vi "BIMS_Collector.vi"() -> ()   [LabVIEW 2015]
doc: "This program is currently beta software. It is designed to address the data requirements defined primarily by the DHB Ballistic Test Report.\n\nThe general operation of this program is based on the Ballistics Version 2005 application developed internally by DuPont as a research tool for the Spruance Plant Ballistics Lab in Richmond, VA.\n\nPlease note that the original trigger control logic was modified and no longer depends on a safety interlock system to enable operation of a ballistic test.\n\nDuPont makes no warranties and assumes no liabilities in connection with any use of this program."
uses:
  DataSource.ctl
  shotsArr.ctl
  Shot Record.ctl
  Collector State.ctl
  <vilib>/Utility/error.llb/DialogType.ctl
  <vilib>/registry/registry.llb/Registry RtKey.ctl
  <vilib>/DAQmx/read.llb/DAQmx Read (Counter DBL 1Chan 1Samp).vi
  BIMS_Collector Globals.vi
  <vilib>/Utility/config.llb/Write Key (String).vi
  <vilib>/addons/database/Connection.llb/DB Tools Open Connec (Path).vi
  <vilib>/addons/database/Connection.llb/Conn Execute.vi
  <vilib>/addons/database/Recordset.llb/Rec Destroy - Connection.vi
  <vilib>/DAQmx/miscellaneous.llb/DAQmx Fill In Error Info.vi
  <vilib>/addons/database/NI_Database_API.lvlib
  <vilib>/Utility/config.llb/NI_LVConfig.lvlib
  <vilib>/Utility/file.llb/Write To Spreadsheet File (string).vi
panel:
  in  "diagPageVisible":bool
  in  "runtimeMenusVisible":bool=TRUE
  out "loadStatus":string
  out "Loading":u16(ring)
  in  "RESET All":bool
  out "ConfigName":string
  out "TimeNow":string
  in  "EXIT":bool
  in  "mainTabCntrl":enum32{"Setup", "Measure", "History", "System"}(tab)=enum."System"
  in  "SampleEntryTabCntrl":enum32{"Environment", "Sample"}(tab)
  in  "ThreatDetails":u16(ring) caption="Detail"
  in  "ThreatGroups":u16(ring) caption="Group" items=["", "RCC", "FSP", "44 Magnum", "0.22 Caliber", "0.380 Caliber", "0.38 Caliber", "9mm Luger", "40 S&W", "0.357 MAG", "0.44 Expp Mag", ".44 SWC Gas Checked", ".44 SJHP", ".357 SIG", "7.62 AP", "7.62 Comum", "5.56 AP", "5.56 Comum", "0.44 Rem Mag"]
  in  "PowderTypes":u16(ring) caption="Type" items=["", "CBC 236", "CBC 210", "CBC 220", "CBC 216", "CBC 207", "CBC PCL 504", "CBC 102"]
  in  "Ballisticians":u16(ring) caption="Laboratorists" items=["", "Gustavo M Rubio", "Manoel Machado", "Outros (others)", "Renato Dantas"]
  in  "Recorders":u16(ring) caption="Recorder"
  in  "Shooters":u16(ring) caption="Shooter" items=["", "Manoel C. Machado                                 ", "Gustavo M Rubio                                   ", "Assef Maluf                                       "]
  in  "Methods":u16(ring) caption="Method" items=["", "V50", "NIJ 0101.04", "NIJ 0101.06", "NIJ 0108.01", "Helmets", "Others"]
  in  "RoomT":sgl caption="Temperature (° C)" format="%.1f"
  in  "RoomHum":sgl caption="Humidity (%)" min=0 max=100 format="%.1f"
  in  "SampleBackings":u16(ring)=3 caption="Type" items=["", "Clay", "Roma Clay", "Corfix Clay", "Dim Clay"]
  in  "clayCalArray":i16[](array[numeric])=[0, 0, 0, 0, 0] caption="Calibration (mm)" min=0 max=99 format="%02.0f"
  out "clayAverage":sgl caption="Clay Average (mm)" format="%#.1f"
  in  "clayTemp":sgl caption="Clay Temp (° F)" format="%.1f"
  out "threatDetails":T1 caption="Description"
  in  "SampleClamping":u16(ring) caption="Clamping" items=["", "elástic with Velcro", "screws", "rubber tube", "anti spall ", "box against fragments"]
  in  "Sample SubTabCntrl":T2(tab)
  in  "SampleID":string caption="Sample ID"
  in  "SampleDimensions":u16(ring) caption="Dimensions" items=["", "40 x 40", "50 x 50", "P", "M", "G", "GG", "Car Part", "Indefinite"]
  in  "ModelMfrs":u16(ring) caption="Manufacturer" items=["DuPont Experimental"]
  in  "SampleTypes":u16(ring) caption="Sample Type" items=["", "Aramid", "Glass", "Steel", "Ceramic", "Panel", "Body Armor", "Car Parts", "Quality Control", "Helmets", "Shield", "Other"]
  in  "Submitters":u16(ring) caption="Submitter" items=["", "Ana P Viegas", "Julio Tabegna", "Priscila Akiti", "Ariana Bottura", "Carlos Magno", "Rodrigo Gomez", "Angela C Vargas", "Manoel Machado", "Others", "Marcelo Fonseca", "Rosa Buono", "Mayara Guimarães", "Katia Hamada", "Lucas Loureiro"]
  in  "ProjectID":string caption="Project ID"
  in  "BackLayers":i32 caption="# of Layers" min=0 max=99 step=5
  in  "FrontLayers":i32 caption="# of Layers" min=0 max=99 step=5
  in  "BackLayer":u16(ring) caption="Back Layer" items=["", "PC", "Steel", "PE Foam", "Ghost", "ceramic plate", "Others"]
  in  "FrontLayer":u16(ring) caption="Front Layer" items=["", "PC", "Steel", "PE Foam", "Ghost", "ceramic plate", "Others"]
  out "totalNumLayers":i32 caption="Total # of Layers" min=0 max=100 step=5
  out "totalBAW":sgl caption="Total BAW (psf)" format="%.2f"
  in  "LayerTabControl":enum32{"1", "2", "3", "4", "5", "6"}(tab) caption="Inner Layers"
  out "fab1_totalWt":sgl caption="Fab1 Wt" min=0 max=99 step=5 format="%.2f"
  out "SampleAttribs_1":T3 caption="fabricAttribs_1"
  in  "Layer_1":T4 caption="Fabric #1" {"plyNum" min=0}
  in  "SampleStyle_1":u16(ring) items=["", "S 5200 GR", "S 623 GR", "S 758 Prepeg", "S363 GR", "S363 WR", "S436 GR", "S436 WR", "S704 GR", "S704 WR", "S706WRH", "S708 GR", "S708 WR", "S720", "S720 GR", "S720 WR", "S724 GR", "S729 GR", "S729 WR", "S731 GR", "S731 WR", "S745 BKT", "S745 BKT 20", "S745 GR", "S745 H", "S745 WR", "S745GR-1", "S754 GR", "S778 GR", "S778 WR", "S779GR", "S779WR", "XF", "XP1000"]
  in  "Mfr_1":u16(ring) caption="vendor" items=["", "AGP", "Assef Maluf", "DuPont", "DuPont Cooper River", "DuPont do Brasil", "TEADIT", "TestBob1"]
  in  "layerStitch_1":u16(ring) caption="Stitch" items=["", "1-inch quilt", "2-inch quilt", "Corners Bartack", "Corners", "Custom (Panel)", "Custom (Vest)", "Diamond", "Edge", "n/a", "Normal"]
  out "fab2_totalWt":sgl caption="Fab2 Wt" min=0 max=99 step=5 format="%.2f"
  out "SampleAttribs_2":T3 caption="fabricAttribs_2"
  in  "Layer_2":T4 caption="Fabric #2" {"plyNum" min=0}
  in  "SampleStyle_2":u16(ring)
  in  "Mfr_2":u16(ring) caption="vendor" items=["", "AGP", "Assef Maluf", "DuPont", "DuPont Cooper River", "DuPont do Brasil", "TEADIT", "TestBob1"]
  in  "layerStitch_2":u16(ring) caption="Stitch" items=["", "1-inch quilt", "2-inch quilt", "Corners Bartack", "Corners", "Custom (Panel)", "Custom (Vest)", "Diamond", "Edge", "n/a", "Normal"]
  out "fab3_totalWt":sgl caption="Fab3 Wt" min=0 max=99 step=5 format="%.2f"
  out "SampleAttribs_3":T3 caption="fabricAttribs_3"
  in  "Layer_3":T4 caption="Fabric #3" {"plyNum" min=0}
  in  "SampleStyle_3":u16(ring)
  in  "Mfr_3":u16(ring) caption="vendor" items=["", "AGP", "Assef Maluf", "DuPont", "DuPont Cooper River", "DuPont do Brasil", "TEADIT", "TestBob1"]
  in  "layerStitch_3":u16(ring) caption="Stitch" items=["", "1-inch quilt", "2-inch quilt", "Corners Bartack", "Corners", "Custom (Panel)", "Custom (Vest)", "Diamond", "Edge", "n/a", "Normal"]
  out "fab4_totalWt":sgl caption="Fab4 Wt" min=0 max=99 step=5 format="%.2f"
  out "SampleAttribs_4":T3 caption="fabricAttribs_4"
  in  "Layer_4":T4 caption="Fabric #4" {"plyNum" min=0}
  in  "SampleStyle_4":u16(ring)
  in  "Mfr_4":u16(ring) caption="vendor" items=["", "AGP", "Assef Maluf", "DuPont", "DuPont Cooper River", "DuPont do Brasil", "TEADIT", "TestBob1"]
  in  "layerStitch_4":u16(ring) caption="Stitch" items=["", "1-inch quilt", "2-inch quilt", "Corners Bartack", "Corners", "Custom (Panel)", "Custom (Vest)", "Diamond", "Edge", "n/a", "Normal"]
  out "fab5_totalWt":sgl caption="Fab5 Wt" min=0 max=99 step=5 format="%.2f"
  out "SampleAttribs_5":T3 caption="fabricAttribs_5"
  in  "Layer_5":T4 caption="Fabric #5" {"plyNum" min=0}
  in  "SampleStyle_5":u16(ring)
  in  "Mfr_5":u16(ring) caption="vendor" items=["", "AGP", "Assef Maluf", "DuPont", "DuPont Cooper River", "DuPont do Brasil", "TEADIT", "TestBob1"]
  in  "layerStitch_5":u16(ring) caption="Stitch" items=["", "1-inch quilt", "2-inch quilt", "Corners Bartack", "Corners", "Custom (Panel)", "Custom (Vest)", "Diamond", "Edge", "n/a", "Normal"]
  out "fab6_totalWt":sgl caption="Fab6 Wt" min=0 max=99 step=5 format="%.2f"
  out "SampleAttribs_6":T3 caption="fabricAttribs_6"
  in  "Layer_6":T4 caption="Fabric #6" {"plyNum" min=0}
  in  "SampleStyle_6":u16(ring)
  in  "Mfr_6":u16(ring) caption="vendor" items=["", "AGP", "Assef Maluf", "DuPont", "DuPont Cooper River", "DuPont do Brasil", "TEADIT", "TestBob1"]
  in  "layerStitch_6":u16(ring) caption="Stitch" items=["", "1-inch quilt", "2-inch quilt", "Corners Bartack", "Corners", "Custom (Panel)", "Custom (Vest)", "Diamond", "Edge", "n/a", "Normal"]
  in  "SampleCoverings":u16(ring) caption="Sample Covering" items=["None", "RipStop", "Plastic bag", "Other"]
  in  "Assemblers":u16(ring) caption="Technician" items=["", "Gustavo M Rubio", "Lucas Loureiro", "Manoel Machado", "Assef Maluf", "Client", "Tecidos Especiales", "Others"]
  in  "Thickness":dbl caption="Thickness (mm)" format="%.3f"
  in  "totalSampleWt":sgl caption="Total Weight (g)" format="%.3f"
  in  "Comments":string caption="Remarks (optional):"
  in  "TestConditions":u16(ring) caption="Sample Condition" items=["", "Dry", "Wet", "T & H Controlled", "After Tumbling", "Heated", "Cooled"]
  in  "shotsTabCntrl":T5(tab)
  in  "2ndScreen":bool=TRUE caption="Enabled"
  out "cntDn":i32
  in  "Frag Rod":sgl format="%.1f"
  in  "Drag Corrected":bool=TRUE
  out "Impact/speed":sgl caption="Chronograph 1" min=0 max=10000 step=0.1 format="%.1f"
  out "residual/speed":sgl caption="Residual" min=0 max=10000 step=0.1 format="%.1f"
  in  "MeasVelScrnSet1":sgl caption="Set #1" min=0 max=10000 step=0.1 format="%.1f"
  in  "Current/shotstatus":u16(ring) caption="Penetration" items=["Partial", "Complete"]
  in  "Current/residual/speed":sgl caption="Residual Set" min=0 max=10000 step=0.1 format="%.1f"
  in  "shotTimestamp":string caption="Date/Time"
  in  "MeasVelScrnSet2":sgl caption="Set #2" min=0 max=1000000 step=0.1 format="%.1f"
  out "%_Difference":sgl caption="% Vel Diff" format="%.3f"
  in  "backdepth":sgl caption="BF Depth"
  out "Redundant/speed":sgl caption="Chronograph 2" min=0 max=10000 step=0.1 format="%.1f"
  out "Current/avg/speed":sgl caption="Average" min=0 max=1000000 step=0.1 format="%.1f"
  out "Avg/speed":sgl caption="Average" min=0 max=10000 step=0.1 format="%.1f"
  out "DC_ factor":sgl=1.0 caption="DC Factor" format="%.4f"
  in  "Barrel Temp":sgl format="%.1f"
  in  "Shot Description":string caption="Description (optional)"
  in  "Powder Loading":sgl caption="Powder Load" min=0 max=100 step=0.1 format="%.3f"
  in  "Shot Angle":u16 max=90 step=1
  out "Projectile Mass":sgl caption="Projectile Mass (grains)" min=0 step=1
  in  "N.I.J":u16(ring) items=["n/a", "PASS", "FAIL"]
  in  "addShot":bool caption="RANGE SETUP must be selected before shots can be added."
  in  "loadingUnits":enum32{"grams", "grains"}(radio)
  out "instruct_addShot":string="RANGE SETUP and THREAT must be selected before shots can be added."
  out "Set#1 Separation":sgl=1.0 caption="Outer" format="%.2f"
  out "Set#2 Separation":sgl=1.0 caption="Inner" format="%.2f"
  out "ARMED":bool caption="Armed"
  in  "commercialReport":bool caption="Report"
  out "velSTDEV":sgl caption="Standard Deviation" min=0 max=10000 step=1 format="%.1f"
  out "saveReq":string="Number of layers in sample ply specification and number of shots in shots table must be greater than 0 to enable saving."
  out "Table of Shots":string[][](table) caption="Shot Table"
  in  "MC Listbox of Shots":i32(listbox)
  in  "saveShots":bool
  in  "clearShots":bool
  out "highPartial":i32 caption="High Partial" min=0 max=10000 step=1
  out "lowComplete":i32 caption="Low Complete" min=0 max=10000 step=1
  out "rangeOfResults":i32 caption="Range of Results" min=0 max=10000 step=1
  out "zmr 2":sgl caption="ZMR" format="%.1f"
  out "computed_V50":sgl caption="V50  (m/s)" format="%.1f"
  out "Pairs":i16 min=0 max=100 step=1
  in  "reportV50":bool caption="Report"
  in  "maxDev":sgl=10.0 caption="Max Deviation (m/s)" min=0 max=100 format="%.1f"
  in  "undoLastShot":bool
  in  "reportType":enum32{"V50", "NIJ"}(radio)
  in  "language":enum16{"Spanish", "Portuguese", "English"}(ring)
  in  "deleteShot":bool
  in  "nextShot":bool
  in  "shotsArr":T6 {"Frag Rod" format="%.1f"; "UncorrectedAvgVel_PB" format="%.1f"; "UncorrectedRed_PB" format="%.1f"; "strikeVel_PB" format="%.1f"; "velLoss_PB" format="%.1f"; "avgVel_PB" format="%.1f"; "Redundant_Velocity" format="%.1f"; "Energy Loss (J)" format="%.3e"; "Projectile Mass" min=0 step=1 format="%.4f"; "Corrected residual" format="%.2f"; "Uncorrected Residual" format="%.1f"; "Corrected Impact" format="%.2f"; "Uncorrected Impact" format="%.1f"; "Shot Angle" max=90 step=1; "SHOT STATUS" items=["Partial", "Complete"]; "IMPACT VELOCITY" min=0 max=10000 step=0.1 format="%.1f"; "Barrel Temperature" format="%.1f"; "Powder Loading" format="%.4f"; "RESIDUAL  VELOCITY" min=0 max=10000 step=0.1 format="%.1f"}
  out "velProfile":cluster{dbl, dbl}[](graph) caption="Shot Velocity Measurement Profile"
  out "velCompProf":cluster{"vStrike":dbl, "vA":dbl} caption="Velocity in fps\n(computed)"
  out "velMeasProf":T8 caption="Velocity in fps\n(measured)"
  out "relativeTime":cluster{"ts2":dbl, "ts3":dbl, "ts1":dbl} caption="Relative time\n(microsec)"
  out "displacement":T9={"ds_v2"=6.75, "ds2"=5.0833, "ds_vB"=4.9167, "ds3"=4.75, "ds_vAvg"=6.9167, "ds_v1"=7.0833, "ds1"=8.75, "ds_vA"=8.9167, "ds0"=9.0833} caption="Distance from\ntarget (ft)" {"ds0" format="%_4g"; "ds_vA" format="%_4g"; "ds1" format="%_4g"; "ds_v1" format="%_4g"; "ds_vAvg" format="%_4g"; "ds3" format="%_4g"; "ds_vB" format="%#_4g"; "ds2" format="%#_4g"; "ds_v2" format="%_4g"}
  out "arrIDC":dbl[](array[numeric]) caption="Instantaneous Drag Coefficient"
  in  "rangeSetup":u16(ring)=1 caption="Range Dimensions" items=["Short (small frag)", "Standard (handgun)", "Long (rifle)"]
  out "mid_to_targ_dist":sgl=5.0 caption="Mid To Target (ft)"
  in  "historyTabCntrl":enum32{"Powder Loading", "Panel Search"}(tab)=enum."Panel Search"
  in  "Threat.freeTxt":string caption="Threat"
  in  "Powder.freeTxt":string caption="Powder"
  in  "QueryLoad":bool
  in  "lkupEndDate":timestamp caption="End Date" format="%<%x>T"
  in  "lkupStartDate":timestamp caption="Begin Date" format="%<%x>T"
  out "Vel.vs.Loading":cluster{dbl[], dbl[]}(graph)
  out "v50_table":string[][](table)
  in  "maxRecs":u16=1001 caption="Max # of SHOT Records" min=1 max=10000 step=100
  out "ActualNumRecs":i32=1001 caption="Actual # Returned"
  in  "appendPrjs":bool caption="merge projects"
  in  "prjAll":bool
  in  "prjV50Rpt":bool
  in  "prjSelect":bool[](array[boolean])
  in  "ProjectID_0":u16(ring) caption="Project ID"
  in  "ThreatSize_0":u16(ring) caption="Threat Size" items=["", "2", "4", "16", "17", "33", "40", "44", "55", "61", "85", "95", "124", "125", "138", "147", "158", "180", "240"]
  in  "panelSearch":bool
  in  "Mfr_0":u16(ring) caption="Manufacturer" items=["", "AGP", "Assef Maluf", "DuPont", "DuPont Cooper River", "DuPont do Brasil", "TEADIT", "TestBob1"]
  in  "SampleStyle_0":u16(ring) caption="Sample Style"
  in  "srchParams":T10={"maxPanels"=1001, "lkupPanelStartDate"=timestamp(0 s since 1904-01-01), "lkupPanelEndDate"=timestamp(3552315047.0950403 s since 1904-01-01)} {"lkupPanelEndDate" format="%<%x>T"; "lkupPanelStartDate" format="%<%x>T"; "maxPanels" min=1 max=10000 step=100}
  out "actualNumPanels":i32 caption="Actual # Returned"
  out "pastPanels":string[][](table)
  in  "Record #":i32=1 min=0 max=3199
  in  "reportV50_History":bool
  out "SampleAttribs_0":T11 caption="fabricAttribs_1"
  in  "Requestors_0":u16(ring) caption="Submitter" items=["", "Ana P Viegas", "Angela C Vargas", "Ariana Bottura", "Carlos Magno", "Julio Tabegna", "Katia Hamada", "Lucas Loureiro", "Manoel Machado", "Marcelo Fonseca", "Mayara Guimarães", "Others", "Priscila Akiti", "Rodrigo Gomez", "Rosa Buono"]
  in  "aboutTabCntrl":T12(tab)
  in  "RefreshMetadata":bool
  out "lastShot":i32 caption="Shot"
  out "lastSamp":i32 caption="Sample"
  in  "PublishNewRecords":bool
  in  "btnScrnSets":bool caption="Update Screen Sets"
  in  "screenSet_1":sgl caption="Outer" format="%.2f"
  in  "screenSet_2":sgl caption="Inner" format="%.2f"
  in  "internal":enum32{"ctr", "deploy", "misc"}(tab)=enum."misc"
  out "taskCtr1":refnum<k21>
  in  "ctr1":tag="LightScreens/ctr1"
  in  "readyClock":bool caption="Clock"
  in  "ActiveDev":tag="LightScreens"
  in  "ctr0":tag="LightScreens/ctr0"
  in  "SampClk.Timebase.Src":tag="/LightScreens/80MHzTimebase"
  out "Device S/N":string
  in  "MeasSrc":T13=enum."Screens" caption="Source"
  in  "ARM":bool
  out "errCtr0":errorcluster
  out "errCtr1":errorcluster
  out "taskCtr0":refnum<k21>
  in  "Folder":string caption="Publish Folder"
  in  "useBMC":bool caption="Use Message Center?"
  in  "Server":string
  in  "Site":string
  in  "InterlockExists":bool=TRUE caption="Safety Interlock Hardware Exist?"
  in  "ScreenSetAvgg":bool=TRUE caption="Average Screen Sets?"
  in  "Sort by AVG":bool=TRUE caption="Sort shots by average velocity"
  in  "useBallisitican":bool=TRUE caption="Use Ballistician field in Setup?"
  in  "useRecorder":bool caption="Use Recorder field in Setup?"
  in  "useShooter":bool caption="Use Shooter field in Setup?"
  in  "close arming loop":bool
  out "progState":T14
  in  "clearErrors":bool
  in  "LayerStitchTypes":u16(ring) caption="Stitch" items=["", "1-inch quilt", "2-inch quilt", "Corners Bartack", "Corners", "Custom (Panel)", "Custom (Vest)", "Diamond", "Edge", "n/a", "Normal"]
  out "GrainSize":u16 caption="Grain"
  out "U/I EvErr":errorcluster
  out "SMErr":errorcluster
  in  "Models":u16(ring) caption="Model #" items=["n/a"]
  in  "serialNum":string caption="Serial #"
  in  "SampleDescrip":u16(ring) caption="Misc. Sample Description (legacy)"
  out "lengthUnits":string="FOOT" caption="Distance Units"
  out "massUnits":string="GRAMS" caption="Weight Units"
  in  "Threat":u16(ring) caption="Threat (long description)"
  in  "Type of work":string="QC"
  in  "minV50":i32=1500 caption="Minimum V50"
  out "configPath":path=path "P:/Private/My Projects/AFS/BIMS/2008/BIMS_Collector.ini" caption="Configuration Path (INI)"
  out "STOP (Shots MC LB)":bool=TRUE
  in  "lookupRec":bool caption="lookup"
  in  "clayCalib":string="##-##-##-##-##" caption="Calibration"
  in  "Fabric Description":string caption="Fabric Desc"
  in  "Areal density text":string
  in  "Areal Density":dbl format="%.2f"
  out "Residual factor":sgl=1.0 caption="Residual" min=0 max=1 format="%.5f"
  out "Impact factor":sgl=1.0 caption="Impact" min=0 max=1 format="%.5f"
  out "Partial":sgl[](array[numeric]) format="%.2f"
  out "factor array":sgl[](array[numeric]) format="%.4f"
  out "Complete":sgl[](array[numeric]) format="%.2f"
  in  "old threat":u16
  out "Z.M.R.":sgl min=0 step=0.1 format="%.1f"
  in  "Residual/Target Dist":sgl=7.083333 format="%.2f"
  out "Residual/Separation":sgl=4.0 format="%.2f"
  in  "Set#1_to_Target":sgl=7.083333 format="%.2f"
  out "Barrel to Screen":sgl=7.8333 format="%.2f"
  out "CorrectedVelScrnSet1":sgl=1503.981 format="%.2f"
  out "Corrected Residual":sgl=751.9905 format="%.2f"
  out "correction coefficient":sgl format="%.8f"
  in  "SoftwareVersion":dbl caption="Version" format="%.2f"
  in  "percent warning":sgl=1.0 format="%.2f"
  out "#_partials":i32
  out "#_completes":i32
  out "conversion factor":sgl=0.3048037 format="%.5f"
  out "CorrectedVelScrnSet2":sgl=1551.8816 caption="Corrected Redundant" format="%.2f"
  out "Corrected Average":sgl=1527.9313 format="%.2f"
  in  "processShots":bool caption="Proc Shots"
  in  "WeaponTypes":u16(ring) caption="Weapon" items=["", "Universal Receiver", "Other"]
  in  "TestStandards":u16(ring)=2 caption="Standard" items=["n/a", "NIJ 0101.04", "MIL-STD-662F"]
  out "SUBMIT DATE/TIME":string
  in  "VsVr Report":bool caption="Report"
  # "Effectively restarts the application from scratch, as if the user pressed the EXIT button and then restarted the application."
  # "Configured for"
  # "Threat"
  # "*"
  # "*"
  # "Test"
  # "Powder"
  # "*"
  # "Personnel"
  # "Room"
  # "*"
  # "Backing"
  # "*"
  # "*"
  # "*"
  # "Strike Face"
  # "Body Side"
  # "Layer"
  # "Mfr"
  # "Style"
  # "# of Plies"
  # "Lot"
  # "Roll"
  # "Stitch"
  # "Internal ID"
  # "Fiber"
  # "Denier"
  # "Construction"
  # "Weave"
  # "Finish"
  # "Basis weight (oz/yd²)"
  # "Yarn Merge"
  # "Total Weight"
  # "*"
  # "*"
  # "*"
  # "1"
  # "2"
  # "3"
  # "4"
  # "5"
  # "6"
  # "Required"
  # "*"
  # "Shot Parameters"
  # "cm"
  # "deg"
  # "° C"
  # "Screens\nSeparation"
  # "meters"
  # "Velocity Measurements"
  # "Observations"
  # "Table Functions"
  # "Summary"
  # "Reports"
  # "Test Record"
  # "Edit Shot Records"
  # "Corrected"
  # "Shot #"
  # "t0"
  # "0"
  # "S Strike"
  # "0"
  # "Internal ID#"
  # "Fiber"
  # "Denier"
  # "Pick"
  # "Weave"
  # "Finish"
  # "oz/yd²"
  # "Asset"
  # "DuPont Protection Technologies\nBallistics Information Management System\n\nBIMS\n\n\nSample Performance\nData Collector\n\nSeptember 17, 2016"
  # "DuET Dynamic Simulation, Control, and Optimization\n+1 (302) 992-2010 for technical support"
  # "Last Assigned\nRecord Numbers"
  # "Screens\nSeparation"
  # "meters"
  # "Deployment Configuration"
  # "NI LabVIEW 2015 Ver 15.0.1f1 (32-bit)\nLast build on 06/23/2016"
  # "Correction Factors"
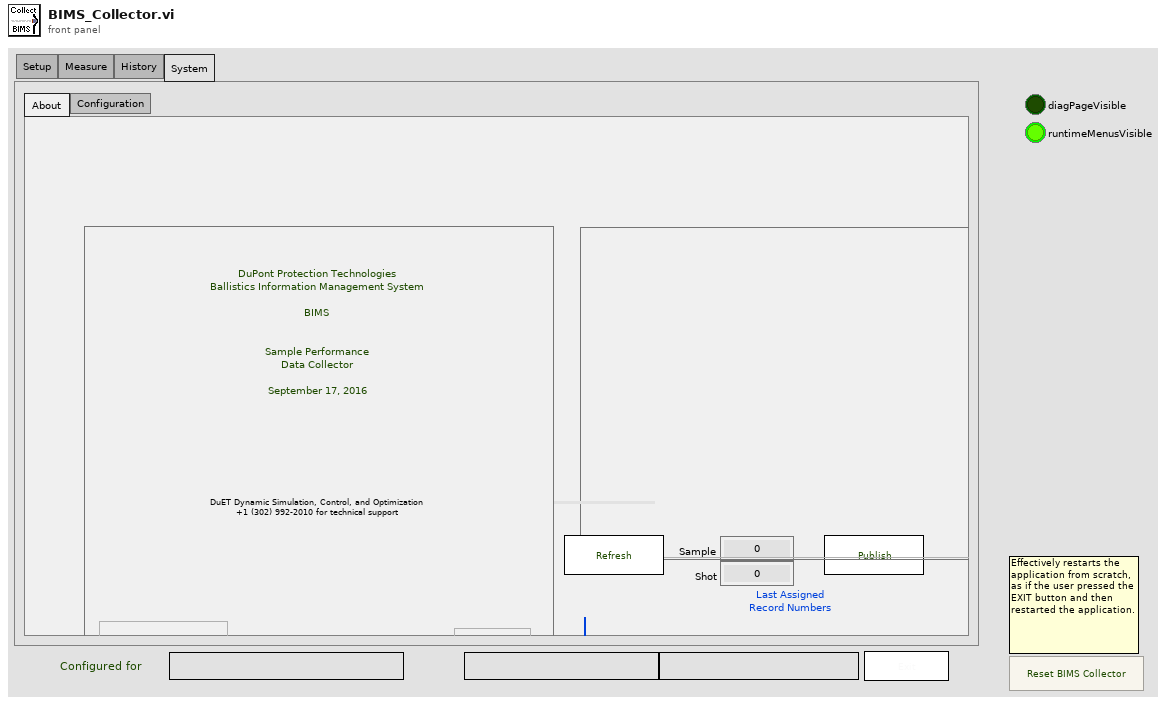
[diagram p1: front panel]
types:
  T1 = cluster{"barrelLength":string, "dragCorrection":string, "detailDescription":string, "barrelCaliber":string, "grainSize":string, "Make":string, "Model":string}
  T2 = enum32{"General Specification", "Ply Specification", "Preparation"}
  T3 = cluster{"Fabric.fiber":string, "Fabric.denier":string, "pick":string, "weave":string, "finish":string, "ozPerYd2":string, "fabricID_DHB":string, "yarnMerge":string}
  T4 = cluster{"plyNum":i32, "LotNum":string, "RollNum":string}
  T5 = enum32{"Ready-Aim-Fire", "Shots Table", "Edit", "Instantaneous DC"}
  T6 = typedef "shotsArr.ctl" = T7[]
  T7 = typedef "Shot Record.ctl" = cluster{"Uncorrected Impact":sgl, "Uncorrected Residual":sgl, "avgVel_PB":sgl, "IMPACT VELOCITY":sgl, "RESIDUAL  VELOCITY ":sgl, "Shot Description":string, "Powder Loading ":sgl, "Barrel Temperature":sgl, "TIME / DATE":string, "shot order":i32, "SHOT STATUS":u16, "Shot Angle":u16, "Corrected Impact":sgl, "Corrected residual":sgl, "Projectile Mass":sgl, "usedv50":bool, "Energy Loss (J)":sgl, "BackFace\nDepth":sgl, "BackFace\nDiameter":sgl, "Redundant_Velocity":sgl, "velLoss_PB":sgl, "strikeVel_PB":sgl, "UncorrectedRed_PB":sgl, "CorrectedRed_PB":sgl, "UncorrectedAvgVel_PB":sgl, "V50userExcl":bool, "Frag Rod":sgl, "fairHit":bool}
  T8 = cluster{"v2":dbl, "vB":dbl, "vOuter":dbl, "v1":dbl, "vA":dbl, "vInner":dbl}
  T9 = cluster{"ds_v2":dbl, "ds2":dbl, "ds_vB":dbl, "ds3":dbl, "ds_vAvg":dbl, "ds_v1":dbl, "ds1":dbl, "ds_vA":dbl, "ds0":dbl}
  T10 = cluster{"maxPanels":u16, "lkupPanelStartDate":timestamp, "lkupPanelEndDate":timestamp}
  T11 = cluster{"Fabric.fiber":string, "Fabric.denier":string, "pick":string, "weave":string, "finish":string, "ozPerYd2":string, "fabricID_DHB":string, "asset":string}
  T12 = enum32{"About ", "Configuration", "Internal Use"}
  T13 = typedef "DataSource.ctl" = enum16{"Simulated", "Radar", "Screens"}
  T14 = typedef "Collector State.ctl" = enum16{"POLL", "INITIALIZE", "V50 Report or GET Record", "VsVr Report", "SAVE SHOTS", "ADD SHOT", "CLEAR SHOTS", "NEXT SHOT", "DELETE SHOT", "READY CLOCK", "PROC SHOTS", "CHECK DAQ"}
  T15 = typedef "DialogType.ctl" = u16
  T16 = enum8{"Enabled", "Disabled", "Disabled and Grayed Out"}
  T17 = enum32{"Page Enabled", "Page Disabled", "Page Disabled & Grayed"}
  T18 = enum32{"invalid app kind", "Development System", "Run Time System", "Student Edition", "Embedded LabVIEW", "Evaluation", "Custom"}
  T19 = cluster{"Mfr_0":refnum<vi>, "SampleStyle_0":refnum<vi>, "pastPanels":refnum<vi>, "ProjectID_0":refnum<vi>}
  T20 = cluster{"clayAverage":string, "clayCalib":string, "maxBFD":string, "minBFD":string, "avgBFD":string, "bfdSTDEV":string}
  T21 = cluster{"V50":string, "highPartial":string, "lowComplete":string, "STDEV":string}
  T22 = cluster{"ProjectID":string, "Comments":string, "method":string, "Thickness":string, "SampleDimension":string, "numPlies":string, "PowderType":string, "SampleBacking":string, "totalSampleWt":string, "RoomHum":string, "RoomT":string, "grainSize":string, "threatGroup":string, "TestConditions":string, "Muzzel/Target":string, "Muzzel/Screen1":string, "Screen1/Screen2":string, "Screen2/Target":string, "Ballistician":string}
  T23 = cluster{"numOfPlies":i32, "LotNum":string, "RollNum":string}[]
  T24 = cluster{"numOfPlies":i32, "LotNum":string, "RollNum":string}
  T25 = typedef "LVRowAndColumnTypeDef.ctl" = cluster{"Row":i32, "Column":i32}
  T26 = typedef "LVRowAndColumnUnsignedTypeDef.ctl" = cluster{"Row":u32, "Column":u32}
  T27 = cluster{"barrelLength":string, "dragCoefficient":string, "detailDescription":string, "barrelCaliber":string, "grainSize":string, "Make":string, "Model":string}
  T28 = cluster{"fiber":string, "denier":string, "construction":string, "weave":string, "finish":string, "ozPerYd2":string, "fabricStyle_DHB":string, "yarnMerge":string}
  T29 = cluster{"fiber":string, "denier":string, "pick":string, "weave":string, "finish":string, "ozPerYd2":string, "internal_ID":string, "asset":string}[]
  T30 = cluster{"plyNum":i32, "LotNum":string, "RollNum":string}[]
  T31 = typedef "NI_LVConfig.lvlib/Config Data RefNum.ctl" = refnum<k1>
  T32 = typedef "Registry RtKey.ctl" = enum32{"HKEY_CLASSES_ROOT", "HKEY_CURRENT_USER", "HKEY_LOCAL_MACHINE", "HKEY_USERS", "HKEY_PERFORMANCE_DATA", "HKEY_CURRENT_CONFIG", "HKEY_DYN_DATA"}
  T33 = cluster{"[0]":string, "[1]":string, "[2]":string, "[3]":string, "[4]":string, "[5]":string, "[6]":string, "[7]":string, "[8]":string, "[9]":string}[]
  T34 = cluster{"[0]":string, "[1]":string, "[2]":string, "[3]":string, "[4]":string, "[5]":string, "[6]":string, "[7]":string, "[8]":string}[]
  T35 = cluster{"Fabric.fiber":string, "Fabric.denier":string, "pick":string, "weave":string, "finish":string, "ozPerYd2":string, "fabricID_DHB":string, "yarnMerge":string}[]
  T36 = cluster{"Uncorrected Impact":bool, "Uncorrected Residual":bool, "avgVel_PB":bool, "IMPACT VELOCITY":bool, "RESIDUAL  VELOCITY ":bool, "Shot Description":bool, "Powder Loading ":bool, "Barrel Temperature":bool, "TIME / DATE":bool, "shot order":bool, "SHOT STATUS":bool, "Shot Angle":bool, "Corrected Impact":bool, "Corrected residual":bool, "Projectile Mass":bool, "usedv50":bool, "Energy Loss (J)":bool, "BackFace\nDepth":bool, "BackFace\nDiameter":bool, "Redundant_Velocity":bool, "velLoss_PB":bool, "strikeVel_PB":bool, "UncorrectedRed_PB":bool, "CorrectedRed_PB":bool, "UncorrectedAvgVel_PB":bool, "V50userExcl":bool, "Frag Rod":bool, "fairHit":bool}
  T37 = cluster{"SampleTypes":refnum<vi>, "SampleDescrip":refnum<vi>}
  T38 = cluster{"max dev":sgl, "residual separation":sgl, "Set#1 Separation":sgl, "Set#2 Separation ":sgl, "impact target dist":sgl, "resid target dist":sgl, "barrel screen dist":sgl, "midpt_to_target_dist":sgl}
  T39 = cluster{"muzzle / target":string, "muzzle / scr#1":string, "Set#1 Separation":string, "scr#2 / target":string, "mid_to_targ_dist":string, string, string, string, "clayCalib":string, string}
  T40 = cluster{string, string, string, string, string, string, string}
  T41 = cluster{"SampleID":string, "element":string, "Type of work":string, "serialNum":string, "element":string, string, string, string, "element":string, string}
  T42 = cluster{"SampleID":string, "element":string, string, string, string, "element":string}
  T43 = cluster{"[0]":string, "[1]":string, "[2]":string, "[3]":string, "[4]":string, "[5]":string, "[6]":string, "[7]":string, "[8]":string, "[9]":string}
  T44 = cluster{"[0]":string, "[1]":string, "[2]":string, "[3]":string, "[4]":string, "[5]":string, "[6]":string, "[7]":string, "[8]":string}
  T45 = cluster{"element":string, "element":string, "grainSize":string, "element":string, "barrelLength":string, string, "element":string, "element":string, "element":string}
  T46 = cluster{"element":string, "grainSize":string, "element":string, "barrelLength":string, string, "element":string}
  T47 = cluster{string, string, string, string, string, string, string, string, "clayCalib":string, string}
  T48 = typedef "NI_Database_API.lvlib/Conn ObjectReference.ctl" = refnum<k1>
  T49 = typedef "NI_Database_API.lvlib/Rec ObjectReference.ctl" = refnum<k1>
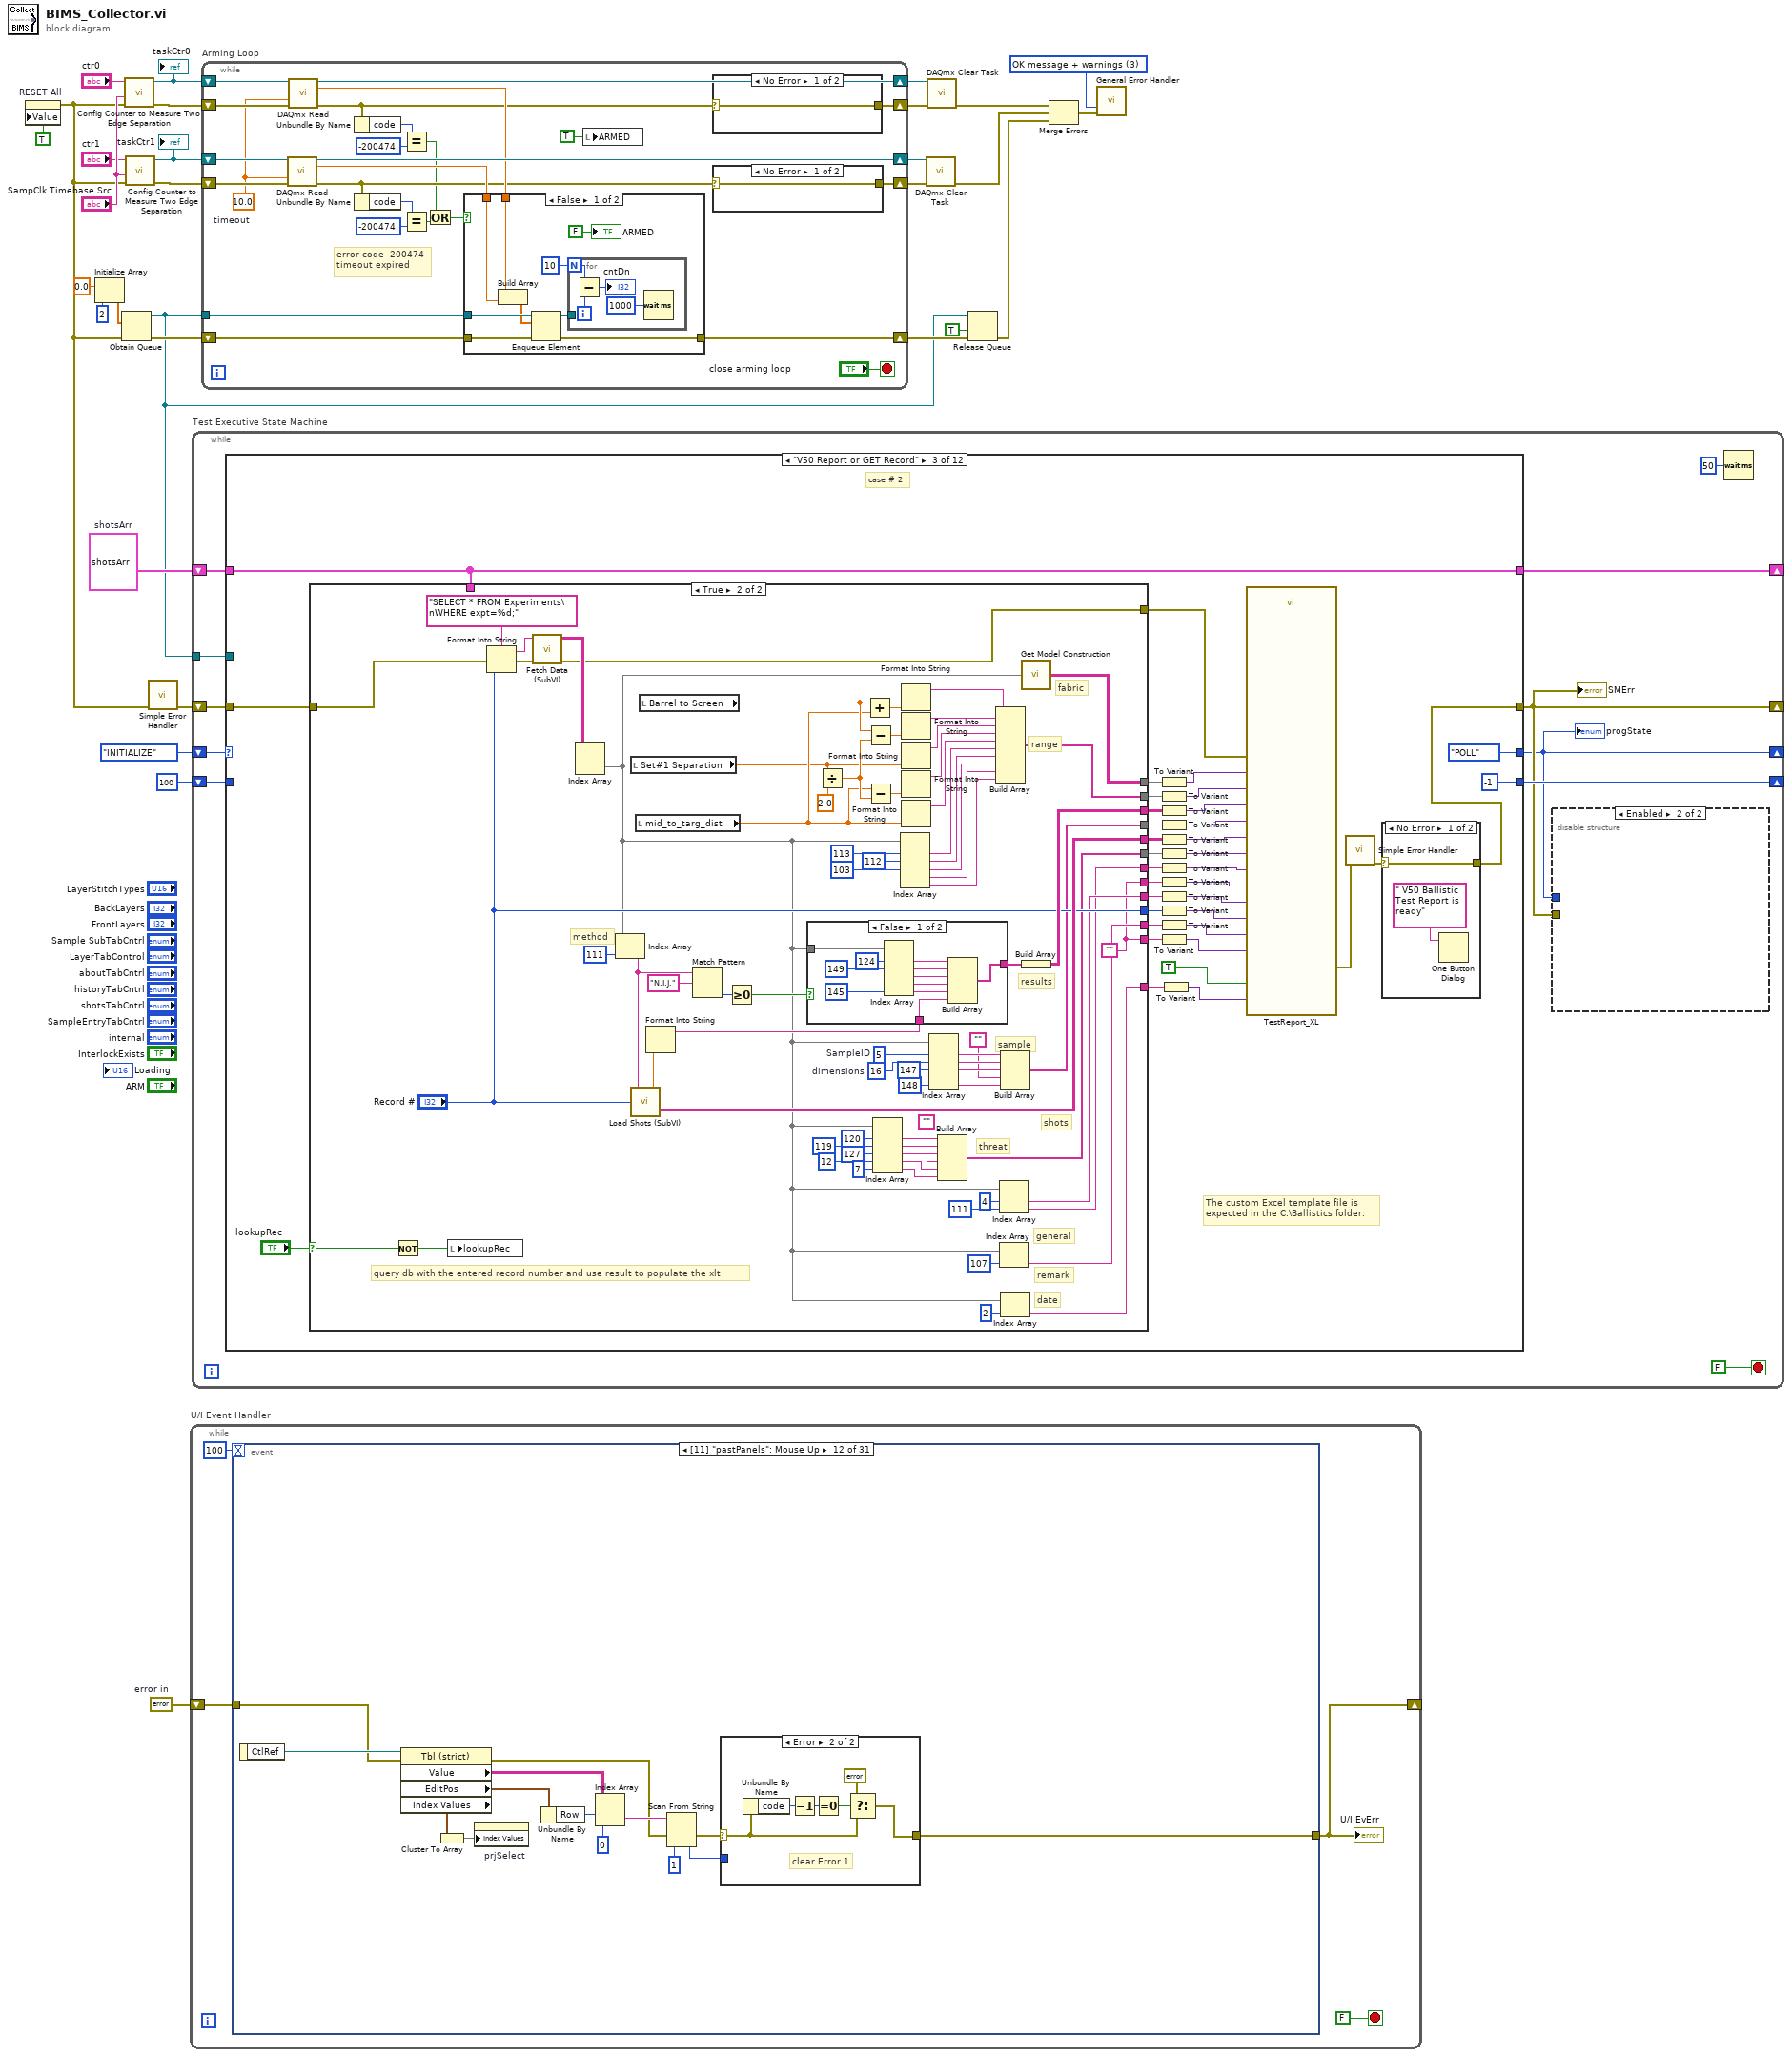
[diagram p0: block diagram]
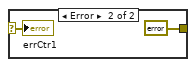
[diagram p3: hidden frame]
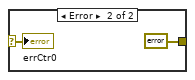
[diagram p4: hidden frame]
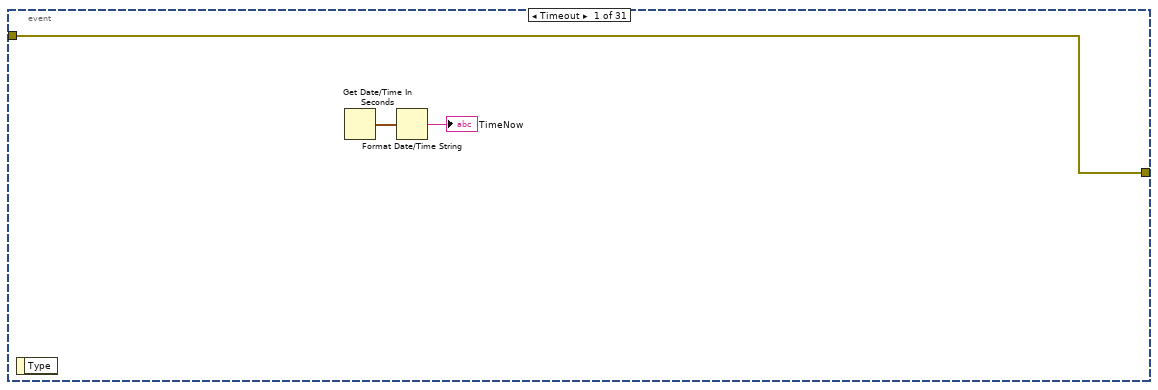
[diagram p5: hidden frame]
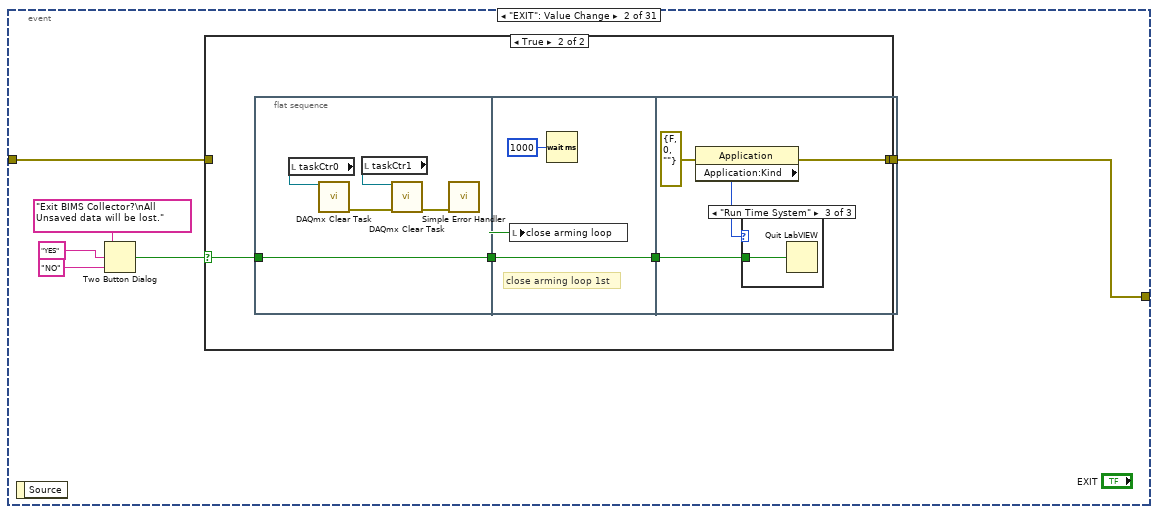
[diagram p6: hidden frame]
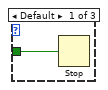
[diagram p8: hidden frame]
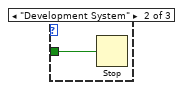
[diagram p9: hidden frame]
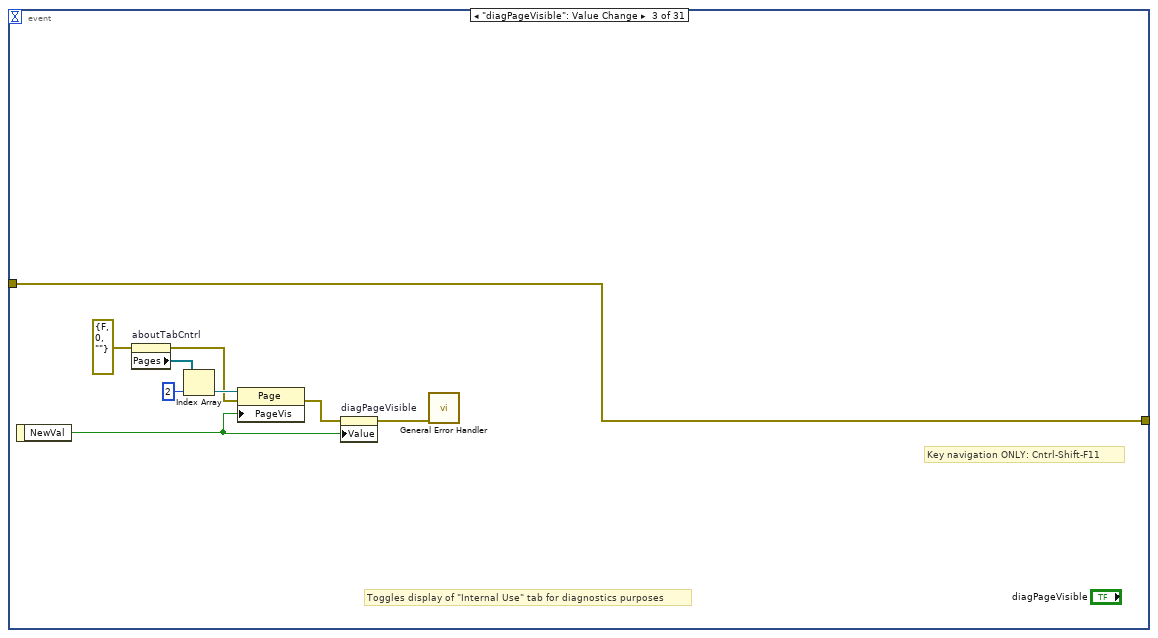
[diagram p10: hidden frame]
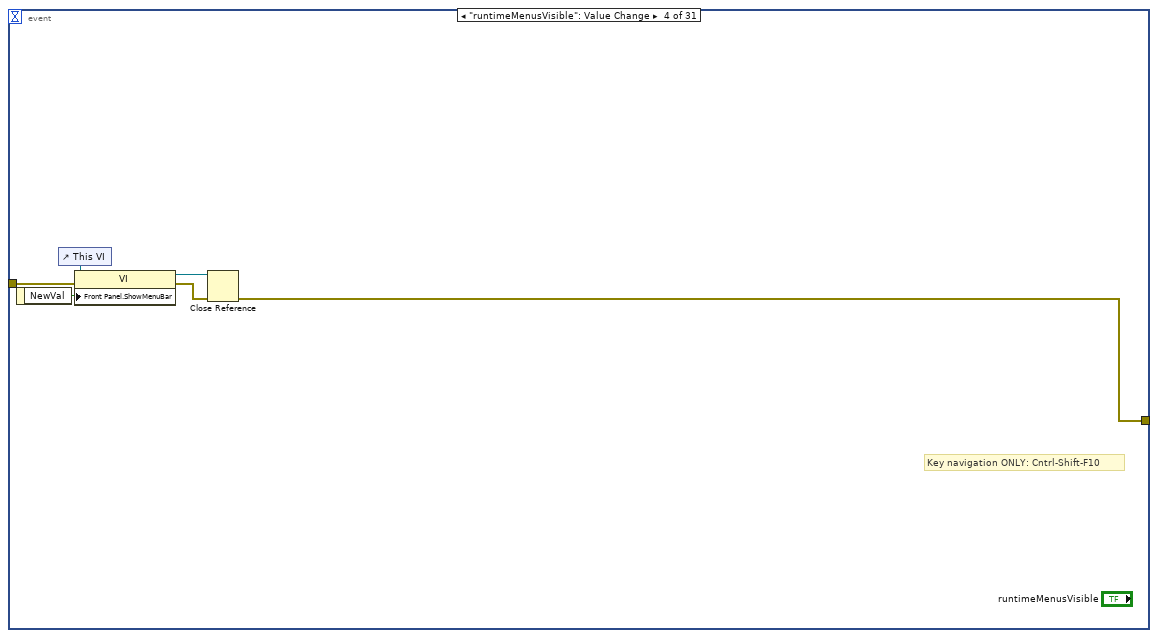
[diagram p11: hidden frame]
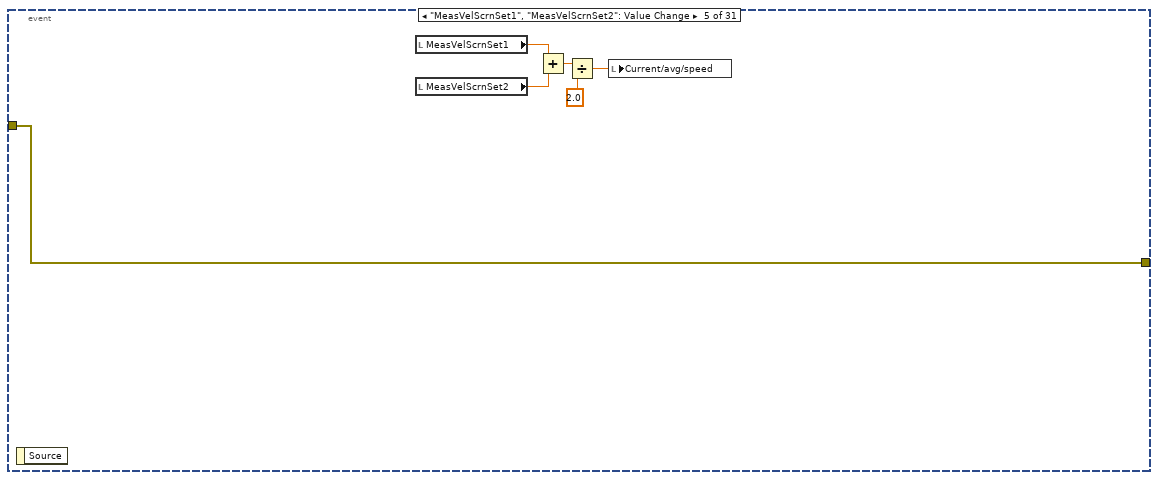
[diagram p12: hidden frame]
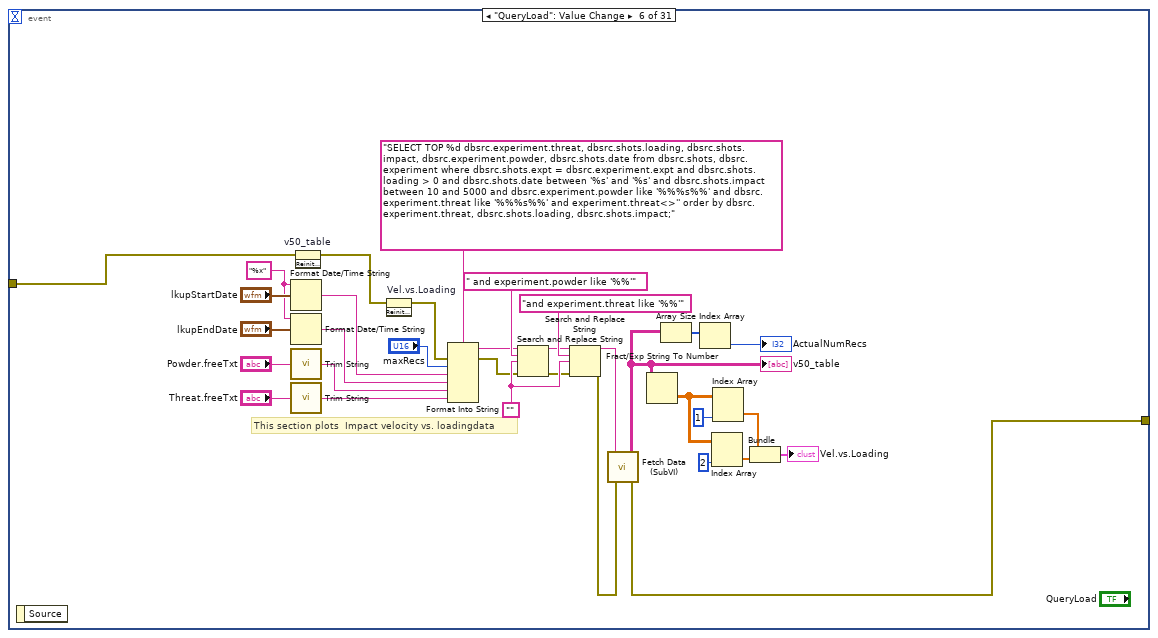
[diagram p13: hidden frame]
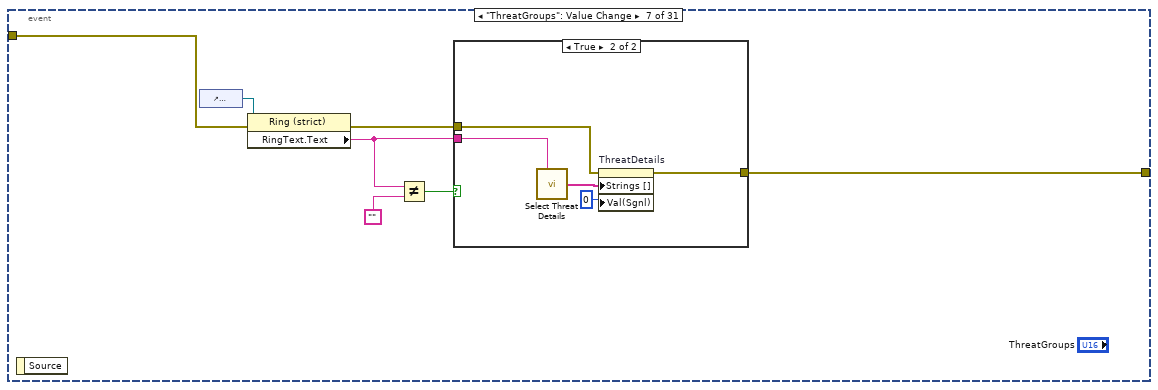
[diagram p14: hidden frame]
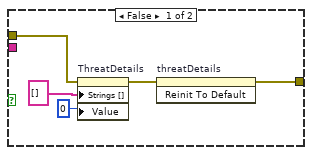
[diagram p15: hidden frame]
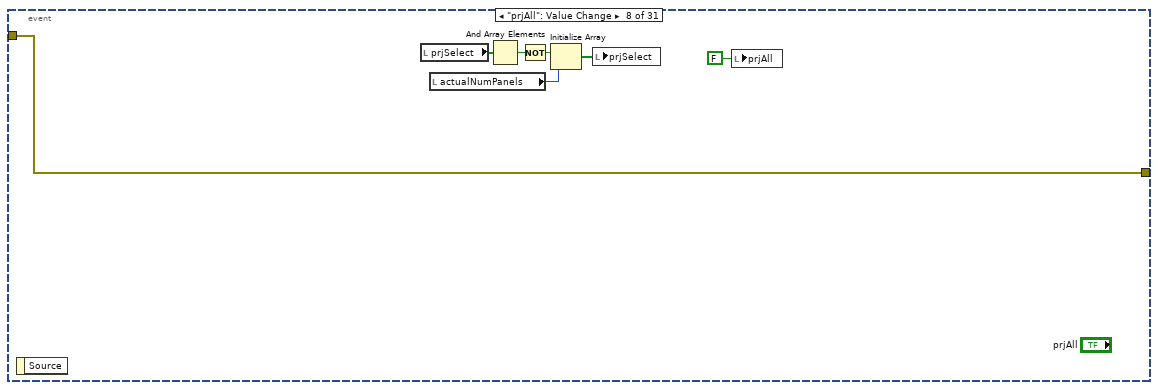
[diagram p16: hidden frame]
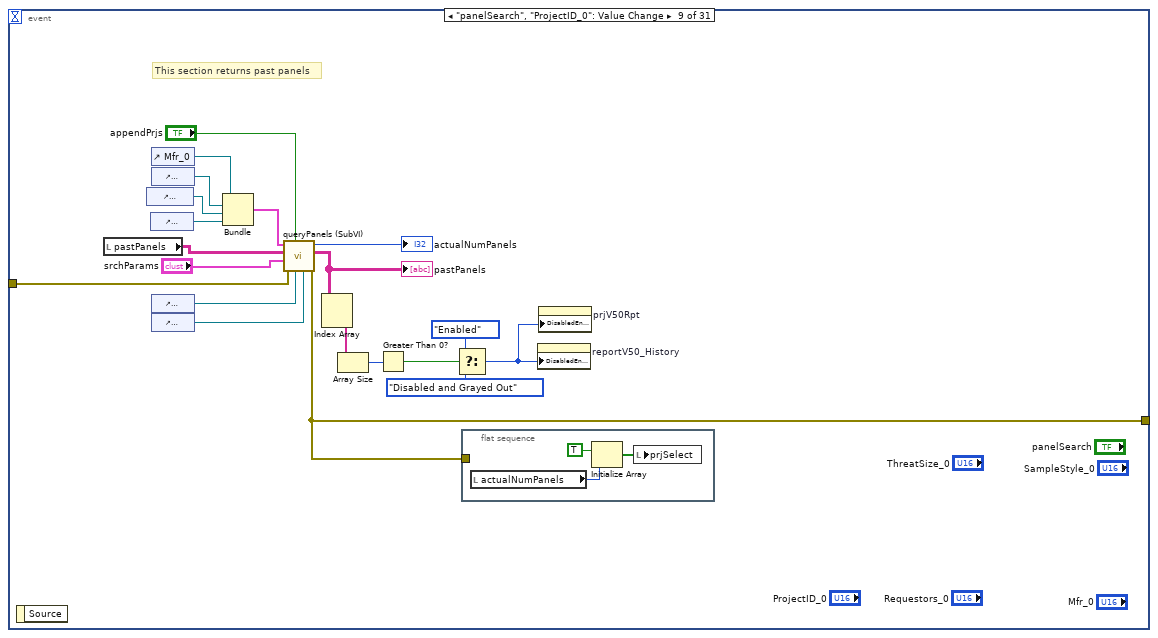
[diagram p17: hidden frame]
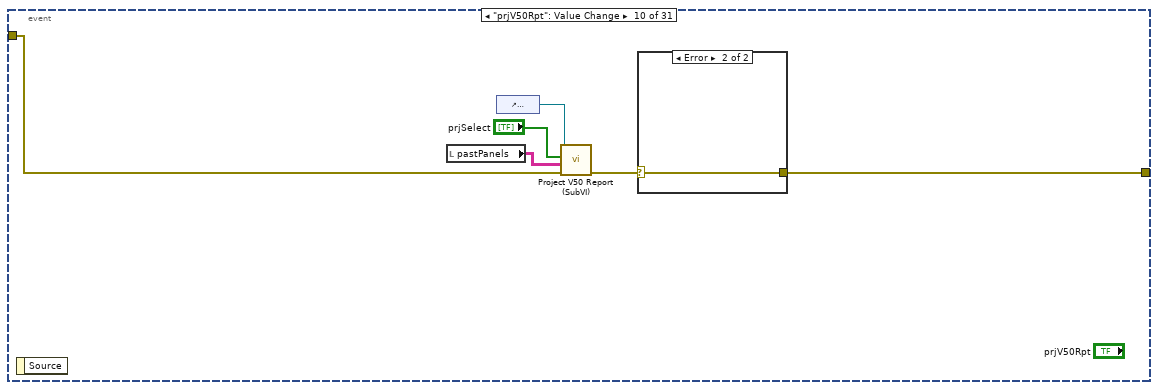
[diagram p18: hidden frame]
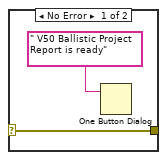
[diagram p19: hidden frame]
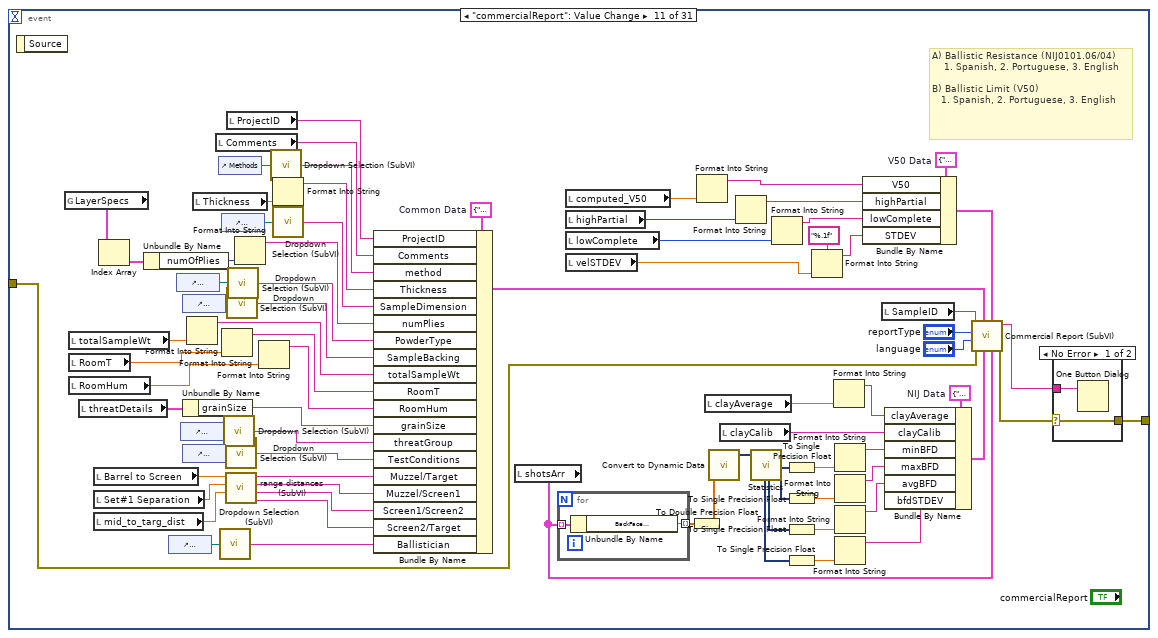
[diagram p20: hidden frame]
diagram:
  w16 = T15 3 items=["no dialog", "OK message", "continue or stop message", "OK message + warnings", "continue/stop + warnings"] ("type of dialog (OK msg:1)")
  w26 = T6 [{"Uncorrected Impact"=0.0, "Uncorrected Residual"=0.0, "avgVel_PB"=0.0, "IMPACT VELOCITY"=0.0, "RESIDUAL  VELOCITY "=0.0, "Shot Description"="", "Powder Loading "=0.0, "Barrel Temperature"=0.0, "TIME / DATE"="", "shot order"=1, "SHOT STATUS"=1, "Shot Angle"=0, "Corrected Impact"=0.0, "Corrected residual"=0.0, "Projectile Mass"=0.0, "usedv50"=FALSE, "Energy Loss (J)"=0.0, "BackFace\nDepth"=0.0, "BackFace\nDiameter"=0.0, "Redundant_Velocity"=0.0, "velLoss_PB"=0.0, "strikeVel_PB"=0.0, "UncorrectedRed_PB"=0.0, "CorrectedRed_PB"=0.0, "UncorrectedAvgVel_PB"=0.0, "V50userExcl"=FALSE, "Frag Rod"=0.0, "fairHit"=FALSE}]  # shotsArr
  w27 = errorcluster {"status"=FALSE, "code"=0, "source"=""}  # error in
  n1 = property on="RESET All" class="Bool (strict)"("Value"=TRUE ("RESET")) -> (error out=w5:errorcluster)  [unwired: 2 in, 1 out]
  n2 = Initialize Array(0.0, 2 ("dimension size")) -> (w6:dbl[])
  n3 = Obtain Queue(element data type=w6, error in (no error)=w5) -> (queue out=w3:refnum<queue>, error out=w21:errorcluster)  [unwired: 3 in, 1 out]
  n4 = call "Config Counter to Measure Two Edge Separation.vi"("errIN"=w5, "SampClk.Timebase.Src"="SampClk.Timebase.Src", "Counter"="ctr0") -> ("errOUT"=w10:errorcluster, "task out"=w2:refnum<k21>)  [unwired: 7 in]
  "taskCtr0" <- w2
  n5 = call "Config Counter to Measure Two Edge Separation.vi"("errIN"=w5, "SampClk.Timebase.Src"="SampClk.Timebase.Src", "Counter"="ctr1") -> ("errOUT"=w9:errorcluster, "task out"=w1:refnum<k21>)  [unwired: 7 in]
  "taskCtr1" <- w1
  n6 = call <vilib>:"Simple Error Handler.vi"("error in (no error)"=w5) -> ("error out"=w22:errorcluster)  [unwired: 4 in, 4 out]
  n7 = while "U/I Event Handler" {
    shift-right: [w31] -> _
    shift-left: w27 -> [w32]
    stop <- FALSE stop-if-true
    n8 = event shown="[11] \"pastPanels\": Mouse Up" {
      selector: _ -> [_ _ _ _ _ _ _ _ _ _ _ _ _ _ _ _ _ _ _ _ _ _ _ _ _ _ _ _ _ _ _]
      dyn-events: _ -> [_ _ _ _ _ _ _ _ _ _ _ _ _ _ _ _ _ _ _ _ _ _ _ _ _ _ _ _ _ _ _]
      timeout: 100 -> [_ _ _ _ _ _ _ _ _ _ _ _ _ _ _ _ _ _ _ _ _ _ _ _ _ _ _ _ _ _ _]
      tunnel: w32 -> [w35 w38 w65 w75 w83 w85 w122 w140 w159 w166 w195 w261 w295 w332 w374 w412 w414 w450 w486 w493 w501 w528 w530 w539 w565 w582 w584 w594 w637 w668 _]
      tunnel: [w35 w40 w65 w72 w83 w84 w121 w140 w149 w164 w250 w258 w303 w331 w371 w412 w414 w450 w486 w492 w497 w528 w530 w536 w562 w582 w584 w593 w639 w668 w675] -> w31
      event Timeout {
        n9 = event-data() -> ()  [unwired: 2 out]
        n10 = Get Date/Time In Seconds() -> (seconds since 1Jan1904=w37:timestamp)
        n11 = Format Date/Time String(seconds (now)=w37) -> (date/time string=→"TimeNow":string)  [unwired: 2 out]
      }
      event "EXIT": Value Change {
        n12 = event-data() -> ()  [unwired: 2 out]
        n13 = Two Button Dialog(message="Exit BIMS Collector?\nAll Unsaved data will be lost.", 1:"NO" ("F button name (\"Cancel\")"), 2:"YES" ("T button name (\"OK\")")) -> (T button?=w39:bool)
        n14 = case shown="True" w39 {
          selector: w39 -> [_ w47]
          tunnel: [w44 w48] -> w40
          tunnel: w38 -> [w44 _]
          frame False {
          }
          frame True {
            n15 = flat-sequence {
              tunnel: w47 -> [w53]
              tunnel: [w53] -> w45
              tunnel: [w55] -> w46
              tunnel: w45 -> [w55]
              tunnel: [w57] -> w48
              tunnel: w46 -> [w56]
              frame #0 {
                n16 = local read "taskCtr0"() -> (w51:refnum<k21>)
                n17 = call <vilib>:"DAQmx Clear Task.vi"("task in"=w51) -> ("error out"=w50:errorcluster)  [unwired: 14 in]
                n18 = local read "taskCtr1"() -> (w52:refnum<k21>)
                n19 = call <vilib>:"DAQmx Clear Task.vi"("task in"=w52, "error in"=w50) -> ("error out"=w49:errorcluster)  [unwired: 13 in]
                n20 = call <vilib>:"Simple Error Handler.vi"("error in (no error)"=w49) -> ()  [unwired: 4 in, 5 out]
              }
              frame #1 {
                # "close arming loop 1st"
                n21 = local write "close arming loop"(w55) -> ()
                n22 = Wait (ms)(milliseconds to wait=u32 1000) -> ()  [unwired: 1 out]
              }
              frame #2 {
                n23 = property on="Property Node" class="Application"(error in=errorcluster {"status"=FALSE, "code"=0, "source"=""} ("error in (no error)")) -> (error out=w57:errorcluster, "Application:Kind"=w59:T18)  [unwired: 1 in, 1 out]
                n24 = case shown="\"Run Time System\"" w59 {
                  tunnel: w56 -> [w60 w61 w62]
                  frame Default {
                    n25 = Stop(stop? (T)=w60) -> ()
                  }
                  frame "Development System" {
                    n26 = Stop(stop? (T)=w61) -> ()
                  }
                  frame "Run Time System" {
                    n27 = Quit LabVIEW(quit? (T)=w62) -> ()
                  }
                }
              }
            }
          }
        }
      }
      event "diagPageVisible": Value Change {
        # "Toggles display of \"Internal Use\" tab for diagnostics purposes"
        # "Key navigation ONLY: Cntrl-Shift-F11"
        n28 = event-data() -> ("NewVal"=w68:bool)  [unwired: 1 out]
        n29 = property on="aboutTabCntrl" class="TabCtl (strict)"(error in=errorcluster {"status"=FALSE, "code"=0, "source"=""} ("error in (no error)")) -> (error out=w67:errorcluster, "Pages"=w71:refnum<vi>[])  [unwired: 1 in, 1 out]
        n30 = Index Array(array=w71, index=2) -> (element=w69:refnum<vi>)
        n31 = property on="Property Node" class="Page"(reference=w69, error in=w67, "PageVis"=w68) -> (error out=w66:errorcluster)  [unwired: 1 out]
        n32 = property on="diagPageVisible" class="Bool (strict)"(error in=w66, "Value"=w68) -> (error out=w63:errorcluster)  [unwired: 1 in, 1 out]
        n33 = call <vilib>:"General Error Handler.vi"("error in (no error)"=w63) -> ()  [unwired: 2 in, 13 out]
      }
      event "runtimeMenusVisible": Value Change {
        # "Key navigation ONLY: Cntrl-Shift-F10"
        n34 = event-data() -> ("NewVal"=w77:bool)  [unwired: 1 out]
        n35 = control-ref of="This VI"() -> (w76:refnum<vi>)
        n36 = property class="VI"(reference=w76, error in=w75, "Front Panel.ShowMenuBar"=w77) -> (reference out=w74:refnum<vi>, error out=w73:errorcluster)
        n37 = Close Reference(reference=w74, error in (no error)=w73) -> (error out=w72:errorcluster)
      }
      event "MeasVelScrnSet1", "MeasVelScrnSet2": Value Change {
        n38 = event-data() -> ()  [unwired: 2 out]
        n39 = local read "MeasVelScrnSet1"() -> (w82:sgl)
        n40 = local read "MeasVelScrnSet2"() -> (w81:sgl)
        n41 = Add(x=w82, y=w81) -> (x+y=w80:sgl)
        n42 = Divide(x=w80, y=sgl 2.0) -> (x/y=w78:sgl)
        n43 = local write "Current/avg/speed"(w78) -> ()
      }
      event "QueryLoad": Value Change {
        w90 = "%x" ("time format string (%c)")
        w106 = "" ("replace string (\"\")")
        # "This section plots  Impact velocity vs. loadingdata"
        n44 = event-data() -> ()  [unwired: 2 out]
        n45 = Format Date/Time String(time format string (%c)=w90, seconds (now)="lkupStartDate") -> (date/time string=w89:string)  [unwired: 1 out]
        n46 = Format Date/Time String(time format string (%c)=w90, seconds (now)="lkupEndDate") -> (date/time string=w88:string)  [unwired: 1 out]
        n47 = call "Trim String.vi"("inStr"="Powder.freeTxt") -> ("outStr"=w104:string)
        n48 = call "Trim String.vi"("inStr"="Threat.freeTxt") -> ("outStr"=w105:string)
        n49 = invoke on="v50_table" class="Tbl" method="Reinit To Default"(error in=w85) -> (error out=w97:errorcluster)  [unwired: 2 in, 2 out]
        n50 = invoke on="Vel.vs.Loading" class="WFGraph (strict)" method="Reinit To Default"(error in=w97) -> (error out=w92:errorcluster)  [unwired: 2 in, 2 out]
        n51 = Format Into String(format string="SELECT TOP %d dbsrc.experiment.threat, dbsrc.shots.loading, dbsrc.shots.impact, dbsrc.experiment.powder, dbsrc.shots.date from dbsrc.shots, dbsrc.experiment where dbsrc.shots.expt = dbsrc.experiment.expt and dbsrc.shots.loading > 0 and dbsrc.shots.date between '%s' and '%s' and dbsrc.shots.impact between 10 and 5000 and dbsrc.experiment.powder like '%%%s%%' and dbsrc.experiment.threat like '%%%s%%' and experiment.threat<>'' order by dbsrc.experiment.threat, dbsrc.shots.loading, dbsrc.shots.impact;" ("Format String"), error in=w92, "maxRecs", w89, w88, w104, w105) -> (resulting string=w110:string, error out=w95:errorcluster)  [unwired: 1 in]
        n52 = Search and Replace String(input string=w110, search string=" and experiment.powder like '%%'", replace string=w106, error in=w95) -> (result string=w108:string, error out=w96:errorcluster)  [unwired: 6 out]
        n53 = Search and Replace String(input string=w108, search string="and experiment.threat like '%%'", replace string=w106, error in=w96) -> (result string=w99:string, error out=w94:errorcluster)  [unwired: 6 out]
        n54 = call "Fetch Data (SubVI).vi"("error IN"=w94, "query string"=w99) -> ("error OUT"=w84:errorcluster, "recordset data"=w100:string[][])  [unwired: 4 out]
        "v50_table" <- w100
        n55 = Fract/Exp String To Number(string=w100) -> (number=w114:dbl[][])  [unwired: 4 out]
        n56 = Array Size(array=w100) -> (size(s)=w102:i32[])
        n57 = Index Array(array=w102) -> (element=→"ActualNumRecs":i32)  [unwired: 1 in]
        n58 = Index Array(array=w114, index (col)=2 ("Disabled Index (col)")) -> (element=w113:dbl[])  [unwired: 1 in]
        n59 = Index Array(array=w114, index (col)=1 ("Disabled Index (col)")) -> (element=w112:dbl[])  [unwired: 1 in]
        n60 = Bundle(w112, w113) -> (→"Vel.vs.Loading":cluster{dbl[], dbl[]})  [unwired: 1 out]
      }
      event "ThreatGroups": Value Change {
        n61 = event-data() -> ()  [unwired: 2 out]
        n62 = control-ref of="ThreatGroups"() -> (w123:refnum<vi>)
        n63 = property on="Property Node" class="Ring (strict)"(reference=w123, error in=w122) -> (error out=w120:errorcluster, "RingText.Text"=w118:string)  [unwired: 1 out]
        n64 = Not Equal?(x=w118, y="") -> (x != y?=w117:bool)
        n65 = case shown="True" w117 {
          tunnel: w118 -> [_ w132]
          tunnel: [w124 w130] -> w121
          tunnel: w120 -> [w127 w129]
          frame False {
            n66 = property on="ThreatDetails" class="Ring (strict)"(error in=w127, "Strings []"=string[] [], "Value"=u16 0 ("Value (Signaling)")) -> (error out=w125:errorcluster)  [unwired: 1 in, 1 out]
            n67 = invoke on="threatDetails" class="Clust (strict)" method="Reinit To Default"(error in=w125) -> (error out=w124:errorcluster)  [unwired: 2 in, 2 out]
          }
          frame True {
            n68 = call "Select Threat Details.vi"("threatGroup"=w132) -> ("threatDetails"=w131:string[])  [unwired: 1 out]
            n69 = property on="ThreatDetails" class="Ring (strict)"(error in=w129, "Strings []"=w131, "Val(Sgnl)"=u16 0 ("Value (Signaling)")) -> (error out=w130:errorcluster)  [unwired: 1 in, 1 out]
          }
        }
      }
      event "prjAll": Value Change {
        n70 = event-data() -> ()  [unwired: 2 out]
        n71 = local read "prjSelect"() -> (w136:bool[])
        n72 = local read "actualNumPanels"() -> (w139:i32)
        n73 = And Array Elements(Boolean array=w136) -> (logical AND=w134:bool)
        n74 = Not(x=w134) -> (.not. x?=w135:bool)
        n75 = Initialize Array(w135, w139) -> (w138:bool[])
        n76 = local write "prjSelect"(w138) -> ()
        n77 = local write "prjAll"(FALSE ("prjAll")) -> ()
      }
      event "panelSearch", "ProjectID_0": Value Change {
        # "This section returns past panels"
        n78 = event-data() -> ()  [unwired: 2 out]
        n79 = local read "pastPanels"() -> (w142:string[][])
        n80 = control-ref of="pastPanels"() -> (w145:refnum<vi>)
        n81 = control-ref of="ProjectID_0"() -> (w144:refnum<vi>)
        n82 = control-ref of="Mfr_0"() -> (w147:refnum<vi>)
        n83 = control-ref of="SampleStyle_0"() -> (w146:refnum<vi>)
        n84 = control-ref of="Requestors_0"() -> (w158:refnum<vi>)
        n85 = control-ref of="ThreatSize_0"() -> (w157:refnum<vi>)
        n86 = Bundle("Mfr_0"=w147, "SampleStyle_0"=w146, "pastPanels"=w145, "ProjectID_0"=w144) -> (w143:T19)  [unwired: 1 in]
        n87 = call "queryPanels (SubVI).vi"("ThreatSize_0"=w157, "Requestors_0"=w158, "append"="appendPrjs", "error in"=w159, "srchParams"="srchParams", "recoSet_IN"=w142, "criteria"=w143) -> ("error out"=w149:errorcluster, "recoSet_OUT"=w156:string[][], "actualNumPanels"=→"actualNumPanels":i32)  [unwired: 2 in]
        "pastPanels" <- w156
        n88 = Index Array(array=w156) -> (element=w151:string[])  [unwired: 2 in]
        n89 = Array Size(array=w151) -> (size(s)=w155:i32)
        n90 = Greater Than 0?(x=w155) -> (x > 0?=w154:bool)
        n91 = Select(t=T16."Enabled" ("Disabled"), s=w154, f=T16."Disabled and Grayed Out" ("Disabled")) -> (s? t:f=w148:T16)
        n92 = flat-sequence {
          tunnel: w149 -> [_]
          frame #0 {
            n93 = local read "actualNumPanels"() -> (w163:i32)
            n94 = Initialize Array(TRUE ("element"), w163) -> (w162:bool[])
            n95 = local write "prjSelect"(w162) -> ()
          }
        }
        n96 = property on="reportV50_History" class="Bool"("DisabledEnum"=w148) -> ()  [unwired: 2 in, 2 out]
        n97 = property on="prjV50Rpt" class="Bool"("DisabledEnum"=w148) -> ()  [unwired: 2 in, 2 out]
      }
      event "prjV50Rpt": Value Change {
        n98 = event-data() -> ()  [unwired: 2 out]
        n99 = local read "pastPanels"() -> (w168:string[][])
        n100 = control-ref of="ProjectID_0"() -> (w167:refnum<vi>)
        n101 = call "Project V50 Report (SubVI).vi"("errIN"=w166, "pastPanels"=w168, "prjSelect"="prjSelect", "Project ID"=w167) -> ("errOUT"=w165:errorcluster)  [unwired: 7 in]
        n102 = case shown="Error" w165 {
          selector: w165 -> [w170 w172]
          tunnel: [w170 w172] -> w164
          frame No Error {
            n103 = One Button Dialog(message=" V50 Ballistic Project Report is ready") -> ()  [unwired: 2 out]
          }
          frame Error {
          }
        }
      }
      event "commercialReport": Value Change {
        w194 = T20 {"clayAverage"="", "clayCalib"="", "maxBFD"="", "minBFD"="", "avgBFD"="", "bfdSTDEV"=""}  # NIJ Data
        w202 = T21 {"V50"="", "highPartial"="", "lowComplete"="", "STDEV"=""}  # V50 Data
        w244 = T22 {"ProjectID"="", "Comments"="", "method"="", "Thickness"="", "SampleDimension"="", "numPlies"="", "PowderType"="", "SampleBacking"="", "totalSampleWt"="", "RoomHum"="", "RoomT"="", "grainSize"="", "threatGroup"="", "TestConditions"="", "Muzzel/Target"="", "Muzzel/Screen1"="", "Screen1/Screen2"="", "Screen2/Target"="", "Ballistician"=""}  # Common Data
        # "A)\tBallistic Resistance (NIJ0101.06/04)\n    1.\tSpanish, 2.\tPortuguese, 3.\tEnglish\n\nB)\tBallistic Limit (V50)\n   1.\tSpanish, 2.\tPortuguese, 3.\tEnglish"
        n104 = event-data() -> ()  [unwired: 2 out]
        n105 = global read "BIMS_Collector Globals.vi" "LayerSpecs"() -> (w234:T23)
        n106 = local read "totalSampleWt"() -> (w226:sgl)
        n107 = local read "RoomT"() -> (w224:sgl)
        n108 = local read "RoomHum"() -> (w223:sgl)
        n109 = local read "threatDetails"() -> (w236:T1)
        n110 = local read "Barrel to Screen"() -> (w216:sgl)
        n111 = local read "Set#1 Separation"() -> (w214:sgl)
        n112 = local read "mid_to_targ_dist"() -> (w215:sgl)
        n113 = Index Array(array=w234) -> (element=w233:T24)  [unwired: 1 in]
        n114 = Unbundle By Name(w233) -> ("numOfPlies"=w232:i32)
        n115 = control-ref of="Ballisticians"() -> (w209:refnum<vi>)
        n116 = control-ref of="PowderTypes"() -> (w230:refnum<vi>)
        n117 = control-ref of="ThreatGroups"() -> (w220:refnum<vi>)
        n118 = control-ref of="SampleBackings"() -> (w228:refnum<vi>)
        n119 = Unbundle By Name(w236) -> ("grainSize"=w235:string)
        n120 = control-ref of="TestConditions"() -> (w218:refnum<vi>)
        n121 = Format Into String(w226) -> (resulting string=w225:string)  [unwired: 3 in, 1 out]
        n122 = local read "Thickness"() -> (w240:dbl)
        n123 = local read "Comments"() -> (w242:string)
        n124 = control-ref of="Methods"() -> (w245:refnum<vi>)
        n125 = call "Dropdown Selection (SubVI).vi"("reference"=w209) -> ("element"=w208:string)
        n126 = control-ref of="SampleDimensions"() -> (w238:refnum<vi>)
        n127 = Format Into String(w224) -> (resulting string=w222:string)  [unwired: 3 in, 1 out]
        n128 = call "Dropdown Selection (SubVI).vi"("reference"=w220) -> ("element"=w219:string)
        n129 = call "Dropdown Selection (SubVI).vi"("reference"=w218) -> ("element"=w217:string)
        n130 = call "range distances (SubVI).vi"("mid_to_targ_dist"=w215, "Set#1 Separation"=w214, "Barrel to Screen"=w216) -> ("scr#2 / target"=w211:string, "Set#1 Separation"=w210:string, "muzzle / scr#1"=w212:string, "muzzle / target"=w213:string)  [unwired: 3 in, 1 out]
        n131 = local read "ProjectID"() -> (w243:string)
        n132 = call "Dropdown Selection (SubVI).vi"("reference"=w228) -> ("element"=w227:string)
        n133 = call "Dropdown Selection (SubVI).vi"("reference"=w230) -> ("element"=w229:string)
        n134 = Format Into String(w232) -> (resulting string=w231:string)  [unwired: 3 in, 1 out]
        n135 = Format Into String(w223) -> (resulting string=w221:string)  [unwired: 3 in, 1 out]
        n136 = call "Dropdown Selection (SubVI).vi"("reference"=w245) -> ("element"=w241:string)
        n137 = Format Into String(w240) -> (resulting string=w239:string)  [unwired: 3 in, 1 out]
        n138 = call "Dropdown Selection (SubVI).vi"("reference"=w238) -> ("element"=w237:string)
        n139 = Bundle By Name(cluster=w244, "ProjectID"=w243, "Comments"=w242, "method"=w241, "Thickness"=w239, "SampleDimension"=w237, "numPlies"=w231, "PowderType"=w229, "SampleBacking"=w227, "totalSampleWt"=w225, "RoomT"=w222, "RoomHum"=w221, "grainSize"=w235, "threatGroup"=w219, "TestConditions"=w217, "Muzzel/Target"=w213, "Muzzel/Screen1"=w212, "Screen1/Screen2"=w210, "Screen2/Target"=w211, "Ballistician"=w208) -> (w197:T22)
        n140 = local read "shotsArr"() -> (w173:T6)
        n141 = for {
          tunnel: w173 -> [w252] mode=indexing
          tunnel: [w251] -> w189 mode=indexing
          n142 = Unbundle By Name(w252) -> ("BackFace\nDepth"=w251:sgl)
        }
        n143 = local read "computed_V50"() -> (w204:sgl)
        n144 = local read "highPartial"() -> (w205:i32)
        n145 = local read "lowComplete"() -> (w206:i32)
        n146 = local read "velSTDEV"() -> (w207:sgl)
        n147 = To Double Precision Float(number=w189) -> (double precision float=w187:dbl[])
        n148 = Format Into String(w204) -> (resulting string=w201:string)  [unwired: 3 in, 1 out]
        n149 = local read "clayAverage"() -> (w192:sgl)
        n150 = call "Convert to Dynamic Data"("Array"=w187) -> ("Dynamic Data Type"=w188:dynamicdata)  [unwired: 3 in]
        n151 = local read "clayCalib"() -> (w193:string)
        n152 = Format Into String(w205) -> (resulting string=w200:string)  [unwired: 3 in, 1 out]
        n153 = call "Statistics"("Signals"=w188) -> ("Standard Dev"=w176:dynamicdata, "Arithmetic Mean"=w179:dynamicdata, "Minimum"=w186:dynamicdata, "Maximum"=w182:dynamicdata)  [unwired: 22 in, 1 out]
        n154 = Format Into String(w206) -> (resulting string=w199:string)  [unwired: 3 in, 1 out]
        n155 = To Single Precision Float(number=w186) -> (single precision float=w185:sgl)
        n156 = To Single Precision Float(number=w182) -> (single precision float=w184:sgl)
        n157 = To Single Precision Float(number=w179) -> (single precision float=w183:sgl)
        n158 = To Single Precision Float(number=w176) -> (single precision float=w177:sgl)
        n159 = Format Into String(format string="%.1f", w207) -> (resulting string=w198:string)  [unwired: 2 in, 1 out]
        n160 = Format Into String(w192) -> (resulting string=w191:string)  [unwired: 3 in, 1 out]
        n161 = Format Into String(w185) -> (resulting string=w181:string)  [unwired: 3 in, 1 out]
        n162 = Format Into String(w184) -> (resulting string=w180:string)  [unwired: 3 in, 1 out]
        n163 = Format Into String(w183) -> (resulting string=w178:string)  [unwired: 3 in, 1 out]
        n164 = Format Into String(w177) -> (resulting string=w175:string)  [unwired: 3 in, 1 out]
        n165 = Bundle By Name(cluster=w202, "V50"=w201, "highPartial"=w200, "lowComplete"=w199, "STDEV"=w198) -> (w196:T21)
        n166 = local read "SampleID"() -> (w247:string)
        n167 = Bundle By Name(cluster=w194, "clayAverage"=w191, "clayCalib"=w193, "minBFD"=w181, "maxBFD"=w180, "avgBFD"=w178, "bfdSTDEV"=w175) -> (w190:T20)
        n168 = call "Commercial Report (SubVI).vi"("shotsArr"=w173, "V50 Data"=w196, "NIJ Data"=w190, "Common Data"=w197, "errIN"=w195, "language"="language", "reportType"="reportType", "SampleID"=w247) -> ("errOUT"=w249:errorcluster, "rptStat"=w174:string)  [unwired: 2 in]
        n169 = case shown="No Error" w249 {
          selector: w249 -> [w254 w255]
          tunnel: [w254 w255] -> w250
          tunnel: w174 -> [w253 _]
          frame No Error {
            n170 = One Button Dialog(message=w253) -> ()  [unwired: 2 out]
          }
          frame Error {
          }
        }
      }
      event "pastPanels": Mouse Up {
        n171 = event-data() -> ("CtlRef"=w269:refnum<vi>)  [unwired: 1 out]
        n172 = property on="Property Node" class="Tbl (strict)"(reference=w269, error in=w261) -> (error out=w260:errorcluster, "Value"=w268:string[][], "EditPos"=w267:T25, "Index Values"=w257:T26)  [unwired: 1 out]
        n173 = Cluster To Array(cluster=w257) -> (array=w256:u32[])
        n174 = property on="prjSelect" class="Arr (strict)"("Index Values"=w256) -> ()  [unwired: 2 in, 2 out]
        n175 = Unbundle By Name(w267) -> ("Row"=w266:i32)
        n176 = Index Array(array=w268, index (row)=w266, index (col)=0 ("disabled index (col)")) -> (element=w265:string)
        n177 = Scan From String(input string=w265, error in=w260, default 1=1 ("Record #")) -> (error out=w259:errorcluster, output 1=w263:i32)  [unwired: 2 in, 2 out]
        n178 = case shown="Error" w259 {
          selector: w259 -> [w270 w273]
          tunnel: w263 -> [w271 _]
          tunnel: [w270 w274] -> w258
          frame No Error {
            n179 = local write "Record #"(w271) -> ()
          }
          frame Error {
            # "clear Error 1"
            n180 = Unbundle By Name(w273) -> ("code"=w277:i32)
            n181 = Decrement(x=w277) -> (x-1=w276:i32)
            n182 = Equal To 0?(x=w276) -> (x = 0?=w275:bool)
            n183 = Select(t=errorcluster {"status"=FALSE, "code"=0, "source"=""} ("error IO"), s=w275, f=w273) -> (s? t:f=w274:errorcluster)
          }
        }
      }
      event "ThreatDetails", "SampleID": Value Change {
        # "A Sample ID is entered"
        # "A range is selected"
        # "A measurement requires the selection of a threat,\nso delay enabling the \"Measure\" tab until a grain wt\nis chosen."
        n184 = event-data() -> ()  [unwired: 2 out]
        n185 = control-ref of="ThreatGroups"() -> (w296:refnum<vi>)
        n186 = control-ref of="ThreatDetails"() -> (w293:refnum<vi>)
        n187 = call "Get Projectile Atributes from ThreatGroupDetail.vi"("error IN"=w295, "ThreatDetail"=w293, "ThreatGroup"=w296) -> ("error out"=w294:errorcluster, "projectileAttribs"=w292:T27)  [unwired: 1 out]
        "threatDetails" <- w292
        n188 = Unbundle By Name(w292) -> ("grainSize"=w285:string)
        n189 = Equal?(x=w285, y="") -> (x = y?=w286:bool)
        n190 = case shown="False" w286 {
          tunnel: w285 -> [w313 _]
          tunnel: [w312 u16 0 ("GrainSize")] -> w291
          frame False {
            # "A grain size is selected"
            n191 = Scan From String(input string=w313) -> (output 1=w312:u16)  [unwired: 3 in, 4 out]
            "GrainSize" <- w312
          }
          frame True {
            # "A grain size not selected"
          }
        }
        n192 = Equal?(x=w285, y="") -> (x = y?=w310:bool)
        n193 = local read "rangeSetup"() -> (w307:u16)
        n194 = case shown="False" w310 {
          tunnel: [w317 sgl 0.0] -> w306
          tunnel: w285 -> [w315 _]
          frame False {
            w319 = sgl 0.0  # sgl
            n195 = Scan From String(format string="%f " ("Format String"), input string=w315, default 1=w319) -> (output 1=w318:sgl)  [unwired: 2 in, 3 out]
            n196 = disable-structure shown="Enabled" {
              disable-tunnel: w318 -> [w322 w323]
              disable-tunnel: [w321 w323] -> w317
              frame Disabled {
                n197 = Multiply(x=sgl 0.06479891, y=w322) -> (x*y=w321:sgl)
              }
              frame Enabled {
              }
            }
          }
          frame True {
          }
        }
        "Projectile Mass" <- w306
        n198 = local read "SampleID"() -> (w290:string)
        n199 = Greater Than 0?(x=w307) -> (x > 0?=w308:bool)
        n200 = Greater Than 0?(x=w291) -> (x > 0?=w309:bool)
        n201 = Not Equal?(x=w290, y="") -> (x != y?=w288:bool)
        n202 = Compound Arithmetic op=AND(w309, w308, w288) -> (w283:bool)
        n203 = property on="mainTabCntrl" class="TabCtl (strict)"(error in=w294) -> (error out=w299:errorcluster, "Pages"=w302:refnum<vi>[])  [unwired: 1 in, 1 out]
        n204 = Not(x=w283) -> (.not. x?=w298:bool)
        n205 = Index Array(array=w302, index=1) -> (element=w300:refnum<vi>)
        n206 = Select(t=T17."Page Enabled" ("Page Enabled State"), s=w283, f=T17."Page Disabled & Grayed" ("Page Enabled State")) -> (s? t:f=w282:T17)
        n207 = property on="Property Node" class="Page"(reference=w300, error in=w299, "PageEnb"=w282) -> (error out=w297:errorcluster)  [unwired: 1 out]
        n208 = Select(t=T16."Enabled" ("Disabled"), s=w283, f=T16."Disabled and Grayed Out" ("Disabled")) -> (s? t:f=w280:T16)
        n209 = property on="ARM" class="Bool"(error in=w297, "Disabled"=w280) -> (error out=w305:errorcluster)  [unwired: 1 in, 1 out]
        n210 = property on="addShot" class="Bool"(error in=w305, "Disabled"=w280) -> (error out=w304:errorcluster)  [unwired: 1 in, 1 out]
        n211 = property on="instruct_addShot" class="Str"(error in=w304, "Visible"=w298) -> (error out=w303:errorcluster)  [unwired: 1 in, 1 out]
      }
      event "Mfr_1", "Mfr_2", "Mfr_3", "Mfr_4", "Mfr_5", "Mfr_6", "Mfr_0": Value Change {
        n212 = event-data() -> ("CtlRef"=w340:refnum<vi>)  [unwired: 1 out]
        n213 = property on="Property Node" class="Ring (strict)"(reference=w340, error in=w332) -> (error out=w330:errorcluster, "Label.Text"=w336:string, "RingText.Text"=w337:string)  [unwired: 1 out]
        n214 = flat-sequence {
          tunnel: ["Mfr_1"] -> _
          tunnel: ["Mfr_2"] -> _
          tunnel: ["Mfr_3"] -> _
          tunnel: ["Mfr_4"] -> _
          tunnel: ["Mfr_5"] -> _
          tunnel: ["Mfr_6"] -> _
          frame #0 {
          }
        }
        n215 = call "Select Sample Style.vi"("error IN"=w330, "Mfr"=w337) -> ("error Out"=w329:errorcluster, "SampleStyles"=w326:string[])  [unwired: 4 out]
        n216 = Scan From String(format string="Mfr_%d", input string=w336, error in=w329, default 1=0 ("Mfr#")) -> (error out=w327:errorcluster, output 1=w335:i32)  [unwired: 1 in, 2 out]
        n217 = case shown="1" w335 {
          tunnel: [w352 w355 w358 w361 w364 w367 w370] -> w334
          tunnel: [w351 w354 w357 w360 w363 w366 w369] -> w328
          tunnel: w327 -> [w351 w354 w357 w360 w363 w366 w369]
          tunnel: w326 -> [w350 w353 w356 w359 w362 w365 w368]
          tunnel: [w349 w353 w356 w359 w362 w365 w368] -> w325
          frame 0, Default {
            n218 = Delete From Array(array=w350, length=1, index=0) -> (array with subset deleted=w349:string[])  [unwired: 1 out]
            n219 = control-ref of="SampleStyle_0"() -> (w352:refnum<vi>)
          }
          frame 1 {
            n220 = control-ref of="SampleStyle_1"() -> (w355:refnum<vi>)
          }
          frame 2 {
            n221 = control-ref of="SampleStyle_2"() -> (w358:refnum<vi>)
          }
          frame 3 {
            n222 = control-ref of="SampleStyle_3"() -> (w361:refnum<vi>)
          }
          frame 4 {
            n223 = control-ref of="SampleStyle_4"() -> (w364:refnum<vi>)
          }
          frame 5 {
            n224 = control-ref of="SampleStyle_5"() -> (w367:refnum<vi>)
          }
          frame 6 {
            n225 = control-ref of="SampleStyle_6"() -> (w370:refnum<vi>)
          }
        }
        n226 = property on="Property Node" class="Ring (strict)"(reference=w334, error in=w328, "Strings []"=w325, "Val(Sgnl)"=u16 0 ("Value (Signaling)")) -> (error out=w331:errorcluster)  [unwired: 1 out]
      }
      event "SampleStyle_1", "SampleStyle_2", "SampleStyle_3", "SampleStyle_4", "SampleStyle_5", "SampleStyle_6", "SampleStyle_0": Value Change {
        n227 = event-data() -> ("CtlRef"=w380:refnum<vi>)  [unwired: 1 out]
        n228 = call "Get Sample Style Atributes.vi"("StyleNumRef"=w380) -> ("SampleSpecs"=w375:T28)  [unwired: 1 in]
        n229 = flat-sequence {
          tunnel: ["SampleStyle_1"] -> _
          tunnel: ["SampleStyle_2"] -> _
          tunnel: ["SampleStyle_3"] -> _
          tunnel: ["SampleStyle_4"] -> _
          tunnel: ["SampleStyle_5"] -> _
          tunnel: ["SampleStyle_6"] -> _
          frame #0 {
          }
        }
        n230 = property on="Property Node" class="Ring (strict)"(reference=w380, error in=w374) -> (error out=w373:errorcluster, "Label.Text"=w379:string)  [unwired: 1 out]
        n231 = Scan From String(format string="SampleStyle_%d", input string=w379, error in=w373, default 1=0 ("default value 1")) -> (error out=w372:errorcluster, output 1=w377:i32)  [unwired: 1 in, 2 out]
        n232 = case shown="1" w377 {
          tunnel: w375 -> [w389 w392 w395 w398 w401 w404 w407]
          tunnel: w372 -> [w388 w391 w394 w397 w400 w403 w406]
          tunnel: [w387 w390 w393 w396 w399 w402 w405] -> w371
          frame 0, Default {
            n233 = property on="SampleAttribs_0" class="Clust (strict)"(error in=w388, "Val(Sgnl)"=w389) -> (error out=w387:errorcluster)  [unwired: 1 in, 1 out]
            "SampleAttribs_0" <- w389
          }
          frame 1 {
            n234 = property on="SampleAttribs_1" class="Clust (strict)"(error in=w391, "Val(Sgnl)"=w392) -> (error out=w390:errorcluster)  [unwired: 1 in, 1 out]
            "SampleAttribs_1" <- w392
          }
          frame 2 {
            n235 = property on="SampleAttribs_2" class="Clust (strict)"(error in=w394, "Val(Sgnl)"=w395) -> (error out=w393:errorcluster)  [unwired: 1 in, 1 out]
            "SampleAttribs_2" <- w395
          }
          frame 3 {
            n236 = property on="SampleAttribs_3" class="Clust (strict)"(error in=w397, "Val(Sgnl)"=w398) -> (error out=w396:errorcluster)  [unwired: 1 in, 1 out]
            "SampleAttribs_3" <- w398
          }
          frame 4 {
            n237 = property on="SampleAttribs_4" class="Clust (strict)"(error in=w400, "Val(Sgnl)"=w401) -> (error out=w399:errorcluster)  [unwired: 1 in, 1 out]
            "SampleAttribs_4" <- w401
          }
          frame 5 {
            n238 = property on="SampleAttribs_5" class="Clust (strict)"(error in=w403, "Val(Sgnl)"=w404) -> (error out=w402:errorcluster)  [unwired: 1 in, 1 out]
            "SampleAttribs_5" <- w404
          }
          frame 6 {
            n239 = property on="SampleAttribs_6" class="Clust (strict)"(error in=w406, "Val(Sgnl)"=w407) -> (error out=w405:errorcluster)  [unwired: 1 in, 1 out]
            "SampleAttribs_6" <- w407
          }
        }
      }
      event "Sort by AVG": Value Change {
        n240 = event-data() -> ()  [unwired: 2 out]
        n241 = local read "shotsArr"() -> (w410:T6)
        n242 = local read "Site"() -> (w408:string)
        n243 = call "Update Shot Table.vi"("Sort by AVG"="Sort by AVG", "Site"=w408, "shotsArr"=w410) -> ("shotTable OUT"=→"Table of Shots":string[][])
      }
      event "Layer_1", "Layer_2", "Layer_3", "Layer_4", "Layer_5", "Layer_6", "SampleAttribs_1.ozPerYd2", "SampleAttribs_2.ozPerYd2", "SampleAttribs_3.ozPerYd2", "SampleAttribs_4.ozPerYd2", "SampleAttribs_5.ozPerYd2", "SampleAttribs_6.ozPerYd2": Value Change {
        n244 = event-data() -> ()  [unwired: 2 out]
        n245 = global read "BIMS_Collector Globals.vi" "SampleAttribs"() -> (w413:T29)
        n246 = Build Array("Layer_1", "Layer_2", "Layer_3", "Layer_4", "Layer_5", "Layer_6") -> (w415:T30)
        n247 = global write "BIMS_Collector Globals.vi" "LayerSpecs"(w415) -> ()
        n248 = for {
          tunnel: w415 -> [w442] mode=indexing
          shift-right: [w444] -> w423
          shift-left: 0 -> [w443]
          tunnel: [w441] -> w433 mode=indexing
          tunnel: w413 -> [w439] mode=indexing
          n249 = Unbundle By Name(w439) -> ("ozPerYd2"=w435:string)
          n250 = Equal?(x=w435, y="" ("Empty String Constant")) -> (x = y?=w434:bool)
          n251 = case shown="False" w434 {
            tunnel: [w448 sgl 0.0 ("default value 1")] -> w438
            tunnel: w435 -> [w445 _]
            frame False {
              n252 = Scan From String(format string="%f", input string=w445, default 1=sgl 0.0 ("default value 1")) -> (output 1=w448:sgl)  [unwired: 2 in, 3 out]
            }
            frame True {
            }
          }
          n253 = Unbundle By Name(w442) -> ("plyNum"=w440:i32)
          n254 = Add(x=w443, y=w440) -> (x+y=w444:i32)
          n255 = To Single Precision Float(number=w440) -> (single precision float=w437:sgl)
          n256 = Multiply(x=w437, y=w438) -> (x*y=w441:sgl)
        }
        "totalNumLayers" <- w423
        n257 = Divide(x=w433, y=sgl 144.0) -> (x/y=w431:sgl[])
        n258 = Index Array(array=w431) -> (element #1=→"fab1_totalWt":sgl, element #2=→"fab2_totalWt":sgl, element #3=→"fab3_totalWt":sgl, element #4=→"fab4_totalWt":sgl, element #5=→"fab5_totalWt":sgl, element #6=→"fab6_totalWt":sgl)  [unwired: 6 in]
        n259 = Add Array Elements(numeric array=w431) -> (sum=→"totalBAW":sgl)
      }
      event "clayCalArray": Value Change {
        n260 = event-data() -> ()  [unwired: 2 out]
        n261 = for {
          tunnel: "clayCalArray" -> [w476] mode=indexing
          shift-right: [w475] -> w458
          shift-left: "" ("Empty String Constant") -> [w473]
          shift-right: [w470] -> w454
          shift-left: i16[] [] -> [w469]
          n262 = Greater Than 0?(x=w476) -> (x > 0?=w477:bool)
          n263 = case shown="False" w477 {
            tunnel: w476 -> [_ w483]
            tunnel: ["##" ("clayCalib") w485] -> w474
            tunnel: w473 -> [w480 w484]
            tunnel: [w480 w484] -> w472
            tunnel: [w478 w482] -> w470
            tunnel: w469 -> [w478 w481]
            frame False {
            }
            frame True {
              n264 = Format Into String(w483) -> (resulting string=w485:string)  [unwired: 3 in, 1 out]
              n265 = Build Array (concatenate)(w481, w483) -> (w482:i16[])
            }
          }
          n266 = Concatenate Strings(w472, w474, "-" ("string")) -> (w475:string)
        }
        n267 = String Length(string=w458) -> (length=w459:i32)
        n268 = Add Array Elements(numeric array=w454) -> (sum=w463:i16)
        n269 = Array Size(array=w454) -> (size(s)=w464:i32)
        n270 = Decrement(x=w459) -> (x-1=w456:i32)
        n271 = To Single Precision Float(number=w463) -> (single precision float=w462:sgl)
        n272 = To Single Precision Float(number=w464) -> (single precision float=w452:sgl)
        n273 = String Subset(string=w458, length (rest)=w456) -> (substring=w457:string)  [unwired: 1 out]
        n274 = Equal To 0?(x=w452) -> (x = 0?=w451:bool)
        n275 = local write "clayCalib"(w457) -> ()
        n276 = case shown="True" w451 {
          tunnel: w462 -> [w467 w468]
          tunnel: w452 -> [w466 _]
          tunnel: [w465 w468] -> w461
          frame False {
            n277 = Divide(x=w467, y=w466) -> (x/y=w465:sgl)
          }
          frame True {
          }
        }
        "clayAverage" <- w461
      }
      event "reportV50_History": Value Change {
        n278 = event-data() -> ()  [unwired: 2 out]
        n279 = local write "lookupRec"(TRUE ("lookupRec")) -> ()
      }
      event "Methods": Value Change {
        n280 = event-data() -> ("CtlRef"=w496:refnum<vi>)  [unwired: 1 out]
        n281 = call "Dropdown Selection (SubVI).vi"("reference"=w496) -> ("element"=w495:string)
        n282 = Equal?(x=w495, y="V50") -> (x = y?=w489:bool)
        n283 = property on="minV50" class="DigNum (strict)"(error in=w493, "Visible"=w489) -> (error out=w492:errorcluster)  [unwired: 1 in, 1 out]
        n284 = Select(t=enum32{"V50", "NIJ"}."V50" ("reportType"), s=w489, f=enum32{"V50", "NIJ"}."NIJ") -> (s? t:f=w490:enum32{"V50", "NIJ"})
        n285 = local write "reportType"(w490) -> ()
      }
      event "rangeSetup": Value Change {
        n286 = event-data() -> ("NewVal"=w505:u16)  [unwired: 1 out]
        n287 = case shown="2" w505 {
          tunnel: ["0" ("section") "5.0" ("section") "7.5" ("section") "45.0" ("section")] -> w511
          frame 0, Default {
          }
          frame 1 {
          }
          frame 2 {
          }
          frame 3 {
          }
        }
        n288 = local read "configPath"() -> (w513:path)
        n289 = local read "GrainSize"() -> (w504:u16)
        n290 = Greater Than 0?(x=w505) -> (x > 0?=w508:bool)
        n291 = Greater Than 0?(x=w504) -> (x > 0?=w506:bool)
        n292 = call <vilib>:"Open Config Data (compatibility).vi"("error in (no error)"=w501, "configuration file path"=w513) -> ("error out"=w521:errorcluster, "refnum"=w523:T31)  [unwired: 7 in, 1 out]
        n293 = And(x=w508, y=w506) -> (x .and. y?=w507:bool)
        n294 = call-poly <vilib>:"Write Key.vi"("write raw string? (F)"=TRUE, "section"="Ballistic Parameters", "error in (no error)"=w521, "value"=w511, "key"="MidPoint To Target Distance", "refnum"=w523) -> ("error out"=w520:errorcluster, "refnum out"=w519:T31)  [unwired: 4 out]
        n295 = call <vilib>:"Close Config Data.vi"("error in (no error)"=w520, "refnum"=w519) -> ("error out"=w512:errorcluster)  [unwired: 1 in, 8 out]
        n296 = Not(x=w507) -> (.not. x?=w517:bool)
        n297 = Select(t=u8 0 ("y"), s=w507, f=u8 2 ("y")) -> (s? t:f=w503:u8)
        n298 = Scan From String(input string=w511, error in=w512, default 1=sgl 0.0 ("default value 1")) -> (error out=w500:errorcluster, output 1=w510:sgl)  [unwired: 2 in, 2 out]
        n299 = local write "mid_to_targ_dist"(w510) -> ()
        n300 = property on="ARM" class="Bool"(error in=w500, "Disabled"=w503) -> (error out=w499:errorcluster)  [unwired: 1 in, 1 out]
        n301 = property on="addShot" class="Bool"(error in=w499, "Disabled"=w503) -> (error out=w498:errorcluster)  [unwired: 1 in, 1 out]
        n302 = property on="instruct_addShot" class="Str"(error in=w498, "Visible"=w517) -> (error out=w497:errorcluster)  [unwired: 1 in, 1 out]
        "instruct_addShot" <- "RANGE SETUP and THREAT must be selected before shots can be added." ("instruct_addShot")
      }
      event "Drag Corrected", "maxDev": Value Change {
        n303 = event-data() -> ()  [unwired: 2 out]
        n304 = local write "processShots"(TRUE ("ProcessShots")) -> ()
      }
      event "2ndScreen": Value Change {
        n305 = event-data() -> ()  [unwired: 7 out]
        n306 = Select(t=T16."Enabled" ("Disabled"), s="2ndScreen", f=T16."Disabled and Grayed Out" ("Disabled")) -> (s? t:f=w531:T16)
        n307 = property on="Redundant/speed" class="DigNum (strict)"("DisabledEnum"=w531) -> ()  [unwired: 2 in, 2 out]
        n308 = property on="MeasVelScrnSet2" class="DigNum (strict)"("DisabledEnum"=w531) -> ()  [unwired: 2 in, 2 out]
      }
      event "MC Listbox of Shots": Mouse Up {
        n309 = event-data() -> ()  [unwired: 2 out]
        n310 = flat-sequence {
          tunnel: w539 -> [w543]
          tunnel: [w541] -> w538
          tunnel: ["MC Listbox of Shots"] -> w535
          tunnel: w538 -> [w547]
          tunnel: [w546] -> w537
          tunnel: w535 -> [_]
          tunnel: w537 -> [w552]
          tunnel: [w550] -> w536
          frame #0 {
            n311 = property on="Table of Shots" class="Tbl (strict)"(error in=w543) -> (error out=w542:errorcluster, "Value"=w544:string[][])  [unwired: 1 in, 1 out]
            n312 = local write "STOP (Shots MC LB)"(FALSE ("STOP (Shots MC LB)")) -> ()
            n313 = property on="MC Listbox of Shots" class="MCListbox (strict)"(error in=w542, "ItemNames"=w544) -> (error out=w541:errorcluster)  [unwired: 1 in, 1 out]
          }
          frame #1 {
            n314 = control-ref of="MC Listbox of Shots"() -> (w549:refnum<vi>)
            n315 = control-ref of="STOP (Shots MC LB)"() -> (w548:refnum<vi>)
            n316 = call "multicolumn listbox sort.vi"("error IN"=w547, "Bool Refnum"=w548, "MCListbox Refnum"=w549) -> ("error out"=w546:errorcluster)  [unwired: 4 in]
          }
          frame #2 {
            n317 = property on="MC Listbox of Shots" class="MCListbox (strict)"(error in=w552) -> (error out=w551:errorcluster, "ItemNames"=w553:string[][])  [unwired: 1 in, 1 out]
            n318 = property on="Table of Shots" class="Tbl (strict)"(error in=w551, "Val(Sgnl)"=w553) -> (error out=w550:errorcluster)  [unwired: 1 in, 1 out]
          }
        }
      }
      event "PublishNewRecords": Value Change {
        w559 = "\\" ("string")
        w569 = TRUE  # overwrite (F)
        # "2. INSERT new records to Experiments and  \n      Shots tables in local Export.mdb file."
        # "1. SELECT new records from local MDB \n     by comparing against last record numbers \n     found in IMPORT table on BIMS server."
        # "Pushes latest ballistics performance data up to BIMS Server\n\n - Attempts connection with server (reports connection success in msgbox)\n - If successful:\n   - Exports all experiment/shot records since last table marker to [site].mdb file\n   - Sends export.mdb file to drop location on BIMS File Server\n   - Executes SSIS package to import records from export.mdb file\n - Otherwise provides option to try again or cancel"
        # "3. Copy Export.mdb file to [sitename].mdb in [sitename] \n      FileDrop folder on BIMS server."
        n319 = event-data() -> ()  [unwired: 2 out]
        n320 = property on="Loading" class="Ring (strict)"(error in=w565, "Visible"=TRUE) -> (error out=w564:errorcluster)  [unwired: 1 in, 1 out]
        n321 = local read "Site"() -> (w554:string)
        n322 = call "Export New Records.vi"("error IN"=w564, "Site"=w554) -> ("error out"=w571:errorcluster)  [unwired: 3 in, 6 out]
        n323 = Concatenate Strings("\\\\" ("string"), "Server", w559, "Folder", w559, w554, ".mdb" ("string")) -> (w555:string)
        n324 = String To Path(string=w555) -> (path=w567:path)
        n325 = Copy(8:w571, 9:w569, 10:w567, 11:path "C:/Ballistics/Export.mdb" ("source path")) -> (0:w568:errorcluster)  [unwired: 3 out]
        n326 = case shown="No Error" w568 {
          selector: w568 -> [w573 w575]
          tunnel: [w573 w574] -> w563
          frame No Error {
            n327 = One Button Dialog(message="New sample performance records submitted \nto BIMS Warehouse successfully.\n\nPublishing will occur in under five minutes.") -> ()  [unwired: 2 out]
          }
          frame Error {
            n328 = call <vilib>:"General Error Handler.vi"("error in (no error)"=w575) -> ("error out"=w574:errorcluster)  [unwired: 2 in, 12 out]
          }
        }
        n329 = property on="Loading" class="Ring (strict)"(error in=w563, "Visible"=FALSE) -> (error out=w562:errorcluster)  [unwired: 1 in, 1 out]
      }
      event "arrIDC": Mouse Up {
        n330 = event-data() -> ()  [unwired: 2 out]
        "velProfile" <- cluster{dbl, dbl}[] [] ("velProfile")
        "arrIDC" <- dbl[] [] ("arrIDC")
        "relativeTime" <- cluster{"ts2":dbl, "ts3":dbl, "ts1":dbl} {"ts2"=0.0, "ts3"=0.0, "ts1"=0.0} ("relativeTime")
        "velMeasProf" <- T8 {"v2"=0.0, "vB"=0.0, "vOuter"=0.0, "v1"=0.0, "vA"=0.0, "vInner"=0.0} ("velMeasProf")
        "velCompProf" <- cluster{"vStrike":dbl, "vA":dbl} {"vStrike"=0.0, "vA"=0.0} ("velCompProf")
        "displacement" <- T9 {"ds_v2"=6.75, "ds2"=5.0833, "ds_vB"=4.9167, "ds3"=4.75, "ds_vAvg"=6.9167, "ds_v1"=7.0833, "ds1"=8.75, "ds_vA"=8.9167, "ds0"=9.0833} ("displacement")
      }
      event "SampleBackings": Value Change {
        # "Clay is the default sample backing material.\n\n  If another selection is made, then grey out and disable all controls relating to clay."
        n331 = event-data() -> ()  [unwired: 2 out]
        n332 = case shown="2.." "SampleBackings" {
          tunnel: [T16."Disabled and Grayed Out" ("Disabled") T16."Enabled" ("Disabled") T16."Disabled and Grayed Out" ("Disabled")] -> w583
          frame 0, Default {
          }
          frame 1 {
          }
          frame 2.. {
          }
        }
        n333 = property on="clayCalArray" class="Arr (strict)"("DisabledEnum"=w583) -> ()  [unwired: 2 in, 2 out]
        n334 = property on="clayAverage" class="DigNum (strict)"("DisabledEnum"=w583) -> ()  [unwired: 2 in, 2 out]
        n335 = property on="clayTemp" class="DigNum (strict)"("DisabledEnum"=w583) -> ()  [unwired: 2 in, 2 out]
      }
      event "btnScrnSets": Value Change {
        n336 = event-data() -> ()  [unwired: 2 out]
        n337 = Bundle("screenSet_1"="screenSet_1", "screenSet_2"="screenSet_2") -> (w590:cluster{"screenSet_1":sgl, "screenSet_2":sgl})  [unwired: 1 in]
        n338 = local read "configPath"() -> (w589:path)
        n339 = call "Write Parameters.vi"("error in (no error)"=w594, "rangeParams"=w590, "appended path"=w589) -> ("error out"=w593:errorcluster)  [unwired: 4 in]
        n340 = case shown="No Error" w593 {
          tunnel: "screenSet_1" -> [w598 _]
          tunnel: "screenSet_2" -> [w597 _]
          frame No Error {
            n341 = Format Into String(format string="Updated Screen Separations\n                (meters)\n\n       Set #1: %.3f\n       Set #2: %.3f", w598, w597) -> (resulting string=w596:string)  [unwired: 2 in, 1 out]
            n342 = One Button Dialog(message=w596) -> ()  [unwired: 1 in, 1 out]
          }
          frame Error {
          }
        }
      }
      event "RefreshMetadata": Value Change {
        # "Pulls latest metadata down from BIMS Database Server\n - Attempts connection with server \n        (reports failure if connection is unsuccessful)\n - If successful:\n   - Updates local database records from server\n   - Updates dropdown listboxes from local database"
        n343 = event-data() -> ()  [unwired: 2 out]
        n344 = Initialize Array(T4 {"plyNum"=0, "LotNum"="-", "RollNum"="-"} ("Layer_1"), 6 ("dimension size")) -> (w609:T30)
        n345 = property on="Loading" class="Ring (strict)"(error in=w637, "Visible"=TRUE) -> (error out=w636:errorcluster)  [unwired: 1 in, 1 out]
        n346 = control-ref of="LayerStitchTypes"() -> (w622:refnum<vi>)
        n347 = control-ref of="BackLayer"() -> (w632:refnum<vi>)
        n348 = control-ref of="FrontLayer"() -> (w633:refnum<vi>)
        n349 = control-ref of="ThreatGroups"() -> (w634:refnum<vi>)
        n350 = control-ref of="SampleClamping"() -> (w641:refnum<vi>)
        n351 = control-ref of="SampleTypes"() -> (w658:refnum<vi>)
        n352 = control-ref of="SampleDimensions"() -> (w657:refnum<vi>)
        n353 = control-ref of="ModelMfrs"() -> (w656:refnum<vi>)
        n354 = control-ref of="Assemblers"() -> (w655:refnum<vi>)
        n355 = control-ref of="Submitters"() -> (w654:refnum<vi>)
        n356 = control-ref of="PowderTypes"() -> (w653:refnum<vi>)
        n357 = control-ref of="Methods"() -> (w650:refnum<vi>)
        n358 = control-ref of="TestConditions"() -> (w649:refnum<vi>)
        n359 = control-ref of="SampleBackings"() -> (w648:refnum<vi>)
        n360 = control-ref of="Ballisticians"() -> (w647:refnum<vi>)
        n361 = control-ref of="Shooters"() -> (w646:refnum<vi>)
        n362 = control-ref of="Recorders"() -> (w645:refnum<vi>)
        n363 = global write "BIMS_Collector Globals.vi" "LayerSpecs"(w609) -> ()
        n364 = control-ref of="SampleCoverings"() -> ()  [unwired: 1 out]
        n365 = Build Array(w622, w632, w633, w634, w641, w658, w657, w656, w655, w654, w653, w650, w649, w648, w647, w646, w645) -> (w652:refnum<vi>[])
        n366 = Index Array(array=w609) -> (element #1=w610:T4, element #2=w608:T4, element #3=w607:T4, element #4=w606:T4, element #5=w605:T4, element #6=w604:T4)  [unwired: 8 in, 2 out]
        n367 = control-ref of="loadStatus"() -> (w616:refnum<vi>)
        n368 = local write "Layer_1"(w610) -> ()
        n369 = local write "Layer_2"(w608) -> ()
        n370 = local write "Layer_3"(w607) -> ()
        n371 = local write "Layer_4"(w606) -> ()
        n372 = local write "Layer_5"(w605) -> ()
        n373 = local write "Layer_6"(w604) -> ()
        n374 = call "Update Metadata using listbox names.vi"("loadStatus Refnum"=w616, "error in"=w636, "Site"="Site", "RefNumArrIn"=w652) -> ("error out"=w614:errorcluster, "RefNumArrOut"=w651:refnum<vi>[])  [unwired: 6 out]
        n375 = control-ref of="ProjectID_0"() -> (w599:refnum<vi>)
        n376 = control-ref of="ThreatSize_0"() -> (w618:refnum<vi>)
        n377 = control-ref of="Requestors_0"() -> (w621:refnum<vi>)
        n378 = call "Fill Lists from DB (1st Pass).vi"("error in"=w614, "RefNumArray"=w651) -> ("error out"=w603:errorcluster)  [unwired: 1 in, 4 out]
        n379 = flat-sequence {
          frame #0 {
            n380 = local write "RefreshMetadata"(FALSE ("UpdateMetadata")) -> ()
            n381 = local write "TimeNow"("Loading from BIMS Server . . ." ("TimeNow")) -> ()
          }
        }
        n382 = call "Fill Stitch Lists.vi"("error IN"=w603) -> ("error OUT"=w602:errorcluster)  [unwired: 6 in]
        n383 = Build Array(w599, w618, w621) -> (w620:refnum<vi>[])
        n384 = call "Fill Lists from DB (2nd Pass).vi"("errorIN"=w602, "colNames"=string[] ["ProjectID", "GrainSize", "requestor"] ("lkupTableNames"), "lkupTableNames"=string[] ["Experiments", "ThreatDetails", "Submitters"], "RefNumArray"=w620) -> ("error OUT"=w600:errorcluster)  [unwired: 3 in]
        n385 = property class="Str"(reference=w616, error in=w614, "Value"="filling dropdown lists") -> (reference out=w615:refnum<vi>)  [unwired: 1 out]
        n386 = property on="LayerStitchTypes" class="Ring (strict)"(error in=w600) -> ("Strings []"=w601:string[])  [unwired: 1 in, 2 out]
        n387 = call "Create local tables from Server DB.vi"("loadStatus Refnum"=w615, "error in"=w600, "Site"="Site", "tableNames"=string[] ["Threats", "ThreatDetails", "ThreatCalibers", "Mfrs", "SampleStyles", "SampleSpecs", "FiberTypes"]) -> ("error out"=w643:errorcluster)  [unwired: 7 out]
        n388 = call "Fill Lists From DB (3rd Pass).vi"("error IN"=w643) -> ("error OUT"=w624:errorcluster)  [unwired: 3 in, 3 out]
        n389 = property on="layerStitch_1" class="Ring (strict)"("Strings []"=w601) -> ()  [unwired: 2 in, 2 out]
        n390 = property on="layerStitch_2" class="Ring (strict)"("Strings []"=w601) -> ()  [unwired: 2 in, 2 out]
        n391 = property on="layerStitch_3" class="Ring (strict)"("Strings []"=w601) -> ()  [unwired: 2 in, 2 out]
        n392 = property on="layerStitch_4" class="Ring (strict)"("Strings []"=w601) -> ()  [unwired: 2 in, 2 out]
        n393 = property on="layerStitch_5" class="Ring (strict)"("Strings []"=w601) -> ()  [unwired: 2 in, 2 out]
        n394 = property on="layerStitch_6" class="Ring (strict)"("Strings []"=w601) -> ()  [unwired: 2 in, 2 out]
        n395 = control-ref of="ModelMfrs"() -> (w631:refnum<vi>)
        n396 = property class="Ring (strict)"(reference=w631, error in=w624) -> (reference out=w630:refnum<vi>, error out=w629:errorcluster, "Strings []"=w628:string[])
        n397 = Delete From Array(array=w628, length=1, index=0) -> (array with subset deleted=w627:string[])  [unwired: 1 out]
        n398 = property class="Ring (strict)"(reference=w630, error in=w629, "Strings []"=w627) -> (error out=w623:errorcluster)  [unwired: 1 out]
        n399 = case shown="No Error" w623 {
          selector: w623 -> [w660 w663]
          tunnel: [w660 w663] -> w640
          frame No Error {
            n400 = local write "TimeNow"("Collector Metadata is READY!" ("TimeNow")) -> ()
            n401 = Wait (ms)(milliseconds to wait=u32 2000) -> ()  [unwired: 1 out]
            "loadStatus" <- ""
          }
          frame Error {
            n402 = call <vilib>:"General Error Handler.vi"("error in (no error)"=w663) -> ()  [unwired: 2 in, 13 out]
          }
        }
        n403 = property on="Loading" class="Ring (strict)"(error in=w640, "Visible"=FALSE) -> (error out=w639:errorcluster)  [unwired: 1 in, 1 out]
      }
      event "loadingUnits": Value Change {
        n404 = local read "Powder Loading"() -> (w667:sgl)
        n405 = event-data() -> ("NewVal"=w666:enum32{"grams", "grains"})  [unwired: 6 out]
        n406 = case shown="\"grams\", Default" w666 {
          tunnel: w667 -> [w671 w672]
          frame "grams", Default {
            n407 = Multiply(x=w671, y=sgl 0.06479891) -> (x*y=w669:sgl)
            n408 = local write "Powder Loading"(w669) -> ()
          }
          frame "grains" {
            n409 = Multiply(x=w672, y=sgl 15.432359) -> (x*y=w673:sgl)
            n410 = local write "Powder Loading"(w673) -> ()
          }
        }
      }
      event "clearErrors": Value Change {
        w675 = errorcluster {"status"=FALSE, "code"=0, "source"=""} ("error in")
        n411 = event-data() -> ()  [unwired: 7 out]
        n412 = local write "SMErr"(w675) -> ()
      }
    }
    "U/I EvErr" <- w31
  }
  n413 = while "Test Executive State Machine" {
    shift-left: 100 -> [w684]
    shift-right: [w685] -> _
    shift-left: Collector_State."INITIALIZE" ("progState") -> [w681]
    shift-right: [w678] -> _
    shift-right: [w682] -> _
    shift-left: w26 -> [w683]
    shift-right: [w679] -> _
    shift-left: w22 -> [w680]
    tunnel: w3 -> [w676]
    stop <- FALSE stop-if-true
    n414 = case shown="\"V50 Report or GET Record\"" w681 {
      tunnel: [w705 w817 Collector_State."POLL" ("progState") Collector_State."POLL" ("progState") w1852 Collector_State."PROC SHOTS" ("progState") Collector_State."POLL" ("progState") Collector_State."PROC SHOTS" ("progState") Collector_State."PROC SHOTS" ("progState") Collector_State."POLL" ("progState") Collector_State."POLL" ("progState") w2457] -> w678
      tunnel: [-1 -1 ("index of element") -1 ("index of element") -1 ("index of element") w1851 -1 ("index of element") -1 -1 ("index of element") -1 ("index of element") -1 -1 ("index of element") w2456] -> w685
      tunnel: w684 -> [_ w818 _ _ _ _ _ _ _ _ _ _]
      tunnel: w683 -> [w708 w816 w972 w1600 w1846 w2085 w2127 w2137 w2155 w2206 w2220 w2458]
      tunnel: [w700 w815 w972 w1600 w1845 w2071 w2131 w2137 w2152 w2206 w2224 w2458] -> w682
      tunnel: w680 -> [_ w811 w969 w1598 w1848 w2081 w2123 w2140 w2151 w2203 w2219 w2450]
      tunnel: [w711 w812 w968 w1597 w1847 w2079 w2123 w2138 w2150 w2202 w2218 w2455] -> w679
      tunnel: w676 -> [_ _ _ _ _ _ _ _ _ _ _ w2449]
      frame "POLL", Default {
        w709 = Collector_State."POLL"  # progStateType
        w721 = TRUE  # element
        w724 = 4  # SAVE
        # "case # 0"
        # "This section checks for any buttons, maintains routine check of the parameters"
        n415 = case shown="\"Measure\"" "mainTabCntrl" {
          frame "Setup", Default {
            n416 = control-ref of="layerStitch_1"() -> (w741:refnum<vi>)
            n417 = control-ref of="layerStitch_2"() -> (w740:refnum<vi>)
            n418 = control-ref of="layerStitch_3"() -> (w739:refnum<vi>)
            n419 = control-ref of="layerStitch_4"() -> (w738:refnum<vi>)
            n420 = control-ref of="layerStitch_5"() -> (w737:refnum<vi>)
            n421 = control-ref of="layerStitch_6"() -> (w736:refnum<vi>)
            n422 = control-ref of="SampleStyle_0"() -> (w734:refnum<vi>)
            n423 = control-ref of="SampleStyle_1"() -> (w755:refnum<vi>)
            n424 = control-ref of="SampleStyle_2"() -> (w756:refnum<vi>)
            n425 = control-ref of="SampleStyle_3"() -> (w757:refnum<vi>)
            n426 = control-ref of="SampleStyle_4"() -> (w758:refnum<vi>)
            n427 = control-ref of="SampleStyle_5"() -> (w759:refnum<vi>)
            n428 = control-ref of="SampleStyle_6"() -> (w760:refnum<vi>)
            n429 = Build Array(w741, w740, w739, w738, w737, w736) -> (w742:refnum<vi>[])
            n430 = global write "BIMS_Collector Globals.vi" "LayerStitchTypeRefs"(w742) -> ()
            n431 = Build Array(w734, w755, w756, w757, w758, w759, w760) -> (w753:refnum<vi>[])
            n432 = global write "BIMS_Collector Globals.vi" "SampleStyles"(w753) -> ()
            n433 = local read "Fabric Description"() -> (w745:string)
            n434 = control-ref of="Mfr_0"() -> (w735:refnum<vi>)
            n435 = control-ref of="Mfr_1"() -> (w766:refnum<vi>)
            n436 = control-ref of="Mfr_2"() -> (w765:refnum<vi>)
            n437 = control-ref of="Mfr_3"() -> (w764:refnum<vi>)
            n438 = control-ref of="Mfr_4"() -> (w763:refnum<vi>)
            n439 = control-ref of="Mfr_5"() -> (w762:refnum<vi>)
            n440 = control-ref of="Mfr_6"() -> (w761:refnum<vi>)
            n441 = String Subset(string=w745, length (rest)=75 ("length (rest)")) -> (substring=w744:string)  [unwired: 1 out]
            n442 = Build Array(w735, w766, w765, w764, w763, w762, w761) -> (w754:refnum<vi>[])
            n443 = local write "Fabric Description"(w744) -> ()
            n444 = global write "BIMS_Collector Globals.vi" "Mfrs"(w754) -> ()
            n445 = local read "SampleAttribs_1"() -> (w747:T3)
            n446 = local read "SampleAttribs_2"() -> (w749:T3)
            n447 = local read "SampleAttribs_3"() -> (w750:T3)
            n448 = local read "SampleAttribs_4"() -> (w751:T3)
            n449 = local read "SampleAttribs_5"() -> (w752:T3)
            n450 = local read "SampleAttribs_6"() -> (w748:T3)
            n451 = Build Array(w747, w749, w750, w751, w752, w748) -> (w746:T35)
            n452 = global write "BIMS_Collector Globals.vi" "SampleAttribs"(w746) -> ()
          }
          frame "Measure" {
            # "Disable and gray out the \"Save\" button\nIF the shot table has no shots, \nOR if there are no plies; otherwise, enable it."
            # "Disable and gray out the \"Clear Shots\" button\nIF the shot table has no shots; otherwise, enable it."
            n453 = local read "shotsArr"() -> (w771:T6)
            n454 = local read "totalNumLayers"() -> (w769:i32)
            n455 = Equal To 0?(x=w769) -> (x = 0?=w770:bool)
            n456 = Array Size(array=w771) -> (size(s)=w781:i32)
            n457 = Equal To 0?(x=w781) -> (x = 0?=w768:bool)
            n458 = Or(x=w768, y=w770) -> (x .or. y?=w767:bool)
            n459 = property on="saveReq" class="Str"("Visible"=w767) -> ()  [unwired: 2 in, 2 out]
            n460 = Select(t=T16."Disabled and Grayed Out" ("Disabled"), s=w767, f=T16."Enabled" ("Disabled")) -> (s? t:f=w772:T16)
            n461 = Select(t=T16."Disabled and Grayed Out" ("Disabled"), s=w768, f=T16."Enabled" ("Disabled")) -> (s? t:f=w780:T16)
            n462 = property on="reportV50" class="Bool"("Disabled"=w772) -> ()  [unwired: 2 in, 2 out]
            n463 = property on="saveShots" class="Bool"("Disabled"=w772) -> ()  [unwired: 2 in, 2 out]
            n464 = property on="clearShots" class="Bool"("Disabled"=w780) -> ()  [unwired: 2 in, 2 out]
            n465 = local read "Shot Description"() -> (w779:string)
            n466 = String Subset(string=w779, length (rest)=30 ("length (rest)")) -> (substring=w777:string)  [unwired: 1 out]
            n467 = local write "Shot Description"(w777) -> ()
          }
          frame "History" {
          }
          frame "System" {
          }
        }
        n468 = Format Date/Time String(time format string (%c)="%x   %H:%M:%S") -> (date/time string=w697:string)  [unwired: 2 out]
        n469 = local write "shotTimestamp"(w697) -> ()
        n470 = Or(x="undoLastShot", y="deleteShot") -> (x .or. y?=w719:bool)
        n471 = Or(x="reportV50", y="reportV50_History") -> (x .or. y?=w727:bool)
        n472 = flat-sequence {
          tunnel: [w788] -> w710
          frame #0 {
            n473 = Wait (ms)(milliseconds to wait=u32 10 ("millisecond timer value")) -> ()  [unwired: 1 out]
          }
          frame #1 {
            n474 = local read "SMErr"() -> (w788:errorcluster)
          }
        }
        n475 = Build Array("RESET All", w727, "VsVr Report", "saveShots", "addShot", "clearShots", "nextShot", w719, "readyClock", "processShots") -> (w722:bool[])
        n476 = Search 1D Array(1D array=w722, element=w721) -> (index of element=w732:i32)  [unwired: 1 out]
        n477 = Increment(x=w732) -> (x+1=w733:i32)
        n478 = Equal?(x=w733, y=w724) -> (x = y?=w725:bool)
        n479 = case shown="False" w725 {
          tunnel: w733 -> [w790 w802]
          tunnel: [w791 w807] -> w731
          tunnel: w710 -> [w789 w798]
          tunnel: [w789 w796] -> w711
          frame False {
            w793 = 0  # Not Found
            n480 = Equal?(x=w790, y=w793) -> (x = y?=w792:bool)
            n481 = case shown="False" w792 {
              tunnel: w790 -> [w794 _]
              tunnel: [w794 w795] -> w791
              frame False {
              }
              frame True {
                w795 = 11  # CheckDAQ
                # "USUAL SCENARIO"
              }
            }
          }
          frame True {
            # "Before allowing data record to be saved,\nprompt user to validate."
            n482 = call "Get Last Record (SubVI).vi"("error in"=w798) -> ("error out"=w797:errorcluster, "experiment record"=w799:i32, "shot record"=w800:i32)  [unwired: 2 out]
            n483 = local write "lastSamp"(w799) -> ()
            n484 = local write "lastShot"(w800) -> ()
            n485 = To Double Precision Float(number=w799) -> (double precision float=w801:dbl)
            n486 = Two Button Dialog(message="Are ALL Data Valid?", 1:"NO" ("F button name (\"Cancel\")"), 2:"YES" ("T button name (\"OK\")")) -> (T button?=w806:bool)
            n487 = property on="Record #" class="DigNum (strict)"(error in=w797, "Maximum"=w801) -> (error out=w796:errorcluster)  [unwired: 1 in, 1 out]
            n488 = case shown="False" w806 {
              tunnel: [0 ("index of element") w809] -> w807
              tunnel: w802 -> [_ w809]
              frame False {
                # "POLL"
              }
              frame True {
              }
            }
          }
        }
        n489 = local read "shotsArr"() -> (w700:T6)
        n490 = for {
          tunnel: w708 -> [w785] mode=indexing
          tunnel: w700 -> [w786] mode=indexing
          tunnel: [w782] -> w707 mode=indexing
          n491 = Not Equal?(x=w786, y=w785) -> (x != y?=w784:T36)
          n492 = Cluster To Array(cluster=w784) -> (array=w783:bool[])
          n493 = Or Array Elements(Boolean array=w783) -> (logical OR=w782:bool)
        }
        n494 = Or Array Elements(Boolean array=w707) -> (logical OR=w703:bool)
        n495 = To Variant(anything=w731) -> (Variant=w730:variant)
        n496 = Variant To Data(type=w709, Variant=w730) -> (data=w706:T14)  [unwired: 1 in, 1 out]
        n497 = Select(t=Collector_State."PROC SHOTS" ("progStateType"), s=w703, f=w706) -> (s? t:f=w705:T14)
        "STOP (Shots MC LB)" <- TRUE ("STOP (Shots MC LB)")
      }
      frame "INITIALIZE" {
        # "case # 1"
        # "This section reads the ini file"
        n498 = case shown="100" w818 {
          tunnel: [w824 w843] -> w819
          tunnel: [w822 w843] -> w814
          tunnel: w811 -> [w821 w835]
          tunnel: [w820 w835] -> w810
          frame 0, Default {
            n499 = local read "RESET All"() -> (w823:bool)
            n500 = case shown="False" w823 {
              tunnel: [TRUE w831] -> w824
              tunnel: [FALSE w831] -> w822
              tunnel: w821 -> [w825 w828]
              tunnel: [w825 w828] -> w820
              frame False {
                # "Refresh"
              }
              frame True {
                n501 = Two Button Dialog(message="Resetting will remove all unsaved data.\n\nDo you really  want to reset? ", 1:"NO" ("F button name (\"Cancel\")"), 2:"YES" ("T button name (\"OK\")")) -> (T button?=w831:bool)
              }
            }
          }
          frame 100 {
            w843 = TRUE  # Reset ALL
            n502 = control-ref of="Mfr_0"() -> (w833:refnum<vi>)
            n503 = control-ref of="Mfr_1"() -> (w842:refnum<vi>)
            n504 = control-ref of="Mfr_2"() -> (w841:refnum<vi>)
            n505 = control-ref of="Mfr_3"() -> (w840:refnum<vi>)
            n506 = control-ref of="Mfr_4"() -> (w839:refnum<vi>)
            n507 = control-ref of="Mfr_5"() -> (w838:refnum<vi>)
            n508 = control-ref of="Mfr_6"() -> (w837:refnum<vi>)
            n509 = property on="Loading" class="Ring (strict)"("Visible"=FALSE) -> ()  [unwired: 2 in, 2 out]
            n510 = Build Array(w833, w842, w841, w840, w839, w838, w837) -> (w836:refnum<vi>[])
            n511 = global write "BIMS_Collector Globals.vi" "Mfrs"(w836) -> ()
          }
        }
        n512 = case shown="True" w819 {
          tunnel: [Collector_State."POLL" ("progState") w885] -> w817
          tunnel: w816 -> [w846 _]
          tunnel: [w846 "shotsArr"] -> w815
          tunnel: w814 -> [_ w886]
          tunnel: [w844 w855] -> w812
          tunnel: w810 -> [w844 w884]
          frame False {
            n513 = local write "RESET All"(FALSE ("RESET")) -> ()
          }
          frame True {
            n514 = case shown="True" w886 {
              selector: w886 -> [_ w912]
              tunnel: [w895 w912] -> w867
              tunnel: [w894 w927] -> w851
              tunnel: w884 -> [w894 w914]
              tunnel: [w893 w911] -> w857
              frame False {
                w895 = FALSE  # Reset All
                # "Refresh"
                n515 = local read "configPath"() -> (w893:path)
              }
              frame True {
                # "This section resets\nentire program"
                # "Reset ALL"
                n516 = control-ref of="This VI"() -> (w904:refnum<vi>)
                n517 = invoke on="Invoke Node" class="VI" method="Default Vals.Reinit All"(reference=w904, error in=w914) -> (reference out=w903:refnum<vi>, error out=w902:errorcluster)  [unwired: 1 in, 1 out]
                n518 = property class="VI"(reference=w903, error in=w902, "Front Panel.ShowMenuBar"=FALSE ("Front Panel Window:Show Menu Bar")) -> (reference out=w900:refnum<vi>, error out=w898:errorcluster)
                n519 = control-ref of="ScreenSetAvgg"() -> (w922:refnum<vi>)
                n520 = control-ref of="InterlockExists"() -> (w923:refnum<vi>)
                n521 = control-ref of="useBallisitican"() -> (w924:refnum<vi>)
                n522 = control-ref of="useRecorder"() -> (w925:refnum<vi>)
                n523 = control-ref of="useShooter"() -> (w926:refnum<vi>)
                n524 = control-ref of="useBMC"() -> (w897:refnum<vi>)
                n525 = property on="mainTabCntrl" class="TabCtl (strict)"() -> (error out=w906:errorcluster, "Pages"=w908:refnum<vi>[])  [unwired: 2 in, 1 out]
                n526 = Close Reference(reference=w900, error in (no error)=w898) -> (error out=w899:errorcluster)
                n527 = call "RegReadParams.vi"("ScreenSetAveraging_Ref"=w922, "useBMC_Ref"=w897, "InterlockExist_Ref"=w923, "errorIN"=w899, "useShooter_Ref"=w926, "useRecorder_Ref"=w925, "useBallistician_Ref"=w924) -> ("error out"=w921:errorcluster)  [unwired: 4 out]
                n528 = Index Array(array=w908, index=1) -> (element=w910:refnum<vi>)
                n529 = control-ref of="Server"() -> (w913:refnum<vi>)
                n530 = control-ref of="ConfigName"() -> (w917:refnum<vi>)
                n531 = control-ref of="Site"() -> (w915:refnum<vi>)
                n532 = control-ref of="Folder"() -> (w896:refnum<vi>)
                n533 = property on="Property Node" class="Page"(reference=w910, error in=w906, "PageEnb"=T17."Page Disabled & Grayed" ("Page Enabled State")) -> (error out=w905:errorcluster)  [unwired: 1 out]
                n534 = Build Array(w917, w915, w913, w896) -> (w918:refnum<vi>[])
                n535 = property on="minV50" class="DigNum (strict)"(error in=w905, "Visible"=w912) -> ()  [unwired: 1 in, 2 out]
                n536 = call "InitStringValuesFromRegistry(SubVI).vi"("error in"=w921, "String References"=w918, "subkey"="SOFTWARE\\DuPont\\BIMS-15\\Collector", "root key (HKEY_LOCAL_MACHINE)"=Registry_RtKey."HKEY_LOCAL_MACHINE") -> ("error out"=w920:errorcluster)  [unwired: 3 out]
                n537 = Current VI's Path() -> (path=w930:path)
                n538 = call "Initialize (SubVI).vi"("path"=w930, "error IN"=w920) -> ("pathConfigOUT"=w911:path, "lengthUnits"=→"lengthUnits":string, "massUnits"=→"massUnits":string, "error out"=w927:errorcluster)  [unwired: 1 out]
                "configPath" <- w911
              }
            }
            n539 = control-ref of="MeasSrc"() -> (w853:refnum<vi>)
            n540 = call "check timing board (SubVI).vi"("errIN"=w851, "ActiveDev"="ActiveDev", "measSrc_ref"=w853) -> ("error out"=w850:errorcluster, "deviceID"=→"Device S/N":string)  [unwired: 7 in]
            n541 = property on="Ballisticians" class="Ring (strict)"("Visible"="useBallisitican") -> ()  [unwired: 2 in, 2 out]
            n542 = property on="Shooters" class="Ring (strict)"("Visible"="useShooter") -> ()  [unwired: 2 in, 2 out]
            n543 = property on="Recorders" class="Ring (strict)"("Visible"="useRecorder") -> ()  [unwired: 2 in, 2 out]
            n544 = control-ref of="Threat"() -> (w870:refnum<vi>)
            n545 = control-ref of="SampleTypes"() -> (w872:refnum<vi>)
            n546 = control-ref of="SampleDescrip"() -> (w879:refnum<vi>)
            n547 = call "Get Threats (SubVI).vi"("pathConfigIN"=w857, "refThreat"=w870, "error in"=w850) -> ("pathConfigOUT"=w874:path, "factorOut"=→"factor array":sgl[], "error out"=w877:errorcluster)  [unwired: 4 out]
            n548 = Bundle("SampleTypes"=w872, "SampleDescrip"=w879) -> (w878:T37)  [unwired: 1 out]
            n549 = call "Fill Lists from INI (SubVI).vi"("clusterListboxes"=w878, "error in"=w877, "pathConfigIN"=w874) -> ("error out"=w876:errorcluster, "pathConfigOUT"=w875:path)  [unwired: 4 out]
            n550 = call "Read Parameters.vi"("error in (no error)"=w876, "appended path"=w875) -> ("error out"=w869:errorcluster, "rangeParams"=w871:T38)  [unwired: 4 out]
            n551 = Unbundle(w871) -> ("max dev"=w858:sgl, "residual separation"=→"Residual/Separation":sgl, "Set#1 Separation"=w849:sgl, "Set#2 Separation"=w848:sgl, "impact target dist"=w860:sgl, "resid target dist"=w861:sgl, "barrel screen dist"=→"Barrel to Screen":sgl, "midpt_to_target_dist"=→"mid_to_targ_dist":sgl)
            "Set#1 Separation" <- w849
            "Set#2 Separation" <- w848
            n552 = local write "maxDev"(w858) -> ()
            n553 = local write "screenSet_1"(w849) -> ()
            n554 = local write "screenSet_2"(w848) -> ()
            n555 = local write "Set#1_to_Target"(w860) -> ()
            n556 = local write "Residual/Target Dist"(w861) -> ()
            n557 = property on="RefreshMetadata" class="Bool (strict)"(error in=w869, "Val(Sgnl)"=TRUE) -> (error out=w864:errorcluster)  [unwired: 1 in, 1 out]
            n558 = case shown="True" w867 {
              tunnel: [Collector_State."POLL" ("progState") w956] -> w885
              tunnel: [w931 w937] -> w883
              tunnel: w864 -> [w931 w953]
              tunnel: w857 -> [_ w944]
              tunnel: "useBMC" -> [_ w943]
              frame False {
                # "Refresh"
              }
              frame True {
                w933 = T16."Disabled and Grayed Out" ("Disabled")
                # "Reset ALL"
                n559 = Get Date/Time In Seconds() -> (seconds since 1Jan1904=w935:timestamp)
                n560 = global read "BIMS_Collector Globals.vi" "SampleStyles"() -> (w946:refnum<vi>[])
                n561 = local read "InterlockExists"() -> (w955:bool)
                n562 = case shown="True" w943 {
                  tunnel: w944 -> [_ w958]
                  frame False {
                  }
                  frame True {
                    n563 = Path To String(path=w958) -> (string=w959:string)
                    n564 = call "Ballistics Message Center.vi"("INI File Name"=w959) -> ()
                  }
                }
                n565 = local read "MeasSrc"() -> (w957:T13)
                n566 = call "Get Last Record (SubVI).vi"("error in"=w953) -> ("error out"=w945:errorcluster, "experiment record"=w951:i32, "shot record"=→"lastShot":i32)  [unwired: 2 out]
                "lastSamp" <- w951
                n567 = control-ref of="ThreatDetails"() -> (w942:refnum<vi>)
                n568 = control-ref of="SampleStyle_0"() -> (w948:refnum<vi>)
                n569 = control-ref of="ThreatGroups"() -> (w947:refnum<vi>)
                n570 = To Double Precision Float(number=w951) -> (double precision float=w950:dbl)
                n571 = case shown="\"Screens\"" w957 {
                  tunnel: [Collector_State."POLL" ("progState") Collector_State."POLL" ("progState") Collector_State."READY CLOCK" ("progState")] -> w956
                  frame "Simulated", Default {
                  }
                  frame "Radar" {
                  }
                  frame "Screens" {
                    # "check for PCI 6602"
                  }
                }
                n572 = Build Array (concatenate)(w942, w948, w947, w946) -> (w949:refnum<vi>[])
                n573 = property on="Record #" class="DigNum (strict)"(error in=w945, "Maximum"=w950) -> (error out=w937:errorcluster)  [unwired: 1 in, 1 out]
                n574 = local read "srchParams"() -> (w936:T10)
                n575 = Bundle By Name(cluster=w936, "lkupPanelEndDate"=w935) -> (w934:T10)
                n576 = Select(t=T16."Enabled" ("Disabled"), s=w955, f=T16."Disabled and Grayed Out" ("Disabled")) -> (s? t:f=w954:T16)
                n577 = for {
                  tunnel: w949 -> [w960] mode=indexing
                  n578 = property on="Property Node" class="Ring (strict)"(reference=w960, "Strings []"=string[] []) -> ()  [unwired: 1 in, 2 out]
                }
                n579 = property on="addShot" class="Bool"("Disabled"=T16."Enabled") -> ()  [unwired: 2 in, 2 out]
                n580 = property on="undoLastShot" class="Bool"("Disabled"=w933) -> ()  [unwired: 2 in, 2 out]
                n581 = property on="saveShots" class="Bool"("Disabled"=w933) -> ()  [unwired: 2 in, 2 out]
                n582 = property on="clearShots" class="Bool"("Disabled"=w933) -> ()  [unwired: 2 in, 2 out]
                n583 = property on="prjV50Rpt" class="Bool"("DisabledEnum"=w933) -> ()  [unwired: 2 in, 2 out]
                n584 = local write "srchParams"(w934) -> ()
                n585 = property on="ARM" class="Bool"("Disabled"=w954) -> ()  [unwired: 2 in, 2 out]
                n586 = property on="saveReq" class="Str"("Visible"=TRUE) -> ()  [unwired: 2 in, 2 out]
              }
            }
            n587 = call <vilib>:"General Error Handler.vi"("error in (no error)"=w883) -> ("error out"=w855:errorcluster)  [unwired: 2 in, 12 out]
            n588 = flat-sequence {
              tunnel: w855 -> [w887]
              frame #0 {
                n589 = local read "ConfigName"() -> (w888:string)
                n590 = case shown="No Error" w887 {
                  tunnel: [w891 "NOT READY!" ("ConfigName")] -> w889
                  tunnel: w888 -> [w891 _]
                  frame No Error {
                    n591 = Wait (ms)(milliseconds to wait=u32 1000) -> ()  [unwired: 1 out]
                  }
                  frame Error {
                  }
                }
                "ConfigName" <- w889
              }
            }
            "saveReq" <- "Number of layers in sample ply specification and number of shots in shots table must be greater than 0 to enable saving." ("saveReq")
          }
        }
      }
      frame "V50 Report or GET Record" {
        # "case # 2"
        # "The custom Excel template file is \nexpected in the C:\\Ballistics folder."
        n592 = case shown="True" "lookupRec" {
          selector: "lookupRec" -> [_ w1579]
          tunnel: [w1016 w1569] -> w996
          tunnel: [w1015 w1555] -> w995
          tunnel: [w1014 w1572] -> w994
          tunnel: [w1013 w1512] -> w993
          tunnel: [w1012 w1570] -> w992
          tunnel: [w1011 w1532] -> w991
          tunnel: [w1010 w1519] -> w978
          tunnel: [w1009 w1521] -> w977
          tunnel: [w1008 w1522] -> w976
          tunnel: [w1007 "Record #"] -> w975
          tunnel: [w1006 w1571] -> w974
          tunnel: [w1005 w1521] -> w967
          tunnel: w972 -> [w1004 _]
          tunnel: [w1003 w1544] -> w970
          tunnel: w969 -> [w1003 w1545]
          tunnel: [w1002 w1517] -> w965
          frame False {
            n593 = local read "Site"() -> (w1001:string)
            n594 = stacked-sequence {
              tunnel: [_ _ _ _ _ w1412] -> w1011
              tunnel: [_ w1080 _ _ _ _] -> w1015
              tunnel: [_ _ _ _ w1204 _] -> w1012
              tunnel: [_ _ _ w1137 _ _] -> w1013
              tunnel: [_ _ w1103 _ _ _] -> w1014
              tunnel: [w1028 _ _ _ _ _] -> w1016
              tunnel: [_ _ _ _ _ w1418] -> w1010
              tunnel: [_ _ _ _ _ w1414] -> w1009
              tunnel: [_ _ _ _ _ w1413] -> w1008
              tunnel: [_ _ _ _ _ w1417] -> w1007
              tunnel: [_ _ _ _ _ w1416] -> w1006
              tunnel: [_ _ _ _ _ w1415] -> w1005
              tunnel: w1004 -> [_ _ w1102 _ w1203 _]
              tunnel: w1001 -> [_ _ w1091 w1136 w1202 w1411]
              frame #0 {
                # "Need to remove first element\nsince it's associated with the \nhistory page."
                # "FABRIC"
                n595 = global read "BIMS_Collector Globals.vi" "SampleStyles"() -> (w1019:refnum<vi>[])
                n596 = global read "BIMS_Collector Globals.vi" "Mfrs"() -> (w1024:refnum<vi>[])
                n597 = global read "BIMS_Collector Globals.vi" "LayerStitchTypeRefs"() -> (w1026:refnum<vi>[])
                n598 = local read "fab1_totalWt"() -> (w1031:sgl)
                n599 = local read "fab2_totalWt"() -> (w1032:sgl)
                n600 = local read "fab3_totalWt"() -> (w1033:sgl)
                n601 = local read "fab4_totalWt"() -> (w1034:sgl)
                n602 = local read "fab5_totalWt"() -> (w1035:sgl)
                n603 = local read "fab6_totalWt"() -> (w1036:sgl)
                n604 = global read "BIMS_Collector Globals.vi" "SampleAttribs"() -> (w1017:T29)
                n605 = global read "BIMS_Collector Globals.vi" "LayerSpecs"() -> (w1027:T23)
                n606 = Delete From Array(array=w1019, length=1, index=0) -> (array with subset deleted=w1018:refnum<vi>[])  [unwired: 1 out]
                n607 = Delete From Array "Delete From Array"(array=w1024, length=1, index=0) -> (array with subset deleted=w1025:refnum<vi>[])  [unwired: 1 out]
                n608 = Build Array(w1031, w1032, w1033, w1034, w1035, w1036) -> (w1030:sgl[])
                n609 = for {
                  tunnel: w1030 -> [w1040] mode=indexing
                  tunnel: [w1048] -> w1029 mode=indexing
                  tunnel: w1017 -> [w1047] mode=indexing
                  tunnel: w1027 -> [w1046] mode=indexing
                  tunnel: w1025 -> [w1045] mode=indexing
                  tunnel: w1018 -> [w1044] mode=indexing
                  tunnel: w1026 -> [w1043] mode=indexing
                  n610 = call "Dropdown Selection (SubVI).vi"("reference"=w1045) -> ("element"=w1038:string)
                  n611 = call "Dropdown Selection (SubVI).vi"("reference"=w1044) -> ("element"=w1042:string)
                  n612 = Equal?(x="", y=w1038) -> (x = y?=w1037:bool)
                  n613 = call "Dropdown Selection (SubVI).vi"("reference"=w1043) -> ("element"=w1041:string)
                  n614 = case shown="False" w1037 {
                    tunnel: [w1067 w1069] -> w1048
                    tunnel: w1047 -> [w1066 _]
                    tunnel: w1046 -> [w1065 _]
                    tunnel: w1042 -> [w1059 _]
                    tunnel: w1041 -> [w1054 _]
                    tunnel: w1040 -> [w1052 _]
                    tunnel: w1038 -> [w1051 _]
                    frame False {
                      n615 = Unbundle By Name(w1065) -> ("numOfPlies"=w1053:i32, "LotNum"=w1062:string, "RollNum"=w1063:string)
                      n616 = Unbundle By Name(w1066) -> ("internal_ID"=w1057:string, "fiber"=w1058:string, "denier"=w1061:string, "pick"=w1060:string, "weave"=w1055:string, "finish"=w1056:string, "ozPerYd2"=w1064:string)
                      n617 = Format Into String(w1053) -> (resulting string=w1050:string)  [unwired: 3 in, 1 out]
                      n618 = Format Into String(w1052) -> (resulting string=w1049:string)  [unwired: 3 in, 1 out]
                      n619 = Build Array(w1050, w1051, w1059, w1057, w1058, w1061, w1060, w1055, w1056, w1062, w1063, w1064, w1049, w1054) -> (w1067:string[])
                    }
                    frame True {
                      n620 = Initialize Array("", 14 ("dimension size")) -> (w1069:string[])
                    }
                  }
                }
                n621 = Transpose 2D Array(2D array=w1029) -> (transposed array=w1028:string[][])
              }
              frame #1 {
                w1072 = "%.1f" ("format string")
                # "RANGE"
                n622 = local read "Barrel to Screen"() -> (w1073:sgl)
                n623 = local read "Set#1 Separation"() -> (w1075:sgl)
                n624 = local read "mid_to_targ_dist"() -> (w1074:sgl)
                n625 = local read "clayAverage"() -> (w1088:sgl)
                n626 = local read "RoomHum"() -> (w1083:sgl)
                n627 = local read "clayTemp"() -> (w1086:sgl)
                n628 = local read "clayCalib"() -> (w1089:string)
                n629 = local read "RoomT"() -> (w1084:sgl)
                n630 = call "range distances (SubVI).vi"("mid_to_targ_dist"=w1074, "Set#1 Separation"=w1075, "Barrel to Screen"=w1073) -> ("scr#2 / target"=w1071:string, "Set#1 Separation"=w1078:string, "muzzle / scr#1"=w1077:string, "muzzle / target"=w1076:string, "mid_to_targ_dist"=w1079:string)  [unwired: 3 in]
                n631 = Format Into String(w1083) -> (resulting string=w1081:string)  [unwired: 3 in, 1 out]
                n632 = Format Into String(format string=w1072, w1084) -> (resulting string=w1082:string)  [unwired: 2 in, 1 out]
                n633 = Format Into String(format string=w1072, w1086) -> (resulting string=w1085:string)  [unwired: 2 in, 1 out]
                n634 = Format Into String(format string=w1072, w1088) -> (resulting string=w1087:string)  [unwired: 2 in, 1 out]
                n635 = Bundle("muzzle / target"=w1076, "muzzle / scr#1"=w1077, "Set#1 Separation"=w1078, "scr#2 / target"=w1071, "mid_to_targ_dist"=w1079, w1081, w1082, w1085, "clayCalib"=w1089, w1087) -> (w1090:T39)  [unwired: 1 out]
                n636 = Cluster To Array(cluster=w1090) -> (array=w1080:string[])
              }
              frame #2 {
                # "RESULTS"
                n637 = for {
                  tunnel: w1102 -> [w1135] mode=indexing
                  tunnel: [w1134] -> w1101 mode=indexing
                  tunnel: [w1133] -> w1100
                  i -> [w1133]
                  n638 = Unbundle By Name(w1135) -> ("BackFace\nDepth"=w1134:sgl)
                }
                n639 = Increment(x=w1100) -> (x+1=w1098:i32)
                n640 = Add Array Elements(numeric array=w1101) -> (sum=w1099:sgl)
                n641 = To Single Precision Float(number=w1098) -> (single precision float=w1097:sgl)
                n642 = control-ref of="Methods"() -> (w1092:refnum<vi>)
                n643 = Divide(x=w1099, y=w1097) -> (x/y=w1096:sgl)
                n644 = call "Dropdown Selection (SubVI).vi"("reference"=w1092) -> ("element"=w1093:string)
                n645 = Format Into String(format string="%1.1f", w1096) -> (resulting string=w1095:string)  [unwired: 2 in, 1 out]
                n646 = case shown="\"V50\"" w1093 {
                  tunnel: [w1121 w1132] -> w1105
                  tunnel: w1095 -> [w1111 w1131]
                  tunnel: w1091 -> [w1110 _]
                  frame "V50" {
                    w1115 = "%1d" ("format string")
                    n647 = local read "Z.M.R."() -> (w1107:sgl)
                    n648 = local read "rangeOfResults"() -> (w1117:i32)
                    n649 = local read "computed_V50"() -> (w1120:sgl)
                    n650 = local read "lowComplete"() -> (w1118:i32)
                    n651 = local read "highPartial"() -> (w1119:i32)
                    n652 = Less Than 0?(x=w1107) -> (x < 0?=w1108:bool)
                    n653 = Select(t=sgl 0.0 ("Z.M.R."), s=w1108, f=w1107) -> (s? t:f=w1106:sgl)
                    n654 = case shown="\"BRZ\"" w1110 {
                      tunnel: [w1126 w1128] -> w1112
                      tunnel: w1111 -> [w1126 _]
                      frame Default {
                      }
                      frame "BRZ" {
                        n655 = local read "velSTDEV"() -> (w1129:sgl)
                        n656 = Format Into String(format string="%1.1f", w1129) -> (resulting string=w1128:string)  [unwired: 2 in, 1 out]
                      }
                    }
                    n657 = Format Into String(format string="%1.1f", w1120) -> (resulting string=w1124:string)  [unwired: 2 in, 1 out]
                    n658 = Format Into String(format string=w1115, w1119) -> (resulting string=w1123:string)  [unwired: 2 in, 1 out]
                    n659 = Format Into String(format string=w1115, w1118) -> (resulting string=w1122:string)  [unwired: 2 in, 1 out]
                    n660 = Format Into String(format string=w1115, w1117) -> (resulting string=w1125:string)  [unwired: 2 in, 1 out]
                    n661 = Format Into String(format string="%1.1f", w1106) -> (resulting string=w1114:string)  [unwired: 2 in, 1 out]
                    n662 = Bundle(w1124, w1123, w1122, w1125, w1114, w1112, w1111) -> (w1121:T40)  [unwired: 1 out]
                  }
                  frame Default {
                    w1130 = "" ("Empty String Constant")
                    n663 = Bundle(w1130, w1130, w1130, w1130, w1130, w1131, w1131) -> (w1132:T40)  [unwired: 1 out]
                  }
                }
                n664 = Cluster To Array(cluster=w1105) -> (array=w1104:string[])
                n665 = Build Array(w1104) -> (w1103:string[][])
              }
              frame #3 {
                # "SAMPLE"
                n666 = case shown="\"ICE1\", Default" w1136 {
                  tunnel: [w1139 w1163 w1176 w1189] -> w1137
                  frame "ICE1", Default {
                    # "PB Req"
                    n667 = control-ref of="Methods"() -> (w1140:refnum<vi>)
                    n668 = call "Dropdown Selection (SubVI).vi"("reference"=w1140) -> ("element"=w1142:string)
                    n669 = Equal?(x=w1142, y="V50") -> (x = y?=w1141:bool)
                    n670 = local read "totalSampleWt"() -> (w1152:sgl)
                    n671 = case shown="True" w1141 {
                      tunnel: ["n/a" w1162] -> w1146
                      frame False {
                      }
                      frame True {
                        n672 = local read "minV50"() -> (w1161:i32)
                        n673 = Format Into String(w1161) -> (resulting string=w1162:string)  [unwired: 3 in, 1 out]
                      }
                    }
                    n674 = control-ref of="SampleDimensions"() -> (w1158:refnum<vi>)
                    n675 = control-ref of="SampleCoverings"() -> (w1159:refnum<vi>)
                    n676 = control-ref of="Models"() -> (w1145:refnum<vi>)
                    n677 = local read "serialNum"() -> (w1154:string)
                    n678 = local read "SampleID"() -> (w1156:string)
                    n679 = local read "Thickness"() -> (w1149:dbl)
                    n680 = local read "totalBAW"() -> (w1148:sgl)
                    n681 = call "Dropdown Selection (SubVI).vi"("reference"=w1158) -> ("element"=w1155:string)
                    n682 = call "Dropdown Selection (SubVI).vi"("reference"=w1145) -> ("element"=w1144:string)
                    n683 = call "Dropdown Selection (SubVI).vi"("reference"=w1159) -> ("element"=w1153:string)
                    n684 = Format Into String(w1152) -> (resulting string=w1151:string)  [unwired: 3 in, 1 out]
                    n685 = Format Into String(w1149) -> (resulting string=w1150:string)  [unwired: 3 in, 1 out]
                    n686 = Format Into String(w1148) -> (resulting string=w1147:string)  [unwired: 3 in, 1 out]
                    n687 = Bundle("SampleID"=w1156, "element"=w1155, "Type of work"="Type of work", "serialNum"=w1154, "element"=w1144, w1151, w1150, w1147, "element"=w1153, w1146) -> (w1157:T41)  [unwired: 1 out]
                    n688 = Cluster To Array(cluster=w1157) -> (array=w1139:string[])
                  }
                  frame "SPR0" {
                    n689 = local read "totalSampleWt"() -> (w1169:sgl)
                    n690 = control-ref of="SampleDimensions"() -> (w1174:refnum<vi>)
                    n691 = control-ref of="SampleCoverings"() -> (w1175:refnum<vi>)
                    n692 = local read "SampleID"() -> (w1172:string)
                    n693 = local read "Thickness"() -> (w1166:dbl)
                    n694 = local read "totalBAW"() -> (w1165:sgl)
                    n695 = call "Dropdown Selection (SubVI).vi"("reference"=w1174) -> ("element"=w1171:string)
                    n696 = call "Dropdown Selection (SubVI).vi"("reference"=w1175) -> ("element"=w1170:string)
                    n697 = Format Into String(w1169) -> (resulting string=w1168:string)  [unwired: 3 in, 1 out]
                    n698 = Format Into String(w1166) -> (resulting string=w1167:string)  [unwired: 3 in, 1 out]
                    n699 = Format Into String(w1165) -> (resulting string=w1164:string)  [unwired: 3 in, 1 out]
                    n700 = Bundle("SampleID"=w1172, "element"=w1171, w1168, w1167, w1164, "element"=w1170) -> (w1173:T42)  [unwired: 1 out]
                    n701 = Cluster To Array(cluster=w1173) -> (array=w1163:string[])
                  }
                  frame "SPR1" {
                    n702 = local read "totalSampleWt"() -> (w1182:sgl)
                    n703 = control-ref of="SampleDimensions"() -> (w1187:refnum<vi>)
                    n704 = control-ref of="SampleCoverings"() -> (w1188:refnum<vi>)
                    n705 = local read "Thickness"() -> (w1179:dbl)
                    n706 = local read "totalBAW"() -> (w1178:sgl)
                    n707 = local read "SampleID"() -> (w1185:string)
                    n708 = call "Dropdown Selection (SubVI).vi"("reference"=w1187) -> ("element"=w1184:string)
                    n709 = call "Dropdown Selection (SubVI).vi"("reference"=w1188) -> ("element"=w1183:string)
                    n710 = Format Into String(w1182) -> (resulting string=w1181:string)  [unwired: 3 in, 1 out]
                    n711 = Format Into String(w1179) -> (resulting string=w1180:string)  [unwired: 3 in, 1 out]
                    n712 = Format Into String(w1178) -> (resulting string=w1177:string)  [unwired: 3 in, 1 out]
                    n713 = Bundle("SampleID"=w1185, "element"=w1184, w1181, w1180, w1177, "element"=w1183) -> (w1186:T42)  [unwired: 1 out]
                    n714 = Cluster To Array(cluster=w1186) -> (array=w1176:string[])
                  }
                  frame "BRZ" {
                    n715 = local read "totalSampleWt"() -> (w1195:sgl)
                    n716 = control-ref of="SampleDimensions"() -> (w1200:refnum<vi>)
                    n717 = control-ref of="SampleCoverings"() -> (w1201:refnum<vi>)
                    n718 = local read "SampleID"() -> (w1198:string)
                    n719 = local read "Thickness"() -> (w1192:dbl)
                    n720 = local read "totalBAW"() -> (w1191:sgl)
                    n721 = call "Dropdown Selection (SubVI).vi"("reference"=w1200) -> ("element"=w1197:string)
                    n722 = call "Dropdown Selection (SubVI).vi"("reference"=w1201) -> ("element"=w1196:string)
                    n723 = Format Into String(w1195) -> (resulting string=w1194:string)  [unwired: 3 in, 1 out]
                    n724 = Format Into String(w1192) -> (resulting string=w1193:string)  [unwired: 3 in, 1 out]
                    n725 = Format Into String(w1191) -> (resulting string=w1190:string)  [unwired: 3 in, 1 out]
                    n726 = Bundle("SampleID"=w1198, "element"=w1197, w1194, w1193, w1190, "element"=w1196) -> (w1199:T42)  [unwired: 1 out]
                    n727 = Cluster To Array(cluster=w1199) -> (array=w1189:string[])
                  }
                }
              }
              frame #4 {
                n728 = case shown="\"BRZ\"" w1202 {
                  tunnel: [w1214 w1264 w1316 w1368] -> w1204
                  tunnel: w1203 -> [w1207 w1257 w1309 w1361]
                  frame "ICE1", Default {
                    # "SHOT TABLE"
                    n729 = control-ref of="Methods"() -> (w1206:refnum<vi>)
                    n730 = call "Dropdown Selection (SubVI).vi"("reference"=w1206) -> ("element"=w1205:string)
                    n731 = for {
                      tunnel: w1207 -> [w1246] mode=indexing
                      shift-right: [w1223] -> _
                      shift-left: T33 [] -> [w1225]
                      tunnel: [w1223] -> w1210
                      tunnel: w1205 -> [w1219]
                      n732 = Unbundle By Name(w1246) -> ("shot order"=w1245:i32, "Powder Loading"=w1244:sgl, "Uncorrected Impact"=w1243:sgl, "UncorrectedRed_PB"=w1242:sgl, "UncorrectedAvgVel_PB"=w1241:sgl, "velLoss_PB"=w1240:sgl, "strikeVel_PB"=w1239:sgl, "SHOT STATUS"=w1228:u16, "usedv50"=w1238:bool, "Shot Angle"=w1220:u16, "BackFace\nDepth"=w1221:sgl)
                      n733 = case shown="\"V50\"" w1219 {
                        tunnel: w1238 -> [w1248 _]
                        tunnel: [w1247 w1252] -> w1237
                        tunnel: w1220 -> [_ w1251]
                        frame "V50" {
                          n734 = case shown="True" w1248 {
                            tunnel: ["" ("Empty String Constant") "*"] -> w1247
                            frame False {
                            }
                            frame True {
                            }
                          }
                        }
                        frame Default {
                          n735 = Format Into String(w1251) -> (resulting string=w1252:string)  [unwired: 3 in, 1 out]
                        }
                      }
                      n736 = case shown="1" w1228 {
                        tunnel: ["P" "C"] -> w1227
                        frame 0, Default {
                        }
                        frame 1 {
                        }
                      }
                      n737 = Format Into String(format string="%2d", w1245) -> (resulting string=w1230:string)  [unwired: 2 in, 1 out]
                      n738 = Format Into String(w1244) -> (resulting string=w1231:string)  [unwired: 3 in, 1 out]
                      n739 = Format Into String(w1243) -> (resulting string=w1232:string)  [unwired: 3 in, 1 out]
                      n740 = Format Into String(w1242) -> (resulting string=w1233:string)  [unwired: 3 in, 1 out]
                      n741 = Format Into String(w1241) -> (resulting string=w1234:string)  [unwired: 3 in, 1 out]
                      n742 = Format Into String(w1240) -> (resulting string=w1235:string)  [unwired: 3 in, 1 out]
                      n743 = Format Into String(w1239) -> (resulting string=w1236:string)  [unwired: 3 in, 1 out]
                      n744 = Format Into String(w1221) -> (resulting string=w1229:string)  [unwired: 3 in, 1 out]
                      n745 = Build Array(w1230, w1231, w1232, w1233, w1234, w1235, w1236, w1227, w1237, w1229) -> (w1224:string[])
                      n746 = Array To Cluster(array=w1224) -> (cluster=w1226:T43)
                      n747 = Build Array (concatenate)(w1225, w1226) -> (w1223:T33)
                    }
                    n748 = Array Size(array=w1210) -> (size(s)=w1212:i32)
                    n749 = Equal To 0?(x=w1212) -> (x = 0?=w1208:bool)
                    n750 = case shown="True" w1208 {
                      tunnel: [w1215 T33 [{"[0]"="", "[1]"="", "[2]"="", "[3]"="", "[4]"="", "[5]"="", "[6]"="", "[7]"="", "[8]"="", "[9]"=""}]] -> w1209
                      tunnel: w1210 -> [w1215 _]
                      frame False {
                      }
                      frame True {
                      }
                    }
                    n751 = Sort 1D Array(array=w1209) -> (sorted array=w1211:T33)
                    n752 = for {
                      tunnel: w1211 -> [w1218] mode=indexing
                      tunnel: [w1217] -> w1214 mode=indexing
                      n753 = Cluster To Array(cluster=w1218) -> (array=w1217:string[])
                    }
                  }
                  frame "SPR0" {
                    # "SHOT TABLE"
                    n754 = control-ref of="Methods"() -> (w1256:refnum<vi>)
                    n755 = call "Dropdown Selection (SubVI).vi"("reference"=w1256) -> ("element"=w1255:string)
                    n756 = for {
                      tunnel: w1257 -> [w1294] mode=indexing
                      shift-right: [w1275] -> _
                      shift-left: T34 [] -> [w1277]
                      tunnel: [w1275] -> w1260
                      tunnel: w1255 -> [w1271]
                      n757 = Unbundle By Name(w1294) -> ("shot order"=w1293:i32, "Powder Loading"=w1292:sgl, "Uncorrected Impact"=w1291:sgl, "UncorrectedRed_PB"=w1290:sgl, "strikeVel_PB"=w1289:sgl, "SHOT STATUS"=w1280:u16, "usedv50"=w1288:bool, "Shot Angle"=w1272:u16, "BackFace\nDepth"=w1273:sgl, "V50userExcl"=w1270:bool, "Shot Description"=w1269:string)
                      n758 = case shown="\"V50\"" w1271 {
                        tunnel: w1288 -> [w1297 _]
                        tunnel: [w1296 w1304] -> w1287
                        tunnel: w1272 -> [_ w1303]
                        tunnel: w1270 -> [w1295 _]
                        frame "V50" {
                          n759 = case shown="True" w1295 {
                            tunnel: w1297 -> [w1299 _]
                            tunnel: [w1298 "!"] -> w1296
                            frame False {
                              n760 = case shown="False" w1299 {
                                tunnel: ["" ("Empty String Constant") "*"] -> w1298
                                frame False {
                                }
                                frame True {
                                }
                              }
                            }
                            frame True {
                            }
                          }
                        }
                        frame Default {
                          n761 = Format Into String(w1303) -> (resulting string=w1304:string)  [unwired: 3 in, 1 out]
                        }
                      }
                      n762 = case shown="1" w1280 {
                        tunnel: ["P" "C"] -> w1279
                        frame 0, Default {
                        }
                        frame 1 {
                        }
                      }
                      n763 = Format Into String(format string="%2d", w1293) -> (resulting string=w1282:string)  [unwired: 2 in, 1 out]
                      n764 = Format Into String(w1292) -> (resulting string=w1283:string)  [unwired: 3 in, 1 out]
                      n765 = Format Into String(w1291) -> (resulting string=w1284:string)  [unwired: 3 in, 1 out]
                      n766 = Format Into String(w1290) -> (resulting string=w1285:string)  [unwired: 3 in, 1 out]
                      n767 = Format Into String(w1289) -> (resulting string=w1286:string)  [unwired: 3 in, 1 out]
                      n768 = Format Into String(w1273) -> (resulting string=w1281:string)  [unwired: 3 in, 1 out]
                      n769 = Build Array(w1282, w1283, w1284, w1285, w1286, w1279, w1287, w1281, w1269) -> (w1276:string[])
                      n770 = Array To Cluster(array=w1276) -> (cluster=w1278:T44)
                      n771 = Build Array (concatenate)(w1277, w1278) -> (w1275:T34)
                    }
                    n772 = Array Size(array=w1260) -> (size(s)=w1262:i32)
                    n773 = Equal To 0?(x=w1262) -> (x = 0?=w1258:bool)
                    n774 = case shown="True" w1258 {
                      tunnel: [w1265 T34 [{"[0]"="", "[1]"="", "[2]"="", "[3]"="", "[4]"="", "[5]"="", "[6]"="", "[7]"="", "[8]"=""}]] -> w1259
                      tunnel: w1260 -> [w1265 _]
                      frame False {
                      }
                      frame True {
                      }
                    }
                    n775 = Sort 1D Array(array=w1259) -> (sorted array=w1261:T34)
                    n776 = for {
                      tunnel: w1261 -> [w1268] mode=indexing
                      tunnel: [w1267] -> w1264 mode=indexing
                      n777 = Cluster To Array(cluster=w1268) -> (array=w1267:string[])
                    }
                  }
                  frame "SPR1" {
                    # "SHOT TABLE"
                    n778 = control-ref of="Methods"() -> (w1308:refnum<vi>)
                    n779 = call "Dropdown Selection (SubVI).vi"("reference"=w1308) -> ("element"=w1307:string)
                    n780 = for {
                      tunnel: w1309 -> [w1346] mode=indexing
                      shift-right: [w1327] -> _
                      shift-left: T34 [] -> [w1329]
                      tunnel: [w1327] -> w1312
                      tunnel: w1307 -> [w1323]
                      n781 = Unbundle By Name(w1346) -> ("shot order"=w1345:i32, "Powder Loading"=w1344:sgl, "Uncorrected Impact"=w1343:sgl, "UncorrectedRed_PB"=w1342:sgl, "strikeVel_PB"=w1341:sgl, "SHOT STATUS"=w1332:u16, "usedv50"=w1340:bool, "Shot Angle"=w1324:u16, "BackFace\nDepth"=w1325:sgl, "V50userExcl"=w1322:bool, "Shot Description"=w1321:string)
                      n782 = case shown="\"V50\"" w1323 {
                        tunnel: w1340 -> [w1349 _]
                        tunnel: [w1348 w1356] -> w1339
                        tunnel: w1324 -> [_ w1355]
                        tunnel: w1322 -> [w1347 _]
                        frame "V50" {
                          n783 = case shown="True" w1347 {
                            tunnel: w1349 -> [w1351 _]
                            tunnel: [w1350 "!"] -> w1348
                            frame False {
                              n784 = case shown="False" w1351 {
                                tunnel: ["" ("Empty String Constant") "*"] -> w1350
                                frame False {
                                }
                                frame True {
                                }
                              }
                            }
                            frame True {
                            }
                          }
                        }
                        frame Default {
                          n785 = Format Into String(w1355) -> (resulting string=w1356:string)  [unwired: 3 in, 1 out]
                        }
                      }
                      n786 = case shown="1" w1332 {
                        tunnel: ["P" "C"] -> w1331
                        frame 0, Default {
                        }
                        frame 1 {
                        }
                      }
                      n787 = Format Into String(format string="%2d", w1345) -> (resulting string=w1334:string)  [unwired: 2 in, 1 out]
                      n788 = Format Into String(w1344) -> (resulting string=w1335:string)  [unwired: 3 in, 1 out]
                      n789 = Format Into String(w1343) -> (resulting string=w1336:string)  [unwired: 3 in, 1 out]
                      n790 = Format Into String(w1342) -> (resulting string=w1337:string)  [unwired: 3 in, 1 out]
                      n791 = Format Into String(w1341) -> (resulting string=w1338:string)  [unwired: 3 in, 1 out]
                      n792 = Format Into String(w1325) -> (resulting string=w1333:string)  [unwired: 3 in, 1 out]
                      n793 = Build Array(w1334, w1335, w1336, w1337, w1338, w1331, w1339, w1333, w1321) -> (w1328:string[])
                      n794 = Array To Cluster(array=w1328) -> (cluster=w1330:T44)
                      n795 = Build Array (concatenate)(w1329, w1330) -> (w1327:T34)
                    }
                    n796 = Array Size(array=w1312) -> (size(s)=w1314:i32)
                    n797 = Equal To 0?(x=w1314) -> (x = 0?=w1310:bool)
                    n798 = case shown="True" w1310 {
                      tunnel: [w1317 T34 [{"[0]"="", "[1]"="", "[2]"="", "[3]"="", "[4]"="", "[5]"="", "[6]"="", "[7]"="", "[8]"=""}]] -> w1311
                      tunnel: w1312 -> [w1317 _]
                      frame False {
                      }
                      frame True {
                      }
                    }
                    n799 = Sort 1D Array(array=w1311) -> (sorted array=w1313:T34)
                    n800 = for {
                      tunnel: w1313 -> [w1320] mode=indexing
                      tunnel: [w1319] -> w1316 mode=indexing
                      n801 = Cluster To Array(cluster=w1320) -> (array=w1319:string[])
                    }
                  }
                  frame "BRZ" {
                    # "SHOT TABLE"
                    n802 = control-ref of="Methods"() -> (w1360:refnum<vi>)
                    n803 = call "Dropdown Selection (SubVI).vi"("reference"=w1360) -> ("element"=w1359:string)
                    n804 = for {
                      tunnel: w1361 -> [w1398] mode=indexing
                      shift-right: [w1379] -> _
                      shift-left: T34 [] -> [w1381]
                      tunnel: [w1379] -> w1364
                      tunnel: w1359 -> [w1375]
                      n805 = Unbundle By Name(w1398) -> ("shot order"=w1397:i32, "Powder Loading"=w1396:sgl, "Uncorrected Impact"=w1395:sgl, "UncorrectedRed_PB"=w1394:sgl, "strikeVel_PB"=w1393:sgl, "SHOT STATUS"=w1384:u16, "usedv50"=w1392:bool, "Shot Angle"=w1376:u16, "BackFace\nDepth"=w1377:sgl, "V50userExcl"=w1374:bool, "Shot Description"=w1373:string)
                      n806 = case shown="\"V50\"" w1375 {
                        tunnel: w1392 -> [w1401 _]
                        tunnel: [w1400 w1408] -> w1391
                        tunnel: w1376 -> [_ w1407]
                        tunnel: w1374 -> [w1399 _]
                        frame "V50" {
                          n807 = case shown="True" w1399 {
                            tunnel: w1401 -> [w1403 _]
                            tunnel: [w1402 "!"] -> w1400
                            frame False {
                              n808 = case shown="False" w1403 {
                                tunnel: ["" ("Empty String Constant") "*"] -> w1402
                                frame False {
                                }
                                frame True {
                                }
                              }
                            }
                            frame True {
                            }
                          }
                        }
                        frame Default {
                          n809 = Format Into String(w1407) -> (resulting string=w1408:string)  [unwired: 3 in, 1 out]
                        }
                      }
                      n810 = case shown="1" w1384 {
                        tunnel: ["P" "C"] -> w1383
                        frame 0, Default {
                        }
                        frame 1 {
                        }
                      }
                      n811 = Format Into String(format string="%2d", w1397) -> (resulting string=w1386:string)  [unwired: 2 in, 1 out]
                      n812 = Format Into String(w1396) -> (resulting string=w1387:string)  [unwired: 3 in, 1 out]
                      n813 = Format Into String(w1395) -> (resulting string=w1388:string)  [unwired: 3 in, 1 out]
                      n814 = Format Into String(w1394) -> (resulting string=w1389:string)  [unwired: 3 in, 1 out]
                      n815 = Format Into String(w1393) -> (resulting string=w1390:string)  [unwired: 3 in, 1 out]
                      n816 = Format Into String(w1377) -> (resulting string=w1385:string)  [unwired: 3 in, 1 out]
                      n817 = Build Array(w1386, w1387, w1388, w1389, w1390, w1383, w1391, w1385, w1373) -> (w1380:string[])
                      n818 = Array To Cluster(array=w1380) -> (cluster=w1382:T44)
                      n819 = Build Array (concatenate)(w1381, w1382) -> (w1379:T34)
                    }
                    n820 = Array Size(array=w1364) -> (size(s)=w1366:i32)
                    n821 = Equal To 0?(x=w1366) -> (x = 0?=w1362:bool)
                    n822 = case shown="True" w1362 {
                      tunnel: [w1369 T34 [{"[0]"="", "[1]"="", "[2]"="", "[3]"="", "[4]"="", "[5]"="", "[6]"="", "[7]"="", "[8]"=""}]] -> w1363
                      tunnel: w1364 -> [w1369 _]
                      frame False {
                      }
                      frame True {
                      }
                    }
                    n823 = Sort 1D Array(array=w1363) -> (sorted array=w1365:T34)
                    n824 = for {
                      tunnel: w1365 -> [w1372] mode=indexing
                      tunnel: [w1371] -> w1368 mode=indexing
                      n825 = Cluster To Array(cluster=w1372) -> (array=w1371:string[])
                    }
                  }
                }
              }
              frame #5 {
                n826 = case shown="\"BRZ\"" w1411 {
                  tunnel: [w1442 w1463 w1483 w1503] -> w1418
                  tunnel: [w1441 w1462 w1482 w1502] -> w1417
                  tunnel: [w1440 w1461 w1481 w1501] -> w1416
                  tunnel: [w1439 w1446 w1466 w1486] -> w1415
                  tunnel: ["" ("projNum") w1446 w1466 w1486] -> w1414
                  tunnel: [w1437 w1460 w1480 w1500] -> w1413
                  tunnel: [w1421 w1449 w1469 w1489] -> w1412
                  frame "ICE1", Default {
                    # "THREAT"
                    # "Range # (supports a PB reporting requirement)"
                    # "Project Name goes here.\nSupports a PB reporting requirement."
                    # "GENERAL"
                    n827 = local read "threatDetails"() -> (w1420:T1)
                    n828 = Unbundle By Name(w1420) -> ("barrelLength"=w1424:string)
                    n829 = Unbundle By Name(w1420) -> ("grainSize"=w1419:string)
                    n830 = local read "Shot Angle"() -> (w1425:u16)
                    n831 = control-ref of="WeaponTypes"() -> (w1434:refnum<vi>)
                    n832 = control-ref of="ThreatGroups"() -> (w1433:refnum<vi>)
                    n833 = control-ref of="PowderTypes"() -> (w1432:refnum<vi>)
                    n834 = control-ref of="Recorders"() -> (w1435:refnum<vi>)
                    n835 = control-ref of="Shooters"() -> (w1436:refnum<vi>)
                    n836 = Format Into String(w1425) -> (resulting string=w1426:string)  [unwired: 3 in, 1 out]
                    n837 = call "Dropdown Selection (SubVI).vi"("reference"=w1434) -> ("element"=w1430:string)
                    n838 = call "Dropdown Selection (SubVI).vi"("reference"=w1433) -> ("element"=w1429:string)
                    n839 = call "Dropdown Selection (SubVI).vi"("reference"=w1432) -> ("element"=w1428:string)
                    n840 = call "Dropdown Selection (SubVI).vi"("reference"=w1435) -> ("element"=w1427:string)
                    n841 = call "Dropdown Selection (SubVI).vi"("reference"=w1436) -> ("element"=w1423:string)
                    n842 = local read "Comments"() -> (w1440:string)
                    n843 = local read "ProjectID"() -> (w1437:string)
                    n844 = Bundle("element"=w1430, "element"=w1429, "grainSize"=w1419, "element"=w1428, "barrelLength"=w1424, w1426, "element"="1", "element"=w1423, "element"=w1427) -> (w1431:T45)  [unwired: 1 out]
                    n845 = local read "lastSamp"() -> (w1445:i32)
                    n846 = control-ref of="TestStandards"() -> (w1444:refnum<vi>)
                    n847 = control-ref of="Methods"() -> (w1443:refnum<vi>)
                    n848 = Cluster To Array(cluster=w1431) -> (array=w1421:string[])
                    n849 = call "Dropdown Selection (SubVI).vi"("reference"=w1444) -> ("element"=w1439:string)
                    n850 = call "Dropdown Selection (SubVI).vi"("reference"=w1443) -> ("element"=w1442:string)
                    n851 = Increment(x=w1445) -> (x+1=w1441:i32)
                  }
                  frame "SPR0" {
                    w1446 = "" ("projNum")
                    # "THREAT"
                    # "Project Name goes here.\nSupports a PB reporting requirement."
                    # "GENERAL"
                    n852 = local read "threatDetails"() -> (w1448:T1)
                    n853 = Unbundle By Name(w1448) -> ("barrelLength"=w1451:string)
                    n854 = Unbundle By Name(w1448) -> ("grainSize"=w1447:string)
                    n855 = local read "Shot Angle"() -> (w1452:u16)
                    n856 = control-ref of="ThreatGroups"() -> (w1458:refnum<vi>)
                    n857 = control-ref of="PowderTypes"() -> (w1457:refnum<vi>)
                    n858 = control-ref of="Ballisticians"() -> (w1459:refnum<vi>)
                    n859 = Format Into String(w1452) -> (resulting string=w1453:string)  [unwired: 3 in, 1 out]
                    n860 = call "Dropdown Selection (SubVI).vi"("reference"=w1458) -> ("element"=w1455:string)
                    n861 = call "Dropdown Selection (SubVI).vi"("reference"=w1457) -> ("element"=w1454:string)
                    n862 = call "Dropdown Selection (SubVI).vi"("reference"=w1459) -> ("element"=w1450:string)
                    n863 = local read "Comments"() -> (w1461:string)
                    n864 = local read "ProjectID"() -> (w1460:string)
                    n865 = Bundle("element"=w1455, "grainSize"=w1447, "element"=w1454, "barrelLength"=w1451, w1453, "element"=w1450) -> (w1456:T46)  [unwired: 1 out]
                    n866 = local read "lastSamp"() -> (w1465:i32)
                    n867 = control-ref of="Methods"() -> (w1464:refnum<vi>)
                    n868 = Cluster To Array(cluster=w1456) -> (array=w1449:string[])
                    n869 = call "Dropdown Selection (SubVI).vi"("reference"=w1464) -> ("element"=w1463:string)
                    n870 = Increment(x=w1465) -> (x+1=w1462:i32)
                  }
                  frame "SPR1" {
                    w1466 = "" ("projNum")
                    # "THREAT"
                    # "Project Name goes here.\nSupports a PB reporting requirement."
                    # "GENERAL"
                    n871 = local read "threatDetails"() -> (w1468:T1)
                    n872 = Unbundle By Name(w1468) -> ("barrelLength"=w1471:string)
                    n873 = Unbundle By Name(w1468) -> ("grainSize"=w1467:string)
                    n874 = local read "Shot Angle"() -> (w1472:u16)
                    n875 = control-ref of="Ballisticians"() -> (w1479:refnum<vi>)
                    n876 = control-ref of="ThreatGroups"() -> (w1478:refnum<vi>)
                    n877 = control-ref of="PowderTypes"() -> (w1477:refnum<vi>)
                    n878 = call "Dropdown Selection (SubVI).vi"("reference"=w1479) -> ("element"=w1470:string)
                    n879 = call "Dropdown Selection (SubVI).vi"("reference"=w1478) -> ("element"=w1475:string)
                    n880 = call "Dropdown Selection (SubVI).vi"("reference"=w1477) -> ("element"=w1474:string)
                    n881 = Format Into String(w1472) -> (resulting string=w1473:string)  [unwired: 3 in, 1 out]
                    n882 = control-ref of="Methods"() -> (w1484:refnum<vi>)
                    n883 = local read "Comments"() -> (w1481:string)
                    n884 = local read "lastSamp"() -> (w1485:i32)
                    n885 = local read "ProjectID"() -> (w1480:string)
                    n886 = Bundle("element"=w1475, "grainSize"=w1467, "element"=w1474, "barrelLength"=w1471, w1473, "element"=w1470) -> (w1476:T46)  [unwired: 1 out]
                    n887 = call "Dropdown Selection (SubVI).vi"("reference"=w1484) -> ("element"=w1483:string)
                    n888 = Cluster To Array(cluster=w1476) -> (array=w1469:string[])
                    n889 = Increment(x=w1485) -> (x+1=w1482:i32)
                  }
                  frame "BRZ" {
                    w1486 = "" ("projNum")
                    # "THREAT"
                    # "Project Name goes here.\nSupports a PB reporting requirement."
                    # "GENERAL"
                    n890 = local read "threatDetails"() -> (w1488:T1)
                    n891 = Unbundle By Name(w1488) -> ("barrelLength"=w1491:string)
                    n892 = Unbundle By Name(w1488) -> ("grainSize"=w1487:string)
                    n893 = local read "Shot Angle"() -> (w1492:u16)
                    n894 = control-ref of="Ballisticians"() -> (w1499:refnum<vi>)
                    n895 = control-ref of="ThreatGroups"() -> (w1498:refnum<vi>)
                    n896 = control-ref of="PowderTypes"() -> (w1497:refnum<vi>)
                    n897 = call "Dropdown Selection (SubVI).vi"("reference"=w1499) -> ("element"=w1490:string)
                    n898 = call "Dropdown Selection (SubVI).vi"("reference"=w1498) -> ("element"=w1495:string)
                    n899 = call "Dropdown Selection (SubVI).vi"("reference"=w1497) -> ("element"=w1494:string)
                    n900 = Format Into String(w1492) -> (resulting string=w1493:string)  [unwired: 3 in, 1 out]
                    n901 = control-ref of="Methods"() -> (w1504:refnum<vi>)
                    n902 = local read "Comments"() -> (w1501:string)
                    n903 = local read "lastSamp"() -> (w1505:i32)
                    n904 = local read "ProjectID"() -> (w1500:string)
                    n905 = Bundle("element"=w1495, "grainSize"=w1487, "element"=w1494, "barrelLength"=w1491, w1493, "element"=w1490) -> (w1496:T46)  [unwired: 1 out]
                    n906 = call "Dropdown Selection (SubVI).vi"("reference"=w1504) -> ("element"=w1503:string)
                    n907 = Cluster To Array(cluster=w1496) -> (array=w1489:string[])
                    n908 = Increment(x=w1505) -> (x+1=w1502:i32)
                  }
                }
              }
            }
            n909 = Get Date/Time String() -> (date string=w1002:string)  [unwired: 3 in, 1 out]
          }
          frame True {
            w1521 = ""
            w1513 = 16  # dimensions
            w1516 = 5  # SampleID
            # "date"
            # "method"
            # "general"
            # "remark"
            # "threat"
            # "shots"
            # "sample"
            # "results"
            # "range"
            # "fabric"
            # "query db with the entered record number and use result to populate the xlt"
            n910 = Not(x=w1579) -> (.not. x?=w1578:bool)
            n911 = local write "lookupRec"(w1578) -> ()
            n912 = Format Into String(format string="SELECT * FROM Experiments\nWHERE expt=%d;" ("query string"), error in=w1545, "Record #") -> (resulting string=w1575:string, error out=w1546:errorcluster)  [unwired: 1 in]
            n913 = call "Fetch Data (SubVI).vi"("error IN"=w1546, "query string"=w1575) -> ("error OUT"=w1544:errorcluster, "recordset data"=w1577:string[][])  [unwired: 4 out]
            n914 = Index Array(array=w1577) -> (element=w1515:string[])  [unwired: 2 in]
            n915 = Index Array(array=w1515, index=111) -> (element=w1548:string)
            n916 = local read "Set#1 Separation"() -> (w1562:sgl)
            n917 = call "Load Shots (SubVI).vi"("Record #"="Record #", "Method"=w1548) -> ("Shot Array"=w1570:string[][], "AvgDef"=w1553:dbl)  [unwired: 1 in]
            n918 = local read "mid_to_targ_dist"() -> (w1565:sgl)
            n919 = local read "Barrel to Screen"() -> (w1568:sgl)
            n920 = Format Into String(w1553) -> (resulting string=w1551:string)  [unwired: 3 in, 1 out]
            n921 = Match Pattern(string=w1548, regular expression="N.I.J.") -> (offset past match=w1550:i32)  [unwired: 4 out]
            n922 = Greater Or Equal To 0?(x=w1550) -> (x >= 0?=w1547:bool)
            n923 = case shown="False" w1547 {
              tunnel: [w1590 w1591] -> w1552
              tunnel: w1551 -> [w1587 w1593]
              tunnel: w1515 -> [w1589 _]
              frame False {
                n924 = Index Array(array=w1589, index #1=124 ("index"), index #2=149 ("index"), index #5=145 ("index")) -> (element #1=w1588:string, element #2=w1586:string, element #3=w1585:string, element #4=w1581:string, element #5=w1582:string)  [unwired: 2 in]
                n925 = Build Array(w1588, w1586, w1585, w1581, w1582, w1587) -> (w1590:string[])
              }
              frame True {
                w1592 = "" ("Empty String Constant")
                n926 = Build Array(w1592, w1592, w1592, w1592, w1592, w1593, w1593) -> (w1591:string[])
              }
            }
            n927 = Divide(x=w1562, y=sgl 2.0) -> (x/y=w1567:sgl)
            n928 = Add(x=w1568, y=w1565) -> (x+y=w1561:sgl)
            n929 = Subtract(x=w1568, y=w1567) -> (x-y=w1566:sgl)
            n930 = Subtract(x=w1565, y=w1567) -> (x-y=w1564:sgl)
            n931 = Index Array(array=w1515, index #1=120 ("index"), index #2=119 ("index"), index #3=127 ("index"), index #4=12 ("index"), index #5=7 ("index")) -> (element #1=w1533:string, element #2=w1531:string, element #3=w1530:string, element #4=w1527:string, element #5=w1526:string)
            n932 = Index Array(array=w1515, index #1=113 ("index"), index #2=112 ("index"), index #3=103 ("index")) -> (element #1=w1542:string, element #2=w1541:string, element #3=w1540:string, element #4=w1539:string, element #5=w1535:string)  [unwired: 2 in]
            n933 = Format Into String(w1561) -> (resulting string=w1560:string)  [unwired: 3 in, 1 out]
            n934 = Format Into String(w1566) -> (resulting string=w1559:string)  [unwired: 3 in, 1 out]
            n935 = Format Into String(w1562) -> (resulting string=w1558:string)  [unwired: 3 in, 1 out]
            n936 = Format Into String(w1564) -> (resulting string=w1557:string)  [unwired: 3 in, 1 out]
            n937 = Format Into String(w1565) -> (resulting string=w1556:string)  [unwired: 3 in, 1 out]
            n938 = Index Array(array=w1515, index #1=w1516, index #2=w1513, index #3=147 ("index"), index #5=148 ("index")) -> (element #1=w1514:string, element #2=w1511:string, element #3=w1510:string, element #5=w1507:string)  [unwired: 1 in, 1 out]
            n939 = Build Array(w1533, w1531, w1530, "", w1527, w1526) -> (w1532:string[])
            n940 = Build Array(w1560, w1559, w1558, w1557, w1556, w1542, w1541, w1540, w1539, w1535) -> (w1555:string[])
            n941 = Index Array(array=w1515, index #1=4 ("index"), index #2=111 ("index")) -> (element #1=w1522:string, element #2=w1519:string)
            n942 = Index Array(array=w1515, index=107) -> (element=w1571:string)
            n943 = Build Array(w1514, w1511, w1510, "", w1507) -> (w1512:string[])
            n944 = Index Array(array=w1515, index=2) -> (element=w1517:string)
            n945 = call "Get Model Construction.vi"("panel record"=w1515) -> ("Fabric Array"=w1569:string[][])
            n946 = Build Array(w1552) -> (w1572:string[][])
          }
        }
        n947 = To Variant(anything=w996) -> (Variant=w990:variant)
        n948 = To Variant(anything=w995) -> (Variant=w989:variant)
        n949 = To Variant(anything=w994) -> (Variant=w988:variant)
        n950 = To Variant(anything=w993) -> (Variant=w987:variant)
        n951 = To Variant(anything=w992) -> (Variant=w986:variant)
        n952 = To Variant(anything=w991) -> (Variant=w985:variant)
        n953 = To Variant(anything=w978) -> (Variant=w984:variant)
        n954 = To Variant(anything=w977) -> (Variant=w983:variant)
        n955 = To Variant(anything=w976) -> (Variant=w982:variant)
        n956 = To Variant(anything=w975) -> (Variant=w979:variant)
        n957 = To Variant(anything=w974) -> (Variant=w980:variant)
        n958 = To Variant(anything=w967) -> (Variant=w981:variant)
        n959 = To Variant(anything=w965) -> (Variant=w966:variant)
        n960 = call "TestReport_XL.vi"("Enable"=TRUE, "blockFabric"=w990, "blockRange"=w989, "blockResults"=w988, "blockSample"=w987, "blockShotTbl"=w986, "error in (no error)"=w970, "blockThreat"=w985, "testDate"=w966, "method"=w984, "projName"=w983, "projNum"=w982, "recNum"=w979, "remark"=w980, "standard"=w981) -> ("error out"=w997:errorcluster)  [unwired: 4 in, 8 out]
        n961 = call <vilib>:"Simple Error Handler.vi"("error in (no error)"=w997) -> ("error out"=w999:errorcluster)  [unwired: 1 in, 7 out]
        n962 = case shown="No Error" w999 {
          selector: w999 -> [w1594 w1596]
          tunnel: [w1594 w1596] -> w968
          frame No Error {
            n963 = One Button Dialog(message=" V50 Ballistic Test Report is ready") -> ()  [unwired: 2 out]
          }
          frame Error {
          }
        }
      }
      frame "VsVr Report" {
        w1626 = TRUE  # Enable
        # "case # 3"
        # "The custom Excel template file is \nexpected in the C:\\Ballistics folder."
        n964 = stacked-sequence {
          tunnel: [_ _ _ _ _ w1817] -> w1619
          tunnel: [_ w1690 _ _ _ _] -> w1623
          tunnel: [_ _ _ _ w1774 _] -> w1620
          tunnel: [_ _ _ w1741 _ _] -> w1621
          tunnel: [_ _ w1712 _ _ _] -> w1622
          tunnel: [w1634 _ _ _ _ _] -> w1624
          tunnel: [_ _ _ _ _ w1838] -> w1606
          tunnel: [_ _ _ _ _ "" ("projNum")] -> w1605
          tunnel: [_ _ _ _ _ w1833] -> w1604
          tunnel: [_ _ _ _ _ w1837] -> w1603
          tunnel: [_ _ _ _ _ w1836] -> w1602
          tunnel: [_ _ _ _ _ w1835] -> w1601
          tunnel: w1600 -> [_ _ w1711 _ w1767 _]
          frame #0 {
            # "FABRIC"
            n965 = local read "fab1_totalWt"() -> (w1637:sgl)
            n966 = local read "fab3_totalWt"() -> (w1639:sgl)
            n967 = local read "fab5_totalWt"() -> (w1641:sgl)
            n968 = global read "BIMS_Collector Globals.vi" "LayerStitchTypeRefs"() -> (w1629:refnum<vi>[])
            n969 = global read "BIMS_Collector Globals.vi" "SampleAttribs"() -> (w1630:T29)
            n970 = global read "BIMS_Collector Globals.vi" "SampleStyles"() -> (w1632:refnum<vi>[])
            n971 = local read "fab2_totalWt"() -> (w1638:sgl)
            n972 = local read "fab4_totalWt"() -> (w1640:sgl)
            n973 = local read "fab6_totalWt"() -> (w1642:sgl)
            n974 = global read "BIMS_Collector Globals.vi" "LayerSpecs"() -> (w1631:T23)
            n975 = global read "BIMS_Collector Globals.vi" "Mfrs"() -> (w1633:refnum<vi>[])
            n976 = Build Array(w1637, w1638, w1639, w1640, w1641, w1642) -> (w1636:sgl[])
            n977 = for {
              tunnel: w1636 -> [w1644] mode=indexing
              tunnel: [w1650] -> w1635 mode=indexing
              tunnel: w1630 -> [w1648] mode=indexing
              tunnel: w1631 -> [w1647] mode=indexing
              tunnel: w1633 -> [w1646] mode=indexing
              tunnel: w1632 -> [w1645] mode=indexing
              tunnel: w1629 -> [w1643] mode=indexing
              n978 = Less Or Equal To 0?(x=w1644) -> (x <= 0?=w1649:bool)
              n979 = case shown="False" w1649 {
                tunnel: [w1672 w1674] -> w1650
                tunnel: w1648 -> [w1671 _]
                tunnel: w1647 -> [w1656 _]
                tunnel: w1646 -> [w1665 _]
                tunnel: w1645 -> [w1662 _]
                tunnel: w1644 -> [w1655 _]
                tunnel: w1643 -> [w1651 _]
                frame False {
                  n980 = Unbundle By Name(w1656) -> ("numOfPlies"=w1654:i32, "LotNum"=w1668:string, "RollNum"=w1669:string)
                  n981 = Unbundle By Name(w1671) -> ("internal_ID"=w1659:string, "fiber"=w1660:string, "denier"=w1667:string, "pick"=w1666:string, "weave"=w1657:string, "finish"=w1658:string, "ozPerYd2"=w1670:string)
                  n982 = Format Into String(w1654) -> (resulting string=w1664:string)  [unwired: 3 in, 1 out]
                  n983 = call "Dropdown Selection (SubVI).vi"("reference"=w1665) -> ("element"=w1663:string)
                  n984 = call "Dropdown Selection (SubVI).vi"("reference"=w1662) -> ("element"=w1661:string)
                  n985 = call "Dropdown Selection (SubVI).vi"("reference"=w1651) -> ("element"=w1652:string)
                  n986 = Format Into String(w1655) -> (resulting string=w1653:string)  [unwired: 3 in, 1 out]
                  n987 = Build Array(w1664, w1663, w1661, w1659, w1660, w1667, w1666, w1657, w1658, w1668, w1669, w1670, w1653, w1652) -> (w1672:string[])
                }
                frame True {
                  n988 = call <vilib>:"Space Constant.vi"() -> ("String"=w1675:string)
                  n989 = Initialize Array(w1675, 12 ("dimension size")) -> (w1674:string[])
                }
              }
            }
            n990 = Transpose 2D Array(2D array=w1635) -> (transposed array=w1634:string[][])
          }
          frame #1 {
            w1676 = "%.1f" ("format string")
            # "muzzel / midpoint"
            # "muzzle / scr#1"
            # "muzzle / target"
            # "scr#2 / target"
            # "RANGE"
            n991 = local read "Set#1 Separation"() -> (w1683:sgl)
            n992 = local read "mid_to_targ_dist"() -> (w1680:sgl)
            n993 = local read "Barrel to Screen"() -> (w1677:sgl)
            n994 = local read "clayAverage"() -> (w1698:sgl)
            n995 = Divide(x=w1683, y=sgl 2.0) -> (x/y=w1678:sgl)
            n996 = local read "RoomHum"() -> (w1693:sgl)
            n997 = local read "clayTemp"() -> (w1696:sgl)
            n998 = local read "clayCalib"() -> (w1699:string)
            n999 = local read "RoomT"() -> (w1694:sgl)
            n1000 = Add(x=w1677, y=w1680) -> (x+y=w1684:sgl)
            n1001 = Subtract(x=w1677, y=w1678) -> (x-y=w1679:sgl)
            n1002 = Subtract(x=w1680, y=w1678) -> (x-y=w1681:sgl)
            n1003 = Format Into String(w1684) -> (resulting string=w1685:string)  [unwired: 3 in, 1 out]
            n1004 = Format Into String(w1679) -> (resulting string=w1686:string)  [unwired: 3 in, 1 out]
            n1005 = Format Into String(w1683) -> (resulting string=w1687:string)  [unwired: 3 in, 1 out]
            n1006 = Format Into String(w1681) -> (resulting string=w1688:string)  [unwired: 3 in, 1 out]
            n1007 = Format Into String(w1680) -> (resulting string=w1689:string)  [unwired: 3 in, 1 out]
            n1008 = Format Into String(w1693) -> (resulting string=w1691:string)  [unwired: 3 in, 1 out]
            n1009 = Format Into String(format string=w1676, w1694) -> (resulting string=w1692:string)  [unwired: 2 in, 1 out]
            n1010 = Format Into String(format string=w1676, w1696) -> (resulting string=w1695:string)  [unwired: 2 in, 1 out]
            n1011 = Format Into String(format string=w1676, w1698) -> (resulting string=w1697:string)  [unwired: 2 in, 1 out]
            n1012 = Bundle(w1685, w1686, w1687, w1688, w1689, w1691, w1692, w1695, "clayCalib"=w1699, w1697) -> (w1700:T47)  [unwired: 1 out]
            n1013 = Cluster To Array(cluster=w1700) -> (array=w1690:string[])
          }
          frame #2 {
            # "RESULTS"
            n1014 = control-ref of="Methods"() -> (w1701:refnum<vi>)
            n1015 = call "Dropdown Selection (SubVI).vi"("reference"=w1701) -> ("element"=w1702:string)
            n1016 = for {
              tunnel: w1711 -> [w1739] mode=indexing
              tunnel: [w1738] -> w1710 mode=indexing
              tunnel: [w1737] -> w1709
              i -> [w1737]
              n1017 = Unbundle By Name(w1739) -> ("BackFace\nDepth"=w1738:sgl)
            }
            n1018 = Increment(x=w1709) -> (x+1=w1707:i32)
            n1019 = Add Array Elements(numeric array=w1710) -> (sum=w1708:sgl)
            n1020 = To Single Precision Float(number=w1707) -> (single precision float=w1706:sgl)
            n1021 = Divide(x=w1708, y=w1706) -> (x/y=w1705:sgl)
            n1022 = Format Into String(format string="%1.1f", w1705) -> (resulting string=w1704:string)  [unwired: 2 in, 1 out]
            n1023 = case shown="\"V50\"" w1702 {
              tunnel: [w1727 w1736] -> w1714
              tunnel: w1704 -> [w1715 w1735]
              frame "V50" {
                w1721 = "%1d" ("format string")
                n1024 = local read "Z.M.R."() -> (w1719:sgl)
                n1025 = Less Than 0?(x=w1719) -> (x < 0?=w1720:bool)
                n1026 = local read "rangeOfResults"() -> (w1723:i32)
                n1027 = local read "computed_V50"() -> (w1726:sgl)
                n1028 = local read "lowComplete"() -> (w1724:i32)
                n1029 = local read "highPartial"() -> (w1725:i32)
                n1030 = case shown="True" w1720 {
                  tunnel: w1719 -> [w1732 _]
                  tunnel: [w1732 sgl 0.0 ("Z.M.R.")] -> w1718
                  frame False {
                  }
                  frame True {
                  }
                }
                n1031 = Format Into String(format string="%1.1f", w1726) -> (resulting string=w1730:string)  [unwired: 2 in, 1 out]
                n1032 = Format Into String(format string=w1721, w1725) -> (resulting string=w1729:string)  [unwired: 2 in, 1 out]
                n1033 = Format Into String(format string=w1721, w1724) -> (resulting string=w1728:string)  [unwired: 2 in, 1 out]
                n1034 = Format Into String(format string=w1721, w1723) -> (resulting string=w1731:string)  [unwired: 2 in, 1 out]
                n1035 = Format Into String(format string="%1.1f", w1718) -> (resulting string=w1717:string)  [unwired: 2 in, 1 out]
                n1036 = Bundle(w1730, w1729, w1728, w1731, w1717, w1715, w1715) -> (w1727:T40)  [unwired: 1 out]
              }
              frame Default {
                w1734 = "" ("Empty String Constant")
                n1037 = Bundle(w1734, w1734, w1734, w1734, w1734, w1735, w1735) -> (w1736:T40)  [unwired: 1 out]
              }
            }
            n1038 = Cluster To Array(cluster=w1714) -> (array=w1713:string[])
            n1039 = Build Array(w1713) -> (w1712:string[][])
          }
          frame #3 {
            # "PB Req"
            # "SAMPLE"
            n1040 = control-ref of="Methods"() -> (w1742:refnum<vi>)
            n1041 = call "Dropdown Selection (SubVI).vi"("reference"=w1742) -> ("element"=w1744:string)
            n1042 = Equal?(x=w1744, y="V50") -> (x = y?=w1743:bool)
            n1043 = local read "totalSampleWt"() -> (w1754:sgl)
            n1044 = case shown="True" w1743 {
              tunnel: ["n/a" w1764] -> w1748
              frame False {
              }
              frame True {
                n1045 = local read "minV50"() -> (w1763:i32)
                n1046 = Format Into String(w1763) -> (resulting string=w1764:string)  [unwired: 3 in, 1 out]
              }
            }
            n1047 = local read "Type of work"() -> (w1740:string)
            n1048 = control-ref of="SampleDimensions"() -> (w1760:refnum<vi>)
            n1049 = control-ref of="SampleCoverings"() -> (w1761:refnum<vi>)
            n1050 = control-ref of="Models"() -> (w1747:refnum<vi>)
            n1051 = local read "serialNum"() -> (w1756:string)
            n1052 = local read "SampleID"() -> (w1758:string)
            n1053 = local read "Thickness"() -> (w1751:dbl)
            n1054 = local read "totalBAW"() -> (w1750:sgl)
            n1055 = call "Dropdown Selection (SubVI).vi"("reference"=w1760) -> ("element"=w1757:string)
            n1056 = call "Dropdown Selection (SubVI).vi"("reference"=w1747) -> ("element"=w1746:string)
            n1057 = call "Dropdown Selection (SubVI).vi"("reference"=w1761) -> ("element"=w1755:string)
            n1058 = Format Into String(w1754) -> (resulting string=w1753:string)  [unwired: 3 in, 1 out]
            n1059 = Format Into String(w1751) -> (resulting string=w1752:string)  [unwired: 3 in, 1 out]
            n1060 = Format Into String(w1750) -> (resulting string=w1749:string)  [unwired: 3 in, 1 out]
            n1061 = Bundle("SampleID"=w1758, "element"=w1757, "Type of work"=w1740, "serialNum"=w1756, "element"=w1746, w1753, w1752, w1749, "element"=w1755, w1748) -> (w1759:T41)  [unwired: 1 out]
            n1062 = Cluster To Array(cluster=w1759) -> (array=w1741:string[])
          }
          frame #4 {
            # "SHOT TABLE"
            n1063 = control-ref of="Methods"() -> (w1766:refnum<vi>)
            n1064 = call "Dropdown Selection (SubVI).vi"("reference"=w1766) -> ("element"=w1765:string)
            n1065 = for {
              tunnel: w1767 -> [w1806] mode=indexing
              shift-right: [w1783] -> _
              shift-left: T33 [] -> [w1785]
              tunnel: [w1783] -> w1770
              tunnel: w1765 -> [w1779]
              n1066 = Unbundle By Name(w1806) -> ("shot order"=w1805:i32, "Powder Loading"=w1804:sgl, "Uncorrected Impact"=w1803:sgl, "UncorrectedRed_PB"=w1802:sgl, "UncorrectedAvgVel_PB"=w1801:sgl, "velLoss_PB"=w1800:sgl, "strikeVel_PB"=w1799:sgl, "SHOT STATUS"=w1788:u16, "usedv50"=w1798:bool, "Shot Angle"=w1780:u16, "BackFace\nDepth"=w1781:sgl)
              n1067 = case shown="\"V50\"" w1779 {
                tunnel: w1798 -> [w1808 _]
                tunnel: [w1807 w1812] -> w1797
                tunnel: w1780 -> [_ w1811]
                frame "V50" {
                  n1068 = case shown="True" w1808 {
                    tunnel: ["" ("Empty String Constant") "*"] -> w1807
                    frame False {
                    }
                    frame True {
                    }
                  }
                }
                frame Default {
                  n1069 = Format Into String(w1811) -> (resulting string=w1812:string)  [unwired: 3 in, 1 out]
                }
              }
              n1070 = case shown="1" w1788 {
                tunnel: ["P" "C"] -> w1787
                frame 0, Default {
                }
                frame 1 {
                }
              }
              n1071 = Format Into String(format string="%2d", w1805) -> (resulting string=w1790:string)  [unwired: 2 in, 1 out]
              n1072 = Format Into String(w1804) -> (resulting string=w1791:string)  [unwired: 3 in, 1 out]
              n1073 = Format Into String(w1803) -> (resulting string=w1792:string)  [unwired: 3 in, 1 out]
              n1074 = Format Into String(w1802) -> (resulting string=w1793:string)  [unwired: 3 in, 1 out]
              n1075 = Format Into String(w1801) -> (resulting string=w1794:string)  [unwired: 3 in, 1 out]
              n1076 = Format Into String(w1800) -> (resulting string=w1795:string)  [unwired: 3 in, 1 out]
              n1077 = Format Into String(w1799) -> (resulting string=w1796:string)  [unwired: 3 in, 1 out]
              n1078 = Format Into String(w1781) -> (resulting string=w1789:string)  [unwired: 3 in, 1 out]
              n1079 = Build Array(w1790, w1791, w1792, w1793, w1794, w1795, w1796, w1787, w1797, w1789) -> (w1784:string[])
              n1080 = Array To Cluster(array=w1784) -> (cluster=w1786:T43)
              n1081 = Build Array (concatenate)(w1785, w1786) -> (w1783:T33)
            }
            n1082 = Array Size(array=w1770) -> (size(s)=w1772:i32)
            n1083 = Equal To 0?(x=w1772) -> (x = 0?=w1768:bool)
            n1084 = case shown="True" w1768 {
              tunnel: [w1775 T33 [{"[0]"="", "[1]"="", "[2]"="", "[3]"="", "[4]"="", "[5]"="", "[6]"="", "[7]"="", "[8]"="", "[9]"=""}]] -> w1769
              tunnel: w1770 -> [w1775 _]
              frame False {
              }
              frame True {
              }
            }
            n1085 = Sort 1D Array(array=w1769) -> (sorted array=w1771:T33)
            n1086 = for {
              tunnel: w1771 -> [w1778] mode=indexing
              tunnel: [w1777] -> w1774 mode=indexing
              n1087 = Cluster To Array(cluster=w1778) -> (array=w1777:string[])
            }
          }
          frame #5 {
            # "THREAT"
            # "Range # (supports a PB reporting requirement)"
            # "Project Name goes here.\nSupports a PB reporting requirement."
            # "GENERAL"
            n1088 = local read "threatDetails"() -> (w1816:T1)
            n1089 = Unbundle By Name(w1816) -> ("barrelLength"=w1820:string)
            n1090 = Unbundle By Name(w1816) -> ("grainSize"=w1815:string)
            n1091 = local read "Shot Angle"() -> (w1821:u16)
            n1092 = control-ref of="WeaponTypes"() -> (w1830:refnum<vi>)
            n1093 = control-ref of="ThreatGroups"() -> (w1829:refnum<vi>)
            n1094 = control-ref of="PowderTypes"() -> (w1828:refnum<vi>)
            n1095 = control-ref of="Recorders"() -> (w1831:refnum<vi>)
            n1096 = control-ref of="Shooters"() -> (w1832:refnum<vi>)
            n1097 = Format Into String(w1821) -> (resulting string=w1822:string)  [unwired: 3 in, 1 out]
            n1098 = call "Dropdown Selection (SubVI).vi"("reference"=w1830) -> ("element"=w1826:string)
            n1099 = call "Dropdown Selection (SubVI).vi"("reference"=w1829) -> ("element"=w1825:string)
            n1100 = call "Dropdown Selection (SubVI).vi"("reference"=w1828) -> ("element"=w1824:string)
            n1101 = call "Dropdown Selection (SubVI).vi"("reference"=w1831) -> ("element"=w1823:string)
            n1102 = call "Dropdown Selection (SubVI).vi"("reference"=w1832) -> ("element"=w1819:string)
            n1103 = Bundle("element"=w1826, "element"=w1825, "grainSize"=w1815, "element"=w1824, "barrelLength"=w1820, w1822, "element"="1", "element"=w1819, "element"=w1823) -> (w1827:T45)  [unwired: 1 out]
            n1104 = Cluster To Array(cluster=w1827) -> (array=w1817:string[])
            n1105 = local read "Comments"() -> (w1836:string)
            n1106 = local read "ProjectID"() -> (w1833:string)
            n1107 = local read "lastSamp"() -> (w1841:i32)
            n1108 = control-ref of="TestStandards"() -> (w1840:refnum<vi>)
            n1109 = control-ref of="Methods"() -> (w1839:refnum<vi>)
            n1110 = call "Dropdown Selection (SubVI).vi"("reference"=w1840) -> ("element"=w1835:string)
            n1111 = call "Dropdown Selection (SubVI).vi"("reference"=w1839) -> ("element"=w1838:string)
            n1112 = Increment(x=w1841) -> (x+1=w1837:i32)
          }
        }
        n1113 = To Variant(anything=w1624) -> (Variant=w1618:variant)
        n1114 = To Variant(anything=w1623) -> (Variant=w1617:variant)
        n1115 = To Variant(anything=w1622) -> (Variant=w1616:variant)
        n1116 = To Variant(anything=w1621) -> (Variant=w1615:variant)
        n1117 = To Variant(anything=w1620) -> (Variant=w1614:variant)
        n1118 = To Variant(anything=w1619) -> (Variant=w1613:variant)
        n1119 = To Variant(anything=w1606) -> (Variant=w1612:variant)
        n1120 = To Variant(anything=w1605) -> (Variant=w1611:variant)
        n1121 = To Variant(anything=w1604) -> (Variant=w1610:variant)
        n1122 = To Variant(anything=w1603) -> (Variant=w1607:variant)
        n1123 = To Variant(anything=w1602) -> (Variant=w1608:variant)
        n1124 = To Variant(anything=w1601) -> (Variant=w1609:variant)
        n1125 = call "TestReport_XL.vi"("Enable"=w1626, "blockFabric"=w1618, "blockRange"=w1617, "blockResults"=w1616, "blockSample"=w1615, "blockShotTbl"=w1614, "error in (no error)"=w1598, "blockThreat"=w1613, "method"=w1612, "projName"=w1611, "projNum"=w1610, "recNum"=w1607, "remark"=w1608, "standard"=w1609) -> ("error out"=w1625:errorcluster)  [unwired: 5 in, 8 out]
        n1126 = call <vilib>:"Simple Error Handler.vi"("error in (no error)"=w1625) -> ("error out"=w1627:errorcluster)  [unwired: 1 in, 7 out]
        n1127 = case shown="No Error" w1627 {
          selector: w1627 -> [w1842 w1844]
          tunnel: [w1842 w1844] -> w1597
          frame No Error {
            n1128 = One Button Dialog(message=" VsVr Ballistic Test Report is ready") -> ()  [unwired: 2 out]
          }
          frame Error {
          }
        }
      }
      frame "SAVE SHOTS" {
        # "case # 4"
        # "This section saves the shots to the data base"
        n1129 = stacked-sequence {
          seq-local: [w1887 _ _] -> [_ w1973 _]
          seq-local: [w1889 _ _] -> [_ w1970 _]
          seq-local: [_ w1958 _] -> [_ _ w1987]
          seq-local: [_ w1960 _] -> [_ _ w1986]
          seq-local: [w1885 _ _] -> [_ _ w1979]
          seq-local: [w1859 _ _] -> [_ w1916 _]
          tunnel: [_ _ w1981] -> w1849
          tunnel: [_ _ w1984] -> w1850
          tunnel: w1846 -> [_ w1925 w1978]
          tunnel: w1848 -> [w1861 _ _]
          frame #0 {
            # "Legacy requirements:"
            # "Shared requirements:"
            n1130 = local read "fab1_totalWt"() -> (w1897:sgl)
            n1131 = local read "fab2_totalWt"() -> (w1896:sgl)
            n1132 = local read "fab3_totalWt"() -> (w1895:sgl)
            n1133 = local read "fab4_totalWt"() -> (w1894:sgl)
            n1134 = local read "fab5_totalWt"() -> (w1893:sgl)
            n1135 = local read "fab6_totalWt"() -> (w1892:sgl)
            n1136 = Build Array(w1897, w1896, w1895, w1894, w1893, w1892) -> (w1891:sgl[])
            n1137 = call "SQL Statement for Sample Descritpion.vi"("error IN"=w1861, "Layer Weight Array"=w1891, "VALUES clause IN"=" VALUES (%d " ("SQL statement IN"), "INSERT clause IN"="INSERT INTO Experiments " ("SQL statement IN")) -> ("error OUT"=w1860:errorcluster, "VALUES clause OUT"=w1890:string, "INSERT clause OUT"=w1888:string)  [unwired: 1 out]
            n1138 = local read "lastSamp"() -> (w1886:i32)
            n1139 = Increment(x=w1886) -> (x+1=w1885:i32)
            n1140 = local read "rangeOfResults"() -> (w1863:i32)
            n1141 = local read "lowComplete"() -> (w1864:i32)
            n1142 = local read "clayAverage"() -> (w1866:sgl)
            n1143 = local read "highPartial"() -> (w1865:i32)
            n1144 = control-ref of="SampleClamping"() -> (w1858:refnum<vi>)
            n1145 = control-ref of="BackLayer"() -> (w1856:refnum<vi>)
            n1146 = control-ref of="FrontLayer"() -> (w1855:refnum<vi>)
            n1147 = control-ref of="Ballisticians"() -> (w1880:refnum<vi>)
            n1148 = control-ref of="Shooters"() -> (w1876:refnum<vi>)
            n1149 = control-ref of="Recorders"() -> (w1875:refnum<vi>)
            n1150 = control-ref of="Submitters"() -> (w1879:refnum<vi>)
            n1151 = control-ref of="SampleCoverings"() -> (w1872:refnum<vi>)
            n1152 = control-ref of="ThreatGroups"() -> (w1871:refnum<vi>)
            n1153 = call "Dropdown Selection (SubVI).vi"("reference"=w1880) -> ("element"=w1878:string)
            n1154 = call "Dropdown Selection (SubVI).vi"("reference"=w1876) -> ("element"=w1874:string)
            n1155 = call "Dropdown Selection (SubVI).vi"("reference"=w1875) -> ("element"=w1873:string)
            n1156 = call "Dropdown Selection (SubVI).vi"("reference"=w1879) -> ("element"=w1877:string)
            n1157 = call "Dropdown Selection (SubVI).vi"("reference"=w1872) -> ("element"=w1870:string)
            n1158 = call "Dropdown Selection (SubVI).vi"("reference"=w1871) -> ("element"=w1869:string)
            n1159 = call "Dropdown Selection (SubVI).vi"("reference"=w1858) -> ("element"=w1857:string)
            n1160 = call "Dropdown Selection (SubVI).vi"("reference"=w1856) -> ("element"=w1854:string)
            n1161 = call "Dropdown Selection (SubVI).vi"("reference"=w1855) -> ("element"=w1853:string)
            n1162 = Format Into String(format string=", %d, #%s#, '%s', '%s', '%s', '%s', '%s', '%s', %.1f, '%s', %.1f, %d, %d, %d, '%s', '%s', '%s'" ("Format String"), initial string=w1890, error in=w1860, w1885, "shotTimestamp", w1878, w1874, w1873, w1877, w1870, w1869, "clayTemp", "clayCalib", w1866, w1865, w1864, w1863, w1857, w1854, w1853) -> (resulting string=w1889:string, error out=w1859:errorcluster)
            n1163 = Concatenate Strings(w1888, ", expt, [date], Ballistician1, Ballistician2, Ballistician3, Submitter1, SampleCovering, ProjectileType, ClayTemp, ClayCalibration, ClayAvgThickness, highPartial, lowComplete, rangeOfResults, clamping, FrontPly, BackPly," ("Substring")) -> (w1887:string)
            n1164 = flat-sequence {
              tunnel: ["TestStandards"] -> _
              tunnel: ["Shooters"] -> _
              tunnel: ["Recorders"] -> _
              tunnel: ["WeaponTypes"] -> _
              tunnel: ["Models"] -> _
              tunnel: ["serialNum"] -> _
              tunnel: ["layerStitch_1"] -> _
              tunnel: ["layerStitch_2"] -> _
              tunnel: ["layerStitch_3"] -> _
              tunnel: ["layerStitch_4"] -> _
              tunnel: ["layerStitch_5"] -> _
              tunnel: ["layerStitch_6"] -> _
              tunnel: ["minV50"] -> _
              frame #0 {
                # "PB-only requirements:"
              }
            }
          }
          frame #1 {
            w1972 = " Angle, Conditions, SampleType, ThreatGrain, ThreatDetail, V50dc, V50, maker, thickness, powder, numshots, backing, totalnumberplys, testcomments, NIJ1, method, temperature, humidity, Dimensions, zmr, ProjectID, SampleID, panelmaker, panelWeight, totalBAW)"  # INSERT clause continued
            # "Although shot angle is defined for the overall\nexperiment, it is also recorded for each shot."
            n1165 = local read "computed_V50"() -> (w1968:sgl)
            n1166 = local read "Drag Corrected"() -> (w1963:bool)
            n1167 = local read "Impact factor"() -> (w1965:sgl)
            n1168 = Array Size(array=w1925) -> (size(s)=w1956:i32)
            n1169 = Select(t=w1965, s=w1963, f=sgl 1.0) -> (s? t:f=w1964:sgl)
            n1170 = Divide(x=w1968, y=w1964) -> (x/y=w1967:sgl)
            n1171 = control-ref of="ModelMfrs"() -> (w1951:refnum<vi>)
            n1172 = control-ref of="PowderTypes"() -> (w1949:refnum<vi>)
            n1173 = call "Dropdown Selection (SubVI).vi"("reference"=w1951) -> ("element"=w1950:string)
            n1174 = call "Dropdown Selection (SubVI).vi"("reference"=w1949) -> ("element"=w1933:string)
            n1175 = local read "GrainSize"() -> (w1914:u16)
            n1176 = local read "Z.M.R."() -> (w1939:sgl)
            n1177 = local read "Shot Angle"() -> (w1927:u16)
            n1178 = Less Than 0?(x=w1939) -> (x < 0?=w1938:bool)
            n1179 = local read "totalNumLayers"() -> (w1955:i32)
            n1180 = control-ref of="ThreatDetails"() -> (w1911:refnum<vi>)
            n1181 = control-ref of="SampleTypes"() -> (w1921:refnum<vi>)
            n1182 = control-ref of="TestConditions"() -> (w1940:refnum<vi>)
            n1183 = control-ref of="SampleBackings"() -> (w1948:refnum<vi>)
            n1184 = Format Into String(w1914) -> (resulting string=w1913:string)  [unwired: 3 in, 1 out]
            n1185 = local read "totalBAW"() -> (w1941:sgl)
            n1186 = case shown="True" w1938 {
              tunnel: w1939 -> [w1976 _]
              tunnel: [w1976 sgl 0.0 ("Z.M.R.")] -> w1937
              frame False {
              }
              frame True {
              }
            }
            n1187 = control-ref of="SampleDimensions"() -> (w1944:refnum<vi>)
            n1188 = control-ref of="N.I.J"() -> (w1946:refnum<vi>)
            n1189 = control-ref of="Methods"() -> (w1931:refnum<vi>)
            n1190 = control-ref of="Assemblers"() -> (w1942:refnum<vi>)
            n1191 = call "Dropdown Selection (SubVI).vi"("reference"=w1911) -> ("element"=w1912:string)
            n1192 = call "Dropdown Selection (SubVI).vi"("reference"=w1921) -> ("element"=w1920:string)
            n1193 = call "Dropdown Selection (SubVI).vi"("reference"=w1940) -> ("element"=w1926:string)
            n1194 = call "Dropdown Selection (SubVI).vi"("reference"=w1948) -> ("element"=w1947:string)
            n1195 = Equal?(x=w1913, y="") -> (x = y?=w1935:bool)
            n1196 = call "Dropdown Selection (SubVI).vi"("reference"=w1946) -> ("element"=w1945:string)
            n1197 = call "Dropdown Selection (SubVI).vi"("reference"=w1931) -> ("element"=w1930:string)
            n1198 = call "Dropdown Selection (SubVI).vi"("reference"=w1944) -> ("element"=w1943:string)
            n1199 = call "Dropdown Selection (SubVI).vi"("reference"=w1942) -> ("element"=w1932:string)
            n1200 = case shown="False" w1935 {
              tunnel: [w1974 "0" ("element")] -> w1934
              tunnel: w1913 -> [w1974 _]
              frame False {
              }
              frame True {
              }
            }
            n1201 = call "Prepare DB Connect Path (SubVI).vi"("connectString"=path "BIMS_Collector.udl", "error in"=w1916) -> ("appended path"=w1915:path, "error out"=w1917:errorcluster)  [unwired: 1 out]
            n1202 = Format Into String(format string=", %d, '%s', '%s', '%s', '%s', %.4f, %.1f, '%s', %.4f, '%s', %d, '%s', %d, '%s', '%s', '%s', %.1f, %.1f, '%s', %.1f, '%s', '%s', '%s', %.1f, %.1f);" ("Format String"), initial string=w1970, error in=w1917, w1927, w1926, w1920, w1934, w1912, w1968, w1967, w1950, "Thickness", w1933, w1956, w1947, w1955, "Comments", w1945, w1930, "RoomT", "RoomHum", w1943, w1937, "ProjectID", "SampleID", w1932, "totalSampleWt", w1941) -> (resulting string=w1969:string, error out=w1919:errorcluster)
            n1203 = call-poly <vilib>:"DB Tools Open Connection.vi"("error in (no error)"=w1919, "connection information"=w1915) -> ("error out"=w1928:errorcluster, "connection reference"=w1929:T48)  [unwired: 3 in, 3 out]
            n1204 = Concatenate Strings(w1973, w1972, w1969) -> (w1962:string)
            n1205 = call-poly <vilib>:"DB Tools Execute Query.vi"("error in (no error)"=w1928, "SQL query"=w1962, "connection reference"=w1929) -> ("error out"=w1961:errorcluster, "recordset reference"=w1959:T49)  [unwired: 1 in, 4 out]
            n1206 = call-poly <vilib>:"DB Tools Free Object.vi"("error in (no error)"=w1961, "recordset reference"=w1959) -> ("error out"=w1960:errorcluster, "connection reference"=w1958:T48)  [unwired: 8 out]
          }
          frame #2 {
            # "Experiment.expt"
            n1207 = local read "lastShot"() -> (w1985:i32)
            n1208 = Increment(x=w1985) -> (x+1=w1983:i32)
            n1209 = for {
              tunnel: w1978 -> [w2031] mode=indexing
              tunnel: w1987 -> [w2006]
              tunnel: w1986 -> [w1990]
              tunnel: [w2004] -> w1980
              tunnel: [w2005] -> w1982
              tunnel: w1983 -> [w2011]
              tunnel: [w2003] -> w1984
              tunnel: w1979 -> [w1999]
              i -> [w2003]
              w1991 = sgl 1.0 ("f")
              # "Shot.id"
              n1210 = Add(x=w2011, y=w2003) -> (x+y=w2010:i32)
              n1211 = Unbundle By Name(w2031) -> ("IMPACT VELOCITY"=w2017:sgl, "Redundant_Velocity"=w1996:sgl, "RESIDUAL  VELOCITY"=w1995:sgl, "Shot Description"=w1997:string, "Powder Loading"=w2021:sgl, "Barrel Temperature"=w2022:sgl, "TIME / DATE"=w2023:string, "shot order"=w2024:i32, "Shot Angle"=w2025:u16, "BackFace\nDepth"=w2026:sgl, "BackFace\nDiameter"=w2027:sgl, "SHOT STATUS"=w2029:u16, "Projectile Mass"=w2020:sgl, "usedv50"=w2019:bool, "Energy Loss (J)"=w2018:sgl, "avgVel_PB"=w2002:sgl, "velLoss_PB"=w2001:sgl, "strikeVel_PB"=w2000:sgl, "Frag Rod"=w1988:sgl)
              n1212 = local read "Drag Corrected"() -> (w1993:bool)
              n1213 = local read "Residual factor"() -> (w2015:sgl)
              n1214 = local read "Impact factor"() -> (w1992:sgl)
              n1215 = Select(t=w1992, s=w1993, f=w1991) -> (s? t:f=w2013:sgl)
              n1216 = Select(t=w1992, s=w1993, f=w1991) -> (s? t:f=w1998:sgl)
              n1217 = Select(t=w2015, s=w1993, f=w1991) -> (s? t:f=w2014:sgl)
              n1218 = Divide(x=w2017, y=w2013) -> (x/y=w2012:sgl)
              n1219 = Divide(x=w1996, y=w1998) -> (x/y=w1994:sgl)
              n1220 = Divide(x=w1995, y=w2014) -> (x/y=w2016:sgl)
              n1221 = Greater Than 0?(x=w2029) -> (x > 0?=w2028:bool)
              n1222 = Format Into String(format string="INSERT INTO shots (impactdc, redundantdc, residualdc,  comment, loading, barreltemp, [date], [order], shotangle, bfdepth, bfdiameter, [complete], expt, id, weight,usedv50, loss, residual, impact, redundant, avgVel_PB, velLoss_PB, strikeVel_PB, fragRod)  VALUES (%.1f, %.1f, %.1f, '%s', %.4f, %.1f, #%s#, %d, %d, %.3f, %.3f, %d, %d, %d, %.4f, %d, %.4f, %.1f, %.1f, %.1f, %.1f, %.1f, %.1f, %.1f)" ("Substring"), error in=w1990, w2017, w1996, w1995, w1997, w2021, w2022, w2023, w2024, w2025, w2026, w2027, w2028, w1999, w2010, w2020, w2019, w2018, w2016, w2012, w1994, w2002, w2001, w2000, w1988) -> (resulting string=w2007:string, error out=w1989:errorcluster)  [unwired: 1 in]
              n1223 = call-poly <vilib>:"DB Tools Execute Query.vi"("error in (no error)"=w1989, "SQL query"=w2007, "connection reference"=w2006) -> ("error out"=w2009:errorcluster, "recordset reference"=w2008:T49)  [unwired: 1 in, 4 out]
              n1224 = call-poly <vilib>:"DB Tools Free Object.vi"("error in (no error)"=w2009, "recordset reference"=w2008) -> ("error out"=w2004:errorcluster, "connection reference"=w2005:T48)  [unwired: 8 out]
            }
            n1225 = call <vilib>:"DB Tools Close Connection.vi"("error in (no error)"=w1980, "connection reference"=w1982) -> ("error out"=w1981:errorcluster)  [unwired: 5 out]
          }
        }
        n1226 = case shown="No Error" w1849 {
          selector: w1849 -> [w2043 w2062]
          tunnel: [-1 -1] -> w1851
          tunnel: [Collector_State."POLL" ("progState") Collector_State."POLL" ("progState")] -> w1852
          tunnel: w1850 -> [w2046 _]
          tunnel: [w2039 w2060] -> w1847
          tunnel: w1846 -> [w2038 w2059]
          tunnel: [w2036 w2059] -> w1845
          frame No Error {
            n1227 = local read "lastSamp"() -> (w2045:i32)
            n1228 = local read "configPath"() -> (w2033:path)
            n1229 = local read "lastShot"() -> (w2047:i32)
            n1230 = flat-sequence {
              tunnel: w2039 -> [_]
              tunnel: w2035 -> [w2057]
              tunnel: [w2057] -> w2036
              frame #0 {
                w2050 = T16."Disabled and Grayed Out" ("Disabled")
                n1231 = property on="saveReq" class="Str"("Visible"=TRUE) -> ()  [unwired: 2 in, 2 out]
                n1232 = local write "SampleID"("") -> ()
                n1233 = property on="clearShots" class="Bool"("Disabled"=T16."Enabled") -> ()  [unwired: 2 in, 2 out]
                n1234 = property on="addShot" class="Bool"("Disabled"=w2050) -> ()  [unwired: 2 in, 2 out]
                n1235 = property on="undoLastShot" class="Bool"("Disabled"=w2050) -> ()  [unwired: 2 in, 2 out]
                n1236 = property on="saveShots" class="Bool"("Disabled"=w2050) -> ()  [unwired: 2 in, 2 out]
                n1237 = property on="mainTabCntrl" class="TabCtl (strict)"("Val(Sgnl)"=enum32{"Setup", "Measure", "History", "System"}."Setup" ("mainTabCntrl")) -> ()  [unwired: 2 in, 2 out]
                n1238 = One Button Dialog(message="Data Saved. Enter new Sample ID.") -> ()  [unwired: 1 in, 1 out]
                n1239 = property on="SampleEntryTabCntrl" class="TabCtl (strict)"("Value"=enum32{"Environment", "Sample"}."Sample" ("SampleEntryTabCntrl")) -> ()  [unwired: 2 in, 2 out]
                n1240 = property on="Sample SubTabCntrl" class="TabCtl (strict)"("Value"=T2."General Specification" ("Sample SubTabCntrl")) -> ()  [unwired: 2 in, 2 out]
              }
            }
            n1241 = Array Size(array=w2038) -> (size(s)=w2037:i32)
            n1242 = Increment(x=w2047) -> (x+1=w2044:i32)
            n1243 = for {
              N: w2037 -> [_]
              shift-right: [w2048] -> w2035
              shift-left: w2038 -> [w2049]
              n1244 = Delete From Array(array=w2049) -> (array with subset deleted=w2048:T6)  [unwired: 2 in, 1 out]
            }
            n1245 = Add(x=w2044, y=w2046) -> (x+y=w2034:i32)
            n1246 = Increment(x=w2045) -> (x+1=w2032:i32)
            n1247 = local write "lastShot"(w2034) -> ()
            n1248 = call "save stats to INI (SubVI).vi"("lastSamp"=w2032, "errIN"=w2043, "lastShot"=w2034, "configPath"=w2033) -> ("errOUT"=w2039:errorcluster, "recordNum"=w2042:dbl)  [unwired: 6 in]
            n1249 = property on="Record #" class="DigNum (strict)"("Maximum"=w2042) -> ()  [unwired: 2 in, 2 out]
            n1250 = local write "lastSamp"(w2032) -> ()
            n1251 = property on="shotsArr" class="Arr (strict)"("Val(Sgnl)"=w2035) -> ()  [unwired: 2 in, 2 out]
          }
          frame Error {
            n1252 = One Button Dialog(message="Error saving Data. ") -> ()  [unwired: 2 out]
            n1253 = call <vilib>:"General Error Handler.vi"("error in (no error)"=w2062) -> ("error out"=w2060:errorcluster)  [unwired: 2 in, 12 out]
          }
        }
      }
      frame "ADD SHOT" {
        # "case # 5"
        # "Shot Order"
        # "This section accepts new data to the shot table."
        n1254 = local read "Impact/speed"() -> (w2106:sgl)
        n1255 = local read "residual/speed"() -> (w2102:sgl)
        n1256 = property on="undoLastShot" class="Bool"(error in=w2081, "Disabled"=T16."Enabled") -> (error out=w2080:errorcluster)  [unwired: 1 in, 1 out]
        n1257 = local read "Current/residual/speed"() -> (w2091:sgl)
        n1258 = local read "CorrectedVelScrnSet1"() -> (w2092:sgl)
        n1259 = local read "CorrectedVelScrnSet2"() -> (w2111:sgl)
        n1260 = local read "Current/avg/speed"() -> (w2113:sgl)
        n1261 = local read "Corrected Residual"() -> (w2090:sgl)
        n1262 = local read "Redundant/speed"() -> (w2110:sgl)
        n1263 = local read "conversion factor"() -> (w2100:sgl)
        n1264 = local read "MeasVelScrnSet1"() -> (w2109:sgl)
        n1265 = local read "MeasVelScrnSet2"() -> (w2108:sgl)
        n1266 = local read "Projectile Mass"() -> (w2082:sgl)
        n1267 = case shown="\"grains\"" "loadingUnits" {
          tunnel: [w2119 w2120] -> w2076
          tunnel: "Powder Loading" -> [w2119 w2121]
          frame "grams", Default {
            # "Always save in grams."
          }
          frame "grains" {
            # "Always save in grams."
            n1268 = Multiply(x=w2121, y=sgl 0.06479891) -> (x*y=w2120:sgl)
          }
        }
        n1269 = control-ref of="N.I.J"() -> (w2068:refnum<vi>)
        n1270 = local read "Avg/speed"() -> (w2112:sgl)
        n1271 = Array Size(array=w2085) -> (size(s)=w2088:i32)
        n1272 = call "Dropdown Selection (SubVI).vi"("reference"=w2068) -> ("element"=w2067:string)
        n1273 = Multiply(x=w2106, y=w2100) -> (x*y=w2098:sgl)
        n1274 = Multiply(x=w2100, y=w2102) -> (x*y=w2099:sgl)
        n1275 = Equal?(x=w2067, y="PASS") -> (x = y?=w2065:bool)
        n1276 = Increment(x=w2088) -> (x+1=w2107:i32)
        n1277 = Multiply(x=w2098, y=w2098) -> (x*y=w2094:sgl)
        n1278 = Multiply(x=w2099, y=w2099) -> (x*y=w2095:sgl)
        n1279 = Subtract(x=w2094, y=w2095) -> (x-y=w2096:sgl)
        n1280 = Compound Arithmetic op=MULTIPLY(w2082, w2096, sgl 0.0005 ("Input")) -> (w2101:sgl)
        n1281 = Format Date/Time String(time format string (%c)="%x   %H:%M:%S") -> (date/time string=w2103:string)  [unwired: 2 out]
        "SUBMIT DATE/TIME" <- w2103
        n1282 = Index Array(array=w2085) -> (element=w2087:T7)  [unwired: 1 in]
        n1283 = Bundle By Name(cluster=w2087, "TIME / DATE"=w2103, "shot order"=w2107, "IMPACT VELOCITY"=w2106, "RESIDUAL  VELOCITY"=w2102, "Shot Description"="Shot Description", "Powder Loading"=w2076, "Barrel Temperature"="Barrel Temp", "SHOT STATUS"="Current/shotstatus", "BackFace\nDepth"="backdepth", "Shot Angle"="Shot Angle", "Uncorrected Impact"=w2109, "Corrected Impact"=w2092, "Uncorrected Residual"=w2091, "Corrected residual"=w2090, "Projectile Mass"=w2082, "Energy Loss (J)"=w2101, "UncorrectedRed_PB"=w2108, "Redundant_Velocity"=w2110, "CorrectedRed_PB"=w2111, "UncorrectedAvgVel_PB"=w2113, "avgVel_PB"=w2112, "Frag Rod"="Frag Rod", "V50userExcl"=FALSE, "fairHit"=w2065) -> (w2089:T7)
        n1284 = Build Array (concatenate)(w2085, w2089) -> (w2072:T6)
        n1285 = flat-sequence {
          tunnel: w2080 -> [w2117]
          tunnel: [w2116] -> w2079
          tunnel: w2072 -> [w2114]
          tunnel: [w2114] -> w2071
          frame #0 {
            n1286 = local write "backdepth"(sgl 0.0 ("BACKFACE DEPTH")) -> ()
            n1287 = property on="shotsTabCntrl" class="TabCtl (strict)"(error in=w2117, "Value"=T5."Shots Table" ("shotsTabCntrl")) -> (error out=w2116:errorcluster)  [unwired: 1 in, 1 out]
          }
        }
      }
      frame "CLEAR SHOTS" {
        # "case # 6"
        # "This section will clear the shot table and re-enable the \"ADD SHOT\" button to get ready for a new test panel."
        n1288 = Two Button Dialog(message="Shot table cleared even if not saved. Are you sure?", 1:"NO" ("F button name (\"Cancel\")"), 2:"YES" ("T button name (\"OK\")")) -> (T button?=w2126:bool)
        n1289 = case shown="True" w2126 {
          tunnel: [w2132 T6 [{"Uncorrected Impact"=0.0, "Uncorrected Residual"=0.0, "avgVel_PB"=0.0, "IMPACT VELOCITY"=0.0, "RESIDUAL  VELOCITY "=0.0, "Shot Description"="", "Powder Loading "=0.0, "Barrel Temperature"=0.0, "TIME / DATE"="", "shot order"=1, "SHOT STATUS"=1, "Shot Angle"=0, "Corrected Impact"=0.0, "Corrected residual"=0.0, "Projectile Mass"=0.0, "usedv50"=FALSE, "Energy Loss (J)"=0.0, "BackFace\nDepth"=0.0, "BackFace\nDiameter"=0.0, "Redundant_Velocity"=0.0, "velLoss_PB"=0.0, "strikeVel_PB"=0.0, "UncorrectedRed_PB"=0.0, "CorrectedRed_PB"=0.0, "UncorrectedAvgVel_PB"=0.0, "V50userExcl"=FALSE, "Frag Rod"=0.0, "fairHit"=FALSE}] ("shotsArr")] -> w2131
          tunnel: w2127 -> [w2132 _]
          frame False {
          }
          frame True {
            w2134 = T16."Disabled and Grayed Out" ("Disabled")
            n1290 = invoke on="Table of Shots" class="Tbl (strict)" method="Reinit To Default"() -> ()  [unwired: 3 in, 3 out]
            n1291 = property on="addShot" class="Bool"("Disabled"=T16."Enabled") -> ()  [unwired: 2 in, 2 out]
            n1292 = invoke on="shotsArr" class="Arr (strict)" method="Reinit To Default"() -> ()  [unwired: 3 in, 3 out]
            n1293 = property on="saveReq" class="Str"("Visible"=TRUE) -> ()  [unwired: 2 in, 2 out]
            n1294 = property on="clearShots" class="Bool"("Disabled"=w2134) -> ()  [unwired: 2 in, 2 out]
            n1295 = property on="undoLastShot" class="Bool"("Disabled"=w2134) -> ()  [unwired: 2 in, 2 out]
            n1296 = property on="saveShots" class="Bool"("Disabled"=w2134) -> ()  [unwired: 2 in, 2 out]
          }
        }
      }
      frame "NEXT SHOT" {
        # "case # 7"
        n1297 = property on="shotsArr" class="Arr (strict)"(error in=w2140) -> (error out=w2139:errorcluster, "Index Values"=w2144:u32[])  [unwired: 1 in, 1 out]
        n1298 = Array Size(array=w2137) -> (size(s)=w2147:i32)
        n1299 = Index Array "Index Array"(array=w2144) -> (element=w2149:u32)  [unwired: 1 in]
        n1300 = To Unsigned Long Integer(number=w2147) -> (unsigned 32bit integer=w2143:u32)
        n1301 = Increment(x=w2149) -> (x+1=w2148:u32)
        n1302 = Quotient & Remainder(x=w2148, y=w2143) -> (x-y*floor(x/y)=w2146:u32)  [unwired: 1 out]
        n1303 = Replace Array Subset "Replace Array Subset"(array=w2144, new element=w2146) -> (w2145:u32[])  [unwired: 1 in]
        n1304 = property on="shotsArr" class="Arr (strict)"(error in=w2139, "Index Values"=w2145) -> (error out=w2138:errorcluster)  [unwired: 1 in, 1 out]
      }
      frame "DELETE SHOT" {
        # "case # 8"
        # "This section undoes new shot data OR deletes the currently accessed previous shot"
        n1305 = local read "deleteShot"() -> (w2156:bool)
        n1306 = case shown="False" w2156 {
          tunnel: w2155 -> [w2160 w2171]
          tunnel: [w2161 w2172] -> w2152
          frame False {
            n1307 = Array Size(array=w2160) -> (size(s)=w2158:i32)
            n1308 = while {
              tunnel: [w2162] -> w2159
              tunnel: w2158 -> [w2164]
              tunnel: w2160 -> [w2166] mode=indexing
              i -> [w2162]
              stop <- w2165 stop-if-true
              n1309 = Unbundle By Name(w2166) -> ("shot order"=w2163:i32)
              n1310 = Equal?(x=w2163, y=w2164) -> (x = y?=w2165:bool)
            }
            n1311 = Delete From Array "Delete From Array"(array=w2160, index=w2159) -> (array with subset deleted=w2161:T6)  [unwired: 1 in, 1 out]
            n1312 = property on="undoLastShot" class="Bool"("Disabled"=T16."Disabled and Grayed Out") -> ()  [unwired: 2 in, 2 out]
          }
          frame True {
            n1313 = property on="shotsArr" class="Arr (strict)"() -> ("Index Values"=w2180:u32[])  [unwired: 2 in, 2 out]
            n1314 = local write "deleteShot"(FALSE) -> ()
            n1315 = Index Array(array=w2180, index=0 ("Index")) -> (element=w2170:u32)
            n1316 = To Long Integer(number=w2170) -> (32bit integer=w2167:i32)
            n1317 = Index Array(array=w2171, index=w2167) -> (element=w2169:T7)
            n1318 = Unbundle By Name(w2169) -> ("shot order"=w2168:i32)
            n1319 = Format Into String(format string="The currently displayed Shot, #%d", w2168) -> (resulting string=w2177:string)  [unwired: 2 in, 1 out]
            n1320 = Concatenate Strings(w2177, ", will be deleted.  IT CANNOT RECOVERED!  Do you want to DELETE the shot?" ("message")) -> (w2176:string)
            n1321 = Two Button Dialog(message=w2176, 1:"NO I do NOT want to delete.  Cancel Request" ("F button name (\"Cancel\")"), 2:"YES I want to delete the shot" ("T button name (\"OK\")")) -> (T button?=w2183:bool)
            n1322 = case shown="True" w2183 {
              tunnel: w2171 -> [w2196 w2199]
              tunnel: [w2196 w2201] -> w2174
              tunnel: w2167 -> [_ w2198]
              tunnel: [10000 ("shot order") w2200] -> w2173
              frame False {
              }
              frame True {
                n1323 = Index Array(array=w2199, index=w2198) -> (element=w2197:T7)
                n1324 = Unbundle By Name(w2197) -> ("shot order"=w2200:i32)
                n1325 = Delete From Array(array=w2199, index=w2198) -> (array with subset deleted=w2201:T6)  [unwired: 1 in, 1 out]
              }
            }
            n1326 = for {
              tunnel: [w2190] -> w2172 mode=indexing
              tunnel: w2174 -> [w2185] mode=indexing
              tunnel: w2173 -> [w2189]
              n1327 = Unbundle By Name(w2185) -> ("shot order"=w2187:i32)
              n1328 = Decrement(x=w2187) -> (x-1=w2186:i32)
              n1329 = Greater?(x=w2187, y=w2189) -> (0:w2188:bool)
              n1330 = case shown="True" w2188 {
                tunnel: w2186 -> [_ w2193]
                tunnel: w2185 -> [w2191 w2194]
                tunnel: [w2191 w2192] -> w2190
                frame False {
                }
                frame True {
                  n1331 = Bundle By Name(cluster=w2194, "shot order"=w2193) -> (w2192:T7)
                }
              }
            }
          }
        }
        n1332 = property on="shotsArr" class="Arr (strict)"(error in=w2151, "Val(Sgnl)"=w2152) -> (error out=w2150:errorcluster)  [unwired: 1 in, 1 out]
      }
      frame "READY CLOCK" {
        # "case # 9"
        n1333 = case shown="\"Screens\"" "MeasSrc" {
          tunnel: w2203 -> [w2210 w2215 w2217]
          tunnel: [w2208 w2215 w2217] -> w2202
          frame "Simulated", Default {
            n1334 = flat-sequence {
              tunnel: w2210 -> [w2211]
              tunnel: [w2211] -> w2209
              tunnel: [w2213] -> w2208
              tunnel: w2209 -> [w2213]
              frame #0 {
                n1335 = local write "readyClock"(FALSE ("RANGE RESET")) -> ()
              }
              frame #1 {
                n1336 = Wait (ms)(milliseconds to wait=u32 100) -> ()  [unwired: 1 out]
              }
            }
          }
          frame "Radar" {
          }
          frame "Screens" {
            n1337 = local write "readyClock"(FALSE ("RANGE RESET")) -> ()
          }
        }
      }
      frame "PROC SHOTS" {
        # "case # 10"
        n1338 = local write "processShots"(FALSE ("ProcessShots")) -> ()
        n1339 = local read "Drag Corrected"() -> (w2223:bool)
        n1340 = stacked-sequence {
          seq-local: [_ w2281 _ _] -> [_ _ w2314 w2364]
          seq-local: [w2226 _ _ _] -> [_ w2277 _ _]
          seq-local: [w2244 _ _ _] -> [_ w2278 _ _]
          seq-local: [w2245 _ _ _] -> [_ w2279 _ _]
          tunnel: [_ _ _ w2357] -> w2224
          tunnel: w2223 -> [w2247 w2280 _ _]
          tunnel: w2220 -> [_ w2276 _ _]
          tunnel: w2219 -> [w2243 _ _ _]
          tunnel: [w2243 _ _ _] -> w2218
          frame #0 {
            n1341 = disable-structure "Diagram Disable Structure" shown="Enabled" {
              disable-tunnel: [w2264 w2271] -> w2252
              frame Disabled {
                n1342 = local read "factor array"() -> (w2266:sgl[])
                n1343 = local read "Threat"() -> (w2263:u16)
                n1344 = To Long Integer(number=w2263) -> (32bit integer=w2265:i32)
                n1345 = Index Array(array=w2266, index=w2265) -> (element=w2264:sgl)
              }
              frame Enabled {
                n1346 = local read "threatDetails"() -> (w2270:T1)
                n1347 = Unbundle By Name(w2270) -> ("dragCorrection"=w2268:string)
                n1348 = Not Equal?(x=w2268, y="") -> (x != y?=w2269:bool)
                n1349 = case shown="True" w2269 {
                  tunnel: [sgl 1.0 ("default value 1") w2274] -> w2271
                  tunnel: w2268 -> [_ w2273]
                  frame False {
                  }
                  frame True {
                    n1350 = Scan From String(input string=w2273, default 1=sgl 0.0 ("default value 1")) -> (output 1=w2274:sgl)  [unwired: 3 in, 3 out]
                  }
                }
              }
            }
            "correction coefficient" <- w2252
            n1351 = local read "Current/avg/speed"() -> (w2248:sgl)
            n1352 = local read "mid_to_targ_dist"() -> (w2249:sgl)
            n1353 = local read "lengthUnits"() -> (w2246:string)
            n1354 = call "Compute Strike Velocity.vi"("drag coefficient"=w2252, "decay distance"=w2249, "raw velocity"=w2248, "distance units"=w2246) -> ("correction factor"=w2226:sgl, "strike velocity"=w2250:sgl)  [unwired: 1 out]
            "DC_ factor" <- w2226
            "Corrected Average" <- w2250
            n1355 = call "Velocity Correction.vi"("raw impact"="MeasVelScrnSet1", "distance units"=w2246, "raw redundant"="MeasVelScrnSet2", "raw residual"="Current/residual/speed", "screen set midpt to target"="Set#1_to_Target", "residual screen to target"="Residual/Target Dist", "correction coefficient"=w2252) -> ("corrected impact"=w2257:sgl, "corrected redundant"=w2253:sgl, "corrected residual"=w2255:sgl, "impact factor"=w2244:sgl, "conversion factor"=→"conversion factor":sgl, "residual factor"=w2245:sgl)  [unwired: 3 out]
            "Residual factor" <- w2245
            "Impact factor" <- w2244
            "CorrectedVelScrnSet1" <- w2257
            "Corrected Residual" <- w2255
            "CorrectedVelScrnSet2" <- w2253
            n1356 = Select(t=w2253, s=w2247, f="MeasVelScrnSet2") -> (s? t:f=→"Redundant/speed":sgl)
            n1357 = Select(t=w2250, s=w2247, f=w2248) -> (s? t:f=→"Avg/speed":sgl)
            n1358 = Select(t=w2257, s=w2247, f="MeasVelScrnSet1") -> (s? t:f=→"Impact/speed":sgl)
            n1359 = Select(t=w2255, s=w2247, f="Current/residual/speed") -> (s? t:f=→"residual/speed":sgl)
            n1360 = Add(x="MeasVelScrnSet2", y="MeasVelScrnSet1") -> (x+y=w2230:sgl)
            n1361 = Subtract(x="MeasVelScrnSet2", y="MeasVelScrnSet1") -> (x-y=w2229:sgl)
            n1362 = Divide(x=w2230, y=sgl 200.0) -> (x/y=w2231:sgl)
            n1363 = Divide(x=w2229, y=w2231) -> (x/y=w2235:sgl)
            "%_Difference" <- w2235
            n1364 = Absolute Value(x=w2235) -> (abs(x)=w2237:sgl)
            n1365 = Less?(x=w2237, y="percent warning") -> (x < y?=w2242:bool)
            n1366 = Select(t=u32 65343, s=w2242, f=u32 15668992) -> (s? t:f=w2238:u32)
            n1367 = Select(t=u32 0, s=w2242, f=u32 16777226) -> (s? t:f=w2241:u32)
            n1368 = property on="%_Difference" class="DigNum (strict)"("Numeric Text.Text Colors:BG Color"=w2238, "NumText.TextColor"=w2241) -> ()  [unwired: 2 in, 2 out]
          }
          frame #1 {
            # "<-- DC_factor (for Average of impact and redundant)"
            # "IF drag corrected THEN apply factors"
            # "Residual factor"
            # "Impact factor\n(also applies to\nredundant velocity)"
            n1369 = for {
              tunnel: w2276 -> [w2292] mode=indexing
              tunnel: w2279 -> [w2301]
              tunnel: w2278 -> [w2296]
              tunnel: w2280 -> [w2290]
              tunnel: [w2303] -> w2281 mode=indexing
              tunnel: w2277 -> [w2286]
              n1370 = Unbundle By Name(w2292) -> ("UncorrectedAvgVel_PB"=w2291:sgl)
              n1371 = Unbundle By Name(w2292) -> ("UncorrectedRed_PB"=w2298:sgl)
              n1372 = Unbundle By Name(w2292) -> ("Uncorrected Impact"=w2295:sgl)
              n1373 = Unbundle By Name(w2292) -> ("Uncorrected Residual"=w2300:sgl)
              n1374 = Multiply(x=w2286, y=w2291) -> (x*y=w2288:sgl)
              n1375 = Multiply(x=w2296, y=w2298) -> (x*y=w2297:sgl)
              n1376 = Multiply(x=w2296, y=w2295) -> (x*y=w2287:sgl)
              n1377 = Multiply(x=w2301, y=w2300) -> (x*y=w2293:sgl)
              n1378 = Select(t=w2288, s=w2290, f=w2291) -> (s? t:f=w2289:sgl)
              n1379 = Select(t=w2297, s=w2290, f=w2298) -> (s? t:f=w2299:sgl)
              n1380 = Select(t=w2293, s=w2290, f=w2300) -> (s? t:f=w2302:sgl)
              n1381 = Select(t=w2287, s=w2290, f=w2295) -> (s? t:f=w2294:sgl)
              n1382 = Subtract(x=w2289, y=w2288) -> (x-y=w2283:sgl)
              n1383 = Not A Number/Path/Refnum?(number/path/refnum=w2283) -> (NaN/Path/Refnum?=w2285:bool)
              n1384 = Select(t=sgl 0.0, s=w2285, f=w2283) -> (s? t:f=w2282:sgl)
              n1385 = Bundle By Name(cluster=w2292, "velLoss_PB"=w2282, "strikeVel_PB"=w2288, "avgVel_PB"=w2289, "CorrectedRed_PB"=w2297, "Redundant_Velocity"=w2299, "Corrected Impact"=w2287, "IMPACT VELOCITY"=w2294, "Corrected residual"=w2293, "RESIDUAL  VELOCITY"=w2302) -> (w2303:T7)
            }
          }
          frame #2 {
            w2315 = sgl[] [] ("Partial")
            # "June 2012\n- Lucas Louriero requested \nstdev of velocities used in V50"
            # "This section calculates the V50"
            n1386 = for {
              shift-right: [w2339] -> w2317
              shift-left: w2315 -> [w2340]
              shift-right: [w2337] -> w2316
              shift-left: w2315 -> [w2338]
              tunnel: w2314 -> [w2331] mode=indexing
              n1387 = Unbundle By Name(w2331) -> ("SHOT STATUS"=w2336:u16)
              n1388 = Unbundle By Name(w2331) -> ("V50userExcl"=w2330:bool)
              n1389 = Unbundle By Name(w2331) -> ("IMPACT VELOCITY"=w2335:sgl)
              n1390 = Unbundle By Name(w2331) -> ("strikeVel_PB"=w2334:sgl)
              n1391 = Select(t=w2334, s="ScreenSetAvgg", f=w2335) -> (s? t:f=w2333:sgl)
              n1392 = case shown="False" w2330 {
                tunnel: w2340 -> [w2346 w2356]
                tunnel: [w2345 w2356] -> w2339
                tunnel: w2338 -> [w2344 w2355]
                tunnel: [w2343 w2355] -> w2337
                tunnel: w2336 -> [w2342 _]
                tunnel: w2333 -> [w2341 _]
                frame False {
                  n1393 = case shown="1" w2342 {
                    tunnel: w2341 -> [w2347 w2351]
                    tunnel: [w2350 w2352] -> w2345
                    tunnel: w2346 -> [w2349 w2352]
                    tunnel: w2344 -> [w2348 w2354]
                    tunnel: [w2348 w2353] -> w2343
                    frame 0, Default {
                      n1394 = Build Array (concatenate)(w2349, w2347) -> (w2350:sgl[])
                    }
                    frame 1 {
                      n1395 = Build Array (concatenate)(w2354, w2351) -> (w2353:sgl[])
                    }
                  }
                }
                frame True {
                }
              }
            }
            n1396 = Sort 1D Array(array=w2317) -> (sorted array=w2329:sgl[])
            n1397 = Sort 1D Array(array=w2316) -> (sorted array=w2322:sgl[])
            "Complete" <- w2322
            n1398 = Reverse 1D Array(array=w2329) -> (reversed array=w2320:sgl[])
            "Partial" <- w2320
            n1399 = Array Size(array=w2322) -> (size(s)=→"#_completes":i32)
            n1400 = Array Size(array=w2320) -> (size(s)=→"#_partials":i32)
            n1401 = Array Max & Min(array=w2320) -> (max value=w2326:sgl)  [unwired: 3 out]
            n1402 = Array Max & Min(array=w2322) -> (min value=w2324:sgl)  [unwired: 3 out]
            n1403 = call "Compute V50.vi"("Partial"=w2320, "Maximum Deviation"="maxDev", "Complete"=w2322) -> ("velSTDEV"=→"velSTDEV":sgl, "Pairs"=→"Pairs":i16, "zmr"=w2305:sgl, "V50"=→"computed_V50":sgl)  [unwired: 1 out]
            "Z.M.R." <- w2305
            n1404 = To Long Integer(number=w2326) -> (32bit integer=→"highPartial":i32)
            n1405 = To Long Integer(number=w2324) -> (32bit integer=→"lowComplete":i32)
            n1406 = Absolute Value(x=w2305) -> (abs(x)=→"zmr 2":sgl)
            n1407 = Less Than 0?(x=w2305) -> (x < 0?=w2308:bool)
            n1408 = Select(t="Low C minus High P", s=w2308, f="ZMR") -> (s? t:f=w2311:string)
            n1409 = Select(t=u32 65336, s=w2308, f=u32 16755266) -> (s? t:f=w2312:u32)
            n1410 = property on="zmr 2" class="DigNum (strict)"("Caption.Text"=w2311, "Numeric Text.Text Colors:BG Color"=w2312) -> ()  [unwired: 2 in, 2 out]
          }
          frame #3 {
            n1411 = local read "Pairs"() -> (w2369:i16)
            n1412 = Sort 1D Array(array=w2364) -> (sorted array=w2367:T7[])
            n1413 = for {
              tunnel: w2367 -> [w2417] mode=indexing
              tunnel: w2369 -> [w2427]
              shift-right: [w2426] -> _
              shift-left: i16 0 -> [w2425]
              tunnel: [w2419] -> w2365 mode=indexing
              # "this section marks the lowest completes that are used in V50"
              n1414 = Unbundle By Name(w2417) -> ("SHOT STATUS"=w2423:u16, "Projectile Mass"=w2421:sgl, "avgVel_PB"=w2420:sgl, "RESIDUAL  VELOCITY"=w2422:sgl)
              n1415 = Unbundle By Name(w2417) -> ("V50userExcl"=w2418:bool)
              n1416 = local read "conversion factor"() -> (w2428:sgl)
              n1417 = case shown="False" w2418 {
                tunnel: w2427 -> [w2439 _]
                tunnel: [w2438 w2448] -> w2426
                tunnel: w2425 -> [w2437 w2448]
                tunnel: [w2436 FALSE] -> w2424
                tunnel: w2423 -> [w2435 _]
                frame False {
                  n1418 = case shown="1" w2435 {
                    tunnel: w2439 -> [_ w2446]
                    tunnel: [FALSE w2445] -> w2436
                    tunnel: [w2441 w2444] -> w2438
                    tunnel: w2437 -> [w2441 w2442]
                    frame 0, Default {
                    }
                    frame 1 {
                      n1419 = Less?(x=w2442, y=w2446) -> (x < y?=w2445:bool)
                      n1420 = Add(x=w2442, y=i16 1 ("t")) -> (x+y=w2444:i16)
                    }
                  }
                }
                frame True {
                }
              }
              n1421 = Multiply(x=w2428, y=w2422) -> (x*y=w2429:sgl)
              n1422 = Multiply(x=w2420, y=w2428) -> (x*y=w2430:sgl)
              n1423 = Multiply(x=w2430, y=w2430) -> (x*y=w2434:sgl)
              n1424 = Multiply(x=w2429, y=w2429) -> (x*y=w2433:sgl)
              n1425 = Subtract(x=w2434, y=w2433) -> (x-y=w2432:sgl)
              n1426 = Compound Arithmetic op=MULTIPLY(w2421, w2432, sgl 0.0005 ("Input")) -> (w2415:sgl)
              n1427 = Not A Number/Path/Refnum?(number/path/refnum=w2415) -> (NaN/Path/Refnum?=w2416:bool)
              n1428 = Select(t=sgl 0.0, s=w2416, f=w2415) -> (s? t:f=w2413:sgl)
              n1429 = Bundle By Name(cluster=w2417, "usedv50"=w2424, "Energy Loss (J)"=w2413) -> (w2419:T7)
            }
            n1430 = Reverse 1D Array(array=w2365) -> (reversed array=w2366:T7[])
            n1431 = for {
              tunnel: w2366 -> [w2389] mode=indexing
              tunnel: w2369 -> [w2396]
              shift-right: [w2394] -> _
              shift-left: i16 0 -> [w2395]
              tunnel: [w2392] -> w2357 mode=indexing
              # "chooses highest partials used in v50"
              n1432 = Unbundle By Name(w2389) -> ("SHOT STATUS"=w2397:u16, "usedv50"=w2391:bool)
              n1433 = Unbundle By Name(w2389) -> ("V50userExcl"=w2390:bool)
              n1434 = case shown="False" w2390 {
                tunnel: w2397 -> [w2403 _]
                tunnel: w2396 -> [w2402 _]
                tunnel: w2395 -> [w2401 w2412]
                tunnel: [w2400 w2412] -> w2394
                tunnel: [w2399 FALSE ("usedv50")] -> w2393
                tunnel: w2391 -> [w2398 _]
                frame False {
                  n1435 = case shown="1" w2403 {
                    tunnel: w2402 -> [w2407 _]
                    tunnel: [w2406 w2410] -> w2399
                    tunnel: w2401 -> [w2404 w2409]
                    tunnel: [w2405 w2409] -> w2400
                    tunnel: w2398 -> [_ w2410]
                    frame 0, Default {
                      n1436 = Less?(x=w2404, y=w2407) -> (x < y?=w2406:bool)
                      n1437 = Add(x=w2404, y=i16 1) -> (x+y=w2405:i16)
                    }
                    frame 1 {
                    }
                  }
                }
                frame True {
                }
              }
              n1438 = Bundle By Name(cluster=w2389, "usedv50"=w2393) -> (w2392:T7)
            }
            n1439 = for {
              shift-right: [w2375] -> w2358
              shift-left: sgl[] [] ("Partial") -> [w2372]
              tunnel: w2357 -> [w2374] mode=indexing
              n1440 = local read "ScreenSetAvgg"() -> (w2379:bool)
              n1441 = Unbundle By Name(w2374) -> ("V50userExcl"=w2373:bool, "usedv50"=w2371:bool)
              n1442 = Unbundle By Name(w2374) -> ("IMPACT VELOCITY"=w2377:sgl)
              n1443 = Unbundle By Name(w2374) -> ("strikeVel_PB"=w2378:sgl)
              n1444 = Select(t=w2378, s=w2379, f=w2377) -> (s? t:f=w2376:sgl)
              n1445 = case shown="False" w2373 {
                tunnel: w2376 -> [w2380 _]
                tunnel: [w2381 w2388] -> w2375
                tunnel: w2372 -> [w2382 w2388]
                tunnel: w2371 -> [w2383 _]
                frame False {
                  n1446 = case shown="False" w2383 {
                    tunnel: w2382 -> [w2384 w2387]
                    tunnel: [w2384 w2386] -> w2381
                    tunnel: w2380 -> [_ w2385]
                    frame False {
                    }
                    frame True {
                      n1447 = Build Array (concatenate)(w2387, w2385) -> (w2386:sgl[])
                    }
                  }
                }
                frame True {
                }
              }
            }
            n1448 = Array Max & Min(array=w2358) -> (max value=w2363:sgl, min value=w2362:sgl)  [unwired: 2 out]
            n1449 = Subtract(x=w2363, y=w2362) -> (x-y=w2361:sgl)
            n1450 = property on="shotsArr" class="Arr (strict)"("Val(Sgnl)"=w2357) -> ()  [unwired: 2 in, 2 out]
            n1451 = To Long Integer(number=w2361) -> (32bit integer=→"rangeOfResults":i32)
          }
        }
      }
      frame "CHECK DAQ" {
        w2454 = 500  # timeout in ms
        # "case # 11"
        n1452 = Dequeue Element(queue=w2449, timeout in ms (-1)=w2454, error in (no error)=w2450) -> (element=w2453:dbl[], timed out?=w2452:bool, error out=w2451:errorcluster)  [unwired: 1 out]
        n1453 = case shown="True" w2452 {
          tunnel: [Collector_State."PROC SHOTS" ("progState") Collector_State."POLL" ("progState")] -> w2457
          tunnel: [-1 -1 ("index of element")] -> w2456
          tunnel: [w2466 w2510] -> w2455
          tunnel: w2451 -> [w2463 w2510]
          tunnel: w2453 -> [w2464 _]
          frame False {
            n1454 = local read "MeasSrc"() -> (w2465:T13)
            n1455 = case shown="\"Screens\"" w2465 {
              tunnel: w2463 -> [w2471 w2490 w2501]
              tunnel: [w2471 w2490 w2506] -> w2466
              tunnel: w2464 -> [_ _ w2505]
              tunnel: [w2470 w2489 w2492] -> w2461
              tunnel: [w2469 w2488 w2491] -> w2460
              frame "Simulated", Default {
                # "Simulated"
                n1456 = local read "minV50"() -> (w2475:i32)
                n1457 = local read "Powder Loading"() -> (w2487:sgl)
                n1458 = Wait (ms)(milliseconds to wait=u32 500 ("number")) -> ()  [unwired: 1 out]
                n1459 = To Single Precision Float(number=w2475) -> (single precision float=w2474:sgl)
                n1460 = call "Get Shell Speed.vi"("loading"=w2487, "v50"=w2474) -> ("impact"=w2470:sgl, "residual"=w2482:sgl)  [unwired: 1 in, 2 out]
                n1461 = Greater Than 0?(x=w2482) -> (x > 0?=w2484:bool)
                n1462 = local write "Current/residual/speed"(w2482) -> ()
                n1463 = Select(t=u16 1, s=w2484, f=u16 0) -> (s? t:f=w2483:u16)
                n1464 = local write "Current/shotstatus"(w2483) -> ()
                n1465 = Random Number (0-1)() -> (number: 0 to 1=w2480:dbl)
                n1466 = To Single Precision Float(number=w2480) -> (single precision float=w2476:sgl)
                n1467 = Multiply(x=w2476, y=sgl 0.002) -> (x*y=w2479:sgl)
                n1468 = local write "readyClock"(TRUE ("RANGE RESET")) -> ()
                n1469 = Add(x=w2479, y=sgl 0.999) -> (x+y=w2477:sgl)
                n1470 = Multiply(x=w2470, y=w2477) -> (x*y=w2469:sgl)
              }
              frame "Radar" {
                # "Radar -- (future)"
                n1471 = local read "MeasVelScrnSet1"() -> (w2489:sgl)
                n1472 = local read "MeasVelScrnSet2"() -> (w2488:sgl)
              }
              frame "Screens" {
                # "This section checks to see if the counters have been fired.  If they have then the counter times are read"
                n1473 = To Single Precision Float(number=w2505) -> (single precision float=w2504:sgl[])
                n1474 = Index Array(array=w2504) -> (element #1=w2500:sgl, element #2=w2499:sgl)  [unwired: 2 in]
                n1475 = Equal To 0?(x=w2500) -> (x = 0?=w2498:bool)
                n1476 = Equal To 0?(x=w2499) -> (x = 0?=w2494:bool)
                n1477 = local read "Set#1 Separation"() -> (w2503:sgl)
                n1478 = local read "Set#2 Separation"() -> (w2502:sgl)
                n1479 = Divide(x=w2503, y=w2500) -> (x/y=w2496:sgl)
                n1480 = Divide(x=w2502, y=w2499) -> (x/y=w2493:sgl)
                n1481 = Select(t=sgl 0.0, s=w2498, f=w2496) -> (s? t:f=w2492:sgl)
                n1482 = Select(t=sgl 0.0, s=w2494, f=w2493) -> (s? t:f=w2491:sgl)
                n1483 = case shown="No Error" w2501 {
                  selector: w2501 -> [w2509 _]
                  frame No Error {
                    # "=false"
                    n1484 = Unbundle By Name(w2509) -> ("status"=w2508:bool)
                    n1485 = Not(x=w2508) -> (.not. x?=w2507:bool)
                    n1486 = local write "readyClock"(w2507) -> ()
                  }
                  frame Error {
                  }
                }
                n1487 = call <vilib>:"Simple Error Handler.vi"("error in (no error)"=w2501) -> ("error out"=w2506:errorcluster)  [unwired: 1 in, 7 out]
              }
            }
            n1488 = control-ref of="2ndScreen"() -> (w2462:refnum<vi>)
            n1489 = call "2nd screen effect (SubVI).vi"("MeasVelScrnSet 2"=w2460, "MeasVelScrnSet 1"=w2461, "2nd Screen ref"=w2462) -> ("MeasVelOut"=→"Current/avg/speed":sgl)
            n1490 = local write "MeasVelScrnSet1"(w2461) -> ()
            n1491 = local write "MeasVelScrnSet2"(w2460) -> ()
          }
          frame True {
            # "timeout expired"
          }
        }
      }
    }
    "SMErr" <- w679
    "progState" <- w678
    n1492 = disable-structure shown="Enabled" {
      disable-tunnel: w679 -> [w688 _]
      disable-tunnel: w678 -> [w687 _]
      frame Disabled {
        n1493 = flat-sequence {
          tunnel: w687 -> [_]
          tunnel: w688 -> [_]
          frame #0 {
            n1494 = Wait (ms)(milliseconds to wait=u32 1) -> ()  [unwired: 1 out]
          }
          frame #1 {
            n1495 = property on="progState" class="Enum (strict)"() -> ("RingText.Text"=w693:string)  [unwired: 2 in, 2 out]
            n1496 = Get Date/Time In Seconds() -> (seconds since 1Jan1904=w691:timestamp)
            n1497 = Format Date/Time String(seconds (now)=w691) -> (date/time string=w690:string)  [unwired: 2 out]
            n1498 = Build Array(w690, "," ("element"), w693) -> (w694:string[])
            n1499 = call-poly <vilib>:"Write To Spreadsheet File.vi"("append to file? (new file:F)"=TRUE, "1D data"=w694, "file path (dialog if empty)"=path "C:/state.txt") -> ()  [unwired: 5 in, 1 out]
          }
        }
      }
      frame Enabled {
      }
    }
    n1500 = Wait (ms)(milliseconds to wait=u32 50 ("millisecond timer value")) -> ()  [unwired: 1 out]
  }
  n1501 = while "Arming Loop" {
    tunnel: w3 -> [w2537]
    shift-right: [w2535] -> w20
    shift-left: w21 -> [w2536]
    shift-right: [w2529] -> w11
    shift-left: w1 -> [w2533]
    shift-right: [w2530] -> w12
    shift-left: w2 -> [w2534]
    shift-right: [w2524] -> w13
    shift-left: w10 -> [w2532]
    shift-right: [w2523] -> w14
    shift-left: w9 -> [w2531]
    stop <- "close arming loop" stop-if-true
    w2527 = 10.0  # timeout
    # "error code -200474\ntimeout expired"
    n1502 = call-poly <vilib>:"DAQmx Read.vi"("task/channels in"=w2533, "timeout"=w2527, "error in"=w2531) -> ("task out"=w2529:refnum<k21>, "data"=w2525:dbl, "error out"=w2520:errorcluster)  [unwired: 10 in]
    n1503 = call-poly <vilib>:"DAQmx Read.vi"("task/channels in"=w2534, "timeout"=w2527, "error in"=w2532) -> ("task out"=w2530:refnum<k21>, "data"=w2526:dbl, "error out"=w2518:errorcluster)  [unwired: 10 in]
    n1504 = Unbundle By Name(w2518) -> ("code"=w2515:i32)
    n1505 = Unbundle By Name(w2520) -> ("code"=w2519:i32)
    n1506 = Equal?(x=w2515, y=-200474) -> (x = y?=w2514:bool)
    n1507 = Equal?(x=w2519, y=-200474) -> (x = y?=w2522:bool)
    n1508 = Or(x=w2514, y=w2522) -> (x .or. y?=w2517:bool)
    n1509 = case shown="False" w2517 {
      tunnel: w2537 -> [w2546 _]
      tunnel: w2536 -> [w2545 w2551]
      tunnel: [w2544 w2551] -> w2535
      tunnel: w2526 -> [w2542 _]
      tunnel: w2525 -> [w2541 _]
      frame False {
        n1510 = Build Array(w2542, w2541) -> (w2543:dbl[])
        n1511 = Enqueue Element(queue=w2546, element=w2543, error in (no error)=w2545) -> (queue out=w2539:refnum<queue>, error out=w2544:errorcluster)  [unwired: 1 in, 1 out]
        n1512 = for {
          N: 10 -> [w2549]
          tunnel: w2539 -> [_]
          i -> [w2548]
          n1513 = Subtract(x=w2549, y=w2548) -> (x-y=→"cntDn":i32)
          n1514 = Wait (ms)(milliseconds to wait=u32 1000) -> ()  [unwired: 1 out]
        }
        "ARMED" <- FALSE ("ARMED")
      }
      frame True {
      }
    }
    n1515 = local write "ARMED"(TRUE ("ARMED")) -> ()
    n1516 = case shown="No Error" w2518 {
      selector: w2518 -> [w2555 w2557]
      tunnel: [w2555 errorcluster {"status"=FALSE, "code"=0, "source"=""} ("error IO")] -> w2524
      frame No Error {
      }
      frame Error {
        "errCtr0" <- w2557
      }
    }
    n1517 = case shown="No Error" w2520 {
      selector: w2520 -> [w2552 w2554]
      tunnel: [w2552 errorcluster {"status"=FALSE, "code"=0, "source"=""} ("error IO")] -> w2523
      frame No Error {
      }
      frame Error {
        "errCtr1" <- w2554
      }
    }
  }
  n1518 = call <vilib>:"DAQmx Clear Task.vi"("task in"=w11, "error in"=w14) -> ("error out"=w17:errorcluster)  [unwired: 13 in]
  n1519 = call <vilib>:"DAQmx Clear Task.vi"("task in"=w12, "error in"=w13) -> ("error out"=w18:errorcluster)  [unwired: 13 in]
  n1520 = Release Queue(queue=w3, force destroy? (F)=TRUE, error in (no error)=w20) -> (error out=w15:errorcluster)  [unwired: 2 out]
  n1521 = Merge Errors(w18, w17, w15) -> (w19:errorcluster)
  n1522 = call <vilib>:"General Error Handler.vi"("type of dialog (OK msg:1)"=w16, "error in (no error)"=w19) -> ()  [unwired: 9 in, 5 out]
